vi "LCM_data_assign.vi"(9 "time-to-live":u16, 10 "Velodyne1":T2(ring), 11 "velodyne enable":bool) -> ()   [LabVIEW 2015]
uses:
  G_LCM.vi
  G_ALL.vi
  G_SEN.vi
  <vilib>/Instr/_visa.llb/VISA Configure Serial Port (Instr).vi
panel:
  out "error out 3":errorcluster
  out "velodyne overflow? 2":bool
  out "VELO_RAW":T1={"hash"=6418264790525055119, "sys time"=0, "type"=0, "raw"=""} {"hash" format="%x"}
  out "ibeo overflow?":bool
  out "veodyne error out":errorcluster
  out "control input":T3
  in  "saveconfig":bool
  in  "get data":bool
  in  "parameter idx 2":u16 format="%x"
  in  "setdata":bool
  in  "Mouting":u32 format="%x"
  in  "parameter idx":u16 format="%x"
  out "LCM error":errorcluster
  out "error out":errorcluster
  out "SDT_GPS_DATA":T4
  out "PATH_T":T5
  out "length":i32
  out "ALT_T":T6={"hash"=-8920902524919788889, "sys time"=0, "u time"=0, "alt"=0.0} {"hash" format="%016x"}
  out "value":cluster{"time":i32, "alt":sgl}
  out "data":dbl[][](array[numeric]) format="%#_17g"
  out "Waveform Graph":dbl[](graph)
  out "IBEO_2202_T":T7={"hash"=-9184050406206942030, "sys time"=0, "Header"={"Size of prev messages"=0, "Size of this messages"=8534, "Reserved"=0, "DeviceID"=0, "Data type"=8706, "NTP time"=30358766255088}, "Scan header"={"Scan number"=22632, "scanner status"=811, "Sync phase offset"=0, "Scan start time NTP"=30358508796168, "Scan end time NTP"=30358603880928, "Angle ticks per rotation"=11520, "Start angle"=0.8726646259971648, "End angle"=-0.8726646259971648, "Scan points"=849, "pos_x"=0.0, "pos_y"=0.0, "pos_h"=0.0, "Mounting position x"=3.5, "Mounting position y"=0.0, "Mounting position z"=0.45, "Reserved"=5}, "Scan points"=[{"flags"=0, "Echo"=0, "Radial distance"=20.2, "Horizontal angle"=0.8552113334772213, "Vertical angle"=-0.020943951023931952, "Echo pulse width"=92, "Reserved"=0}, {"flags"=0, "Echo"=0, "Radial distance"=20.05, "Horizontal angle"=0.8552113334772213, "Vertical angle"=-0.006981317007977317, "Echo pulse width"=48, "Reserved"=0}, {"flags"=0, "Echo"=0, "Radial distance"=20.21, "Horizontal angle"=0.8464846872172498, "Vertical angle"=-0.020943951023931952, "Echo pulse width"=80, "Reserved"=0}, {"flags"=0, "Echo"=0, "Radial distance"=20.03, "Horizontal angle"=0.8464846872172498, "Vertical angle"=-0.006981317007977317, "Echo pulse width"=120, "Reserved"=0}, {"flags"=0, "Echo"=0, "Radial distance"=20.400000000000002, "Horizontal angle"=0.8377580409572781, "Vertical angle"=-0.020943951023931952, "Echo pulse width"=136, "Reserved"=0}, {"flags"=0, "Echo"=0, "Radial distance"=20.080000000000002, "Horizontal angle"=0.8377580409572781, "Vertical angle"=-0.006981317007977317, "Echo pulse width"=132, "Reserved"=0}, {"flags"=0, "Echo"=0, "Radial distance"=20.67, "Horizontal angle"=0.8290313946973066, "Vertical angle"=-0.020943951023931952, "Echo pulse width"=124, "Reserved"=0}, {"flags"=0, "Echo"=0, "Radial distance"=20.37, "Horizontal angle"=0.8290313946973066, "Vertical angle"=-0.006981317007977317, "Echo pulse width"=144, "Reserved"=0}, {"flags"=5, "Echo"=0, "Radial distance"=20.830000000000002, "Horizontal angle"=0.8203047484373349, "Vertical angle"=-0.020943951023931952, "Echo pulse width"=72, "Reserved"=0}, {"flags"=4, "Echo"=1, "Radial distance"=21.87, "Horizontal angle"=0.8203047484373349, "Vertical angle"=-0.020943951023931952, "Echo pulse width"=124, "Reserved"=0}, {"flags"=4, "Echo"=0, "Radial distance"=21.88, "Horizontal angle"=0.8115781021773633, "Vertical angle"=-0.020943951023931952, "Echo pulse width"=132, "Reserved"=0}, {"flags"=4, "Echo"=0, "Radial distance"=21.78, "Horizontal angle"=0.8028514559173915, "Vertical angle"=-0.020943951023931952, "Echo pulse width"=156, "Reserved"=0}, {"flags"=4, "Echo"=0, "Radial distance"=21.76, "Horizontal angle"=0.7941248096574199, "Vertical angle"=-0.020943951023931952, "Echo pulse width"=176, "Reserved"=0}, {"flags"=1, "Echo"=0, "Radial distance"=23.37, "Horizontal angle"=0.7941248096574199, "Vertical angle"=-0.006981317007977317, "Echo pulse width"=100, "Reserved"=1}, {"flags"=0, "Echo"=1, "Radial distance"=48.230000000000004, "Horizontal angle"=0.7941248096574199, "Vertical angle"=-0.006981317007977317, "Echo pulse width"=120, "Reserved"=2}, {"flags"=4, "Echo"=0, "Radial distance"=21.76, "Horizontal angle"=0.7853981633974483, "Vertical angle"=-0.020943951023931952, "Echo pulse width"=172, "Reserved"=0}, {"flags"=1, "Echo"=0, "Radial distance"=23.25, "Horizontal angle"=0.7853981633974483, "Vertical angle"=-0.006981317007977317, "Echo pulse width"=144, "Reserved"=1}, {"flags"=0, "Echo"=1, "Radial distance"=48.02, "Horizontal angle"=0.7853981633974483, "Vertical angle"=-0.006981317007977317, "Echo pulse width"=108, "Reserved"=2}, {"flags"=0, "Echo"=0, "Radial distance"=16.740000000000002, "Horizontal angle"=0.7766715171374766, "Vertical angle"=-0.020943951023931952, "Echo pulse width"=156, "Reserved"=3}, {"flags"=0, "Echo"=0, "Radial distance"=16.77, "Horizontal angle"=0.7766715171374766, "Vertical angle"=-0.006981317007977317, "Echo pulse width"=152, "Reserved"=3}, {"flags"=5, "Echo"=0, "Radial distance"=5.44, "Horizontal angle"=0.767944870877505, "Vertical angle"=-0.020943951023931952, "Echo pulse width"=136, "Reserved"=0}, {"flags"=4, "Echo"=1, "Radial distance"=21.87, "Horizontal angle"=0.767944870877505, "Vertical angle"=-0.020943951023931952, "Echo pulse width"=164, "Reserved"=0}, {"flags"=1, "Echo"=0, "Radial distance"=23.17, "Horizontal angle"=0.767944870877505, "Vertical angle"=-0.006981317007977317, "Echo pulse width"=148, "Reserved"=1}, {"flags"=0, "Echo"=1, "Radial distance"=48.18, "Horizontal angle"=0.767944870877505, "Vertical angle"=-0.006981317007977317, "Echo pulse width"=108, "Reserved"=4}, {"flags"=4, "Echo"=0, "Radial distance"=22.03, "Horizontal angle"=0.7592182246175333, "Vertical angle"=-0.020943951023931952, "Echo pulse width"=164, "Reserved"=0}, {"flags"=0, "Echo"=0, "Radial distance"=23.3, "Horizontal angle"=0.7592182246175333, "Vertical angle"=-0.006981317007977317, "Echo pulse width"=168, "Reserved"=1}, {"flags"=5, "Echo"=0, "Radial distance"=5.21, "Horizontal angle"=0.7504915783575618, "Vertical angle"=-0.020943951023931952, "Echo pulse width"=144, "Reserved"=0}, {"flags"=4, "Echo"=1, "Radial distance"=22.27, "Horizontal angle"=0.7504915783575618, "Vertical angle"=-0.020943951023931952, "Echo pulse width"=164, "Reserved"=0}, {"flags"=0, "Echo"=0, "Radial distance"=23.34, "Horizontal angle"=0.7504915783575618, "Vertical angle"=-0.006981317007977317, "Echo pulse width"=172, "Reserved"=1}, {"flags"=5, "Echo"=0, "Radial distance"=20.36, "Horizontal angle"=0.74176493209759, "Vertical angle"=-0.020943951023931952, "Echo pulse width"=68, "Reserved"=0}, {"flags"=4, "Echo"=1, "Radial distance"=22.42, "Horizontal angle"=0.74176493209759, "Vertical angle"=-0.020943951023931952, "Echo pulse width"=152, "Reserved"=0}, {"flags"=0, "Echo"=0, "Radial distance"=23.38, "Horizontal angle"=0.74176493209759, "Vertical angle"=-0.006981317007977317, "Echo pulse width"=168, "Reserved"=1}, {"flags"=5, "Echo"=0, "Radial distance"=5.5600000000000005, "Horizontal angle"=0.7330382858376184, "Vertical angle"=-0.020943951023931952, "Echo pulse width"=168, "Reserved"=0}, {"flags"=4, "Echo"=1, "Radial distance"=22.62, "Horizontal angle"=0.7330382858376184, "Vertical angle"=-0.020943951023931952, "Echo pulse width"=152, "Reserved"=0}, {"flags"=1, "Echo"=0, "Radial distance"=23.37, "Horizontal angle"=0.7330382858376184, "Vertical angle"=-0.006981317007977317, "Echo pulse width"=156, "Reserved"=1}, {"flags"=0, "Echo"=1, "Radial distance"=48.21, "Horizontal angle"=0.7330382858376184, "Vertical angle"=-0.006981317007977317, "Echo pulse width"=72, "Reserved"=5}, {"flags"=5, "Echo"=0, "Radial distance"=5.58, "Horizontal angle"=0.7243116395776468, "Vertical angle"=-0.020943951023931952, "Echo pulse width"=136, "Reserved"=0}, {"flags"=5, "Echo"=1, "Radial distance"=20.88, "Horizontal angle"=0.7243116395776468, "Vertical angle"=-0.020943951023931952, "Echo pulse width"=64, "Reserved"=0}, {"flags"=4, "Echo"=2, "Radial distance"=22.77, "Horizontal angle"=0.7243116395776468, "Vertical angle"=-0.020943951023931952, "Echo pulse width"=148, "Reserved"=0}, {"flags"=0, "Echo"=0, "Radial distance"=23.62, "Horizontal angle"=0.7243116395776468, "Vertical angle"=-0.006981317007977317, "Echo pulse width"=172, "Reserved"=1}, {"flags"=5, "Echo"=0, "Radial distance"=5.63, "Horizontal angle"=0.7155849933176751, "Vertical angle"=-0.020943951023931952, "Echo pulse width"=196, "Reserved"=0}, {"flags"=4, "Echo"=1, "Radial distance"=22.69, "Horizontal angle"=0.7155849933176751, "Vertical angle"=-0.020943951023931952, "Echo pulse width"=212, "Reserved"=0}, {"flags"=0, "Echo"=0, "Radial distance"=23.82, "Horizontal angle"=0.7155849933176751, "Vertical angle"=-0.006981317007977317, "Echo pulse width"=160, "Reserved"=1}, {"flags"=5, "Echo"=0, "Radial distance"=5.67, "Horizontal angle"=0.7068583470577035, "Vertical angle"=-0.020943951023931952, "Echo pulse width"=172, "Reserved"=0}, {"flags"=4, "Echo"=1, "Radial distance"=23.16, "Horizontal angle"=0.7068583470577035, "Vertical angle"=-0.020943951023931952, "Echo pulse width"=176, "Reserved"=0}, {"flags"=0, "Echo"=0, "Radial distance"=23.62, "Horizontal angle"=0.7068583470577035, "Vertical angle"=-0.006981317007977317, "Echo pulse width"=164, "Reserved"=1}, {"flags"=5, "Echo"=0, "Radial distance"=5.53, "Horizontal angle"=0.6981317007977318, "Vertical angle"=-0.020943951023931952, "Echo pulse width"=208, "Reserved"=0}, {"flags"=0, "Echo"=1, "Radial distance"=23.35, "Horizontal angle"=0.6981317007977318, "Vertical angle"=-0.020943951023931952, "Echo pulse width"=160, "Reserved"=1}, {"flags"=0, "Echo"=0, "Radial distance"=23.650000000000002, "Horizontal angle"=0.6981317007977318, "Vertical angle"=-0.006981317007977317, "Echo pulse width"=148, "Reserved"=1}, {"flags"=5, "Echo"=0, "Radial distance"=5.55, "Horizontal angle"=0.6894050545377601, "Vertical angle"=-0.020943951023931952, "Echo pulse width"=192, "Reserved"=0}, {"flags"=0, "Echo"=1, "Radial distance"=23.55, "Horizontal angle"=0.6894050545377601, "Vertical angle"=-0.020943951023931952, "Echo pulse width"=160, "Reserved"=1}, {"flags"=0, "Echo"=0, "Radial distance"=23.62, "Horizontal angle"=0.6894050545377601, "Vertical angle"=-0.006981317007977317, "Echo pulse width"=160, "Reserved"=1}, {"flags"=5, "Echo"=0, "Radial distance"=5.5600000000000005, "Horizontal angle"=0.6806784082777886, "Vertical angle"=-0.020943951023931952, "Echo pulse width"=236, "Reserved"=0}, {"flags"=0, "Echo"=1, "Radial distance"=23.77, "Horizontal angle"=0.6806784082777886, "Vertical angle"=-0.020943951023931952, "Echo pulse width"=144, "Reserved"=1}, {"flags"=0, "Echo"=0, "Radial distance"=23.61, "Horizontal angle"=0.6806784082777886, "Vertical angle"=-0.006981317007977317, "Echo pulse width"=156, "Reserved"=1}, {"flags"=5, "Echo"=0, "Radial distance"=5.5200000000000005, "Horizontal angle"=0.6719517620178168, "Vertical angle"=-0.020943951023931952, "Echo pulse width"=220, "Reserved"=0}, {"flags"=4, "Echo"=1, "Radial distance"=24.17, "Horizontal angle"=0.6719517620178168, "Vertical angle"=-0.020943951023931952, "Echo pulse width"=148, "Reserved"=0}, {"flags"=0, "Echo"=0, "Radial distance"=23.66, "Horizontal angle"=0.6719517620178168, "Vertical angle"=-0.006981317007977317, "Echo pulse width"=164, "Reserved"=1}, {"flags"=5, "Echo"=0, "Radial distance"=5.67, "Horizontal angle"=0.6632251157578453, "Vertical angle"=-0.020943951023931952, "Echo pulse width"=224, "Reserved"=0}, {"flags"=4, "Echo"=1, "Radial distance"=24.45, "Horizontal angle"=0.6632251157578453, "Vertical angle"=-0.020943951023931952, "Echo pulse width"=148, "Reserved"=0}, {"flags"=1, "Echo"=0, "Radial distance"=32.230000000000004, "Horizontal angle"=0.6632251157578453, "Vertical angle"=-0.006981317007977317, "Echo pulse width"=40, "Reserved"=6}, {"flags"=0, "Echo"=1, "Radial distance"=35.42, "Horizontal angle"=0.6632251157578453, "Vertical angle"=-0.006981317007977317, "Echo pulse width"=164, "Reserved"=7}, {"flags"=5, "Echo"=0, "Radial distance"=5.63, "Horizontal angle"=0.6544984694978736, "Vertical angle"=-0.020943951023931952, "Echo pulse width"=208, "Reserved"=0}, {"flags"=4, "Echo"=1, "Radial distance"=24.73, "Horizontal angle"=0.6544984694978736, "Vertical angle"=-0.020943951023931952, "Echo pulse width"=144, "Reserved"=0}, {"flags"=0, "Echo"=0, "Radial distance"=35.14, "Horizontal angle"=0.6544984694978736, "Vertical angle"=-0.006981317007977317, "Echo pulse width"=164, "Reserved"=7}, {"flags"=5, "Echo"=0, "Radial distance"=5.64, "Horizontal angle"=0.6457718232379019, "Vertical angle"=-0.020943951023931952, "Echo pulse width"=244, "Reserved"=0}, {"flags"=4, "Echo"=1, "Radial distance"=25.04, "Horizontal angle"=0.6457718232379019, "Vertical angle"=-0.020943951023931952, "Echo pulse width"=132, "Reserved"=0}, {"flags"=0, "Echo"=0, "Radial distance"=35.01, "Horizontal angle"=0.6457718232379019, "Vertical angle"=-0.006981317007977317, "Echo pulse width"=156, "Reserved"=7}, {"flags"=5, "Echo"=0, "Radial distance"=5.71, "Horizontal angle"=0.6370451769779303, "Vertical angle"=-0.020943951023931952, "Echo pulse width"=264, "Reserved"=0}, {"flags"=4, "Echo"=1, "Radial distance"=25.6, "Horizontal angle"=0.6370451769779303, "Vertical angle"=-0.020943951023931952, "Echo pulse width"=132, "Reserved"=0}, {"flags"=1, "Echo"=0, "Radial distance"=32.68, "Horizontal angle"=0.6370451769779303, "Vertical angle"=-0.006981317007977317, "Echo pulse width"=56, "Reserved"=8}, {"flags"=0, "Echo"=1, "Radial distance"=34.86, "Horizontal angle"=0.6370451769779303, "Vertical angle"=-0.006981317007977317, "Echo pulse width"=160, "Reserved"=7}, {"flags"=5, "Echo"=0, "Radial distance"=5.63, "Horizontal angle"=0.6283185307179586, "Vertical angle"=-0.020943951023931952, "Echo pulse width"=296, "Reserved"=0}, {"flags"=4, "Echo"=1, "Radial distance"=25.84, "Horizontal angle"=0.6283185307179586, "Vertical angle"=-0.020943951023931952, "Echo pulse width"=92, "Reserved"=0}, {"flags"=5, "Echo"=0, "Radial distance"=7.54, "Horizontal angle"=0.6283185307179586, "Vertical angle"=-0.006981317007977317, "Echo pulse width"=168, "Reserved"=0}, {"flags"=0, "Echo"=1, "Radial distance"=34.87, "Horizontal angle"=0.6283185307179586, "Vertical angle"=-0.006981317007977317, "Echo pulse width"=124, "Reserved"=7}, {"flags"=4, "Echo"=0, "Radial distance"=5.67, "Horizontal angle"=0.619591884457987, "Vertical angle"=-0.020943951023931952, "Echo pulse width"=272, "Reserved"=0}, {"flags"=4, "Echo"=0, "Radial distance"=7.38, "Horizontal angle"=0.619591884457987, "Vertical angle"=-0.006981317007977317, "Echo pulse width"=204, "Reserved"=0}, {"flags"=4, "Echo"=0, "Radial distance"=5.67, "Horizontal angle"=0.6108652381980153, "Vertical angle"=-0.020943951023931952, "Echo pulse width"=284, "Reserved"=0}, {"flags"=0, "Echo"=0, "Radial distance"=7.33, "Horizontal angle"=0.6108652381980153, "Vertical angle"=-0.006981317007977317, "Echo pulse width"=224, "Reserved"=9}, {"flags"=0, "Echo"=0, "Radial distance"=7.21, "Horizontal angle"=0.6065019150680295, "Vertical angle"=0.00698131700797732, "Echo pulse width"=124, "Reserved"=9}, {"flags"=0, "Echo"=0, "Radial distance"=7.08, "Horizontal angle"=0.6065019150680295, "Vertical angle"=0.020943951023931963, "Echo pulse width"=120, "Reserved"=9}, {"flags"=4, "Echo"=0, "Radial distance"=5.79, "Horizontal angle"=0.6021385919380438, "Vertical angle"=-0.020943951023931952, "Echo pulse width"=248, "Reserved"=0}, {"flags"=0, "Echo"=0, "Radial distance"=7.09, "Horizontal angle"=0.6021385919380438, "Vertical angle"=-0.006981317007977317, "Echo pulse width"=232, "Reserved"=9}, {"flags"=0, "Echo"=0, "Radial distance"=7.24, "Horizontal angle"=0.5977752688080579, "Vertical angle"=0.00698131700797732, "Echo pulse width"=72, "Reserved"=9}, {"flags"=0, "Echo"=0, "Radial distance"=6.99, "Horizontal angle"=0.5977752688080579, "Vertical angle"=0.020943951023931963, "Echo pulse width"=60, "Reserved"=9}, {"flags"=4, "Echo"=0, "Radial distance"=5.75, "Horizontal angle"=0.593411945678072, "Vertical angle"=-0.020943951023931952, "Echo pulse width"=268, "Reserved"=0}, {"flags"=0, "Echo"=0, "Radial distance"=6.84, "Horizontal angle"=0.593411945678072, "Vertical angle"=-0.006981317007977317, "Echo pulse width"=284, "Reserved"=9}, {"flags"=0, "Echo"=0, "Radial distance"=7.140000000000001, "Horizontal angle"=0.5890486225480862, "Vertical angle"=0.00698131700797732, "Echo pulse width"=160, "Reserved"=9}, {"flags"=0, "Echo"=0, "Radial distance"=6.98, "Horizontal angle"=0.5890486225480862, "Vertical angle"=0.020943951023931963, "Echo pulse width"=144, "Reserved"=9}, {"flags"=4, "Echo"=0, "Radial distance"=5.79, "Horizontal angle"=0.5846852994181004, "Vertical angle"=-0.020943951023931952, "Echo pulse width"=236, "Reserved"=0}, {"flags"=0, "Echo"=0, "Radial distance"=6.95, "Horizontal angle"=0.5846852994181004, "Vertical angle"=-0.006981317007977317, "Echo pulse width"=264, "Reserved"=9}, {"flags"=0, "Echo"=0, "Radial distance"=7.03, "Horizontal angle"=0.5803219762881145, "Vertical angle"=0.00698131700797732, "Echo pulse width"=112, "Reserved"=9}, {"flags"=0, "Echo"=0, "Radial distance"=6.8, "Horizontal angle"=0.5803219762881145, "Vertical angle"=0.020943951023931963, "Echo pulse width"=104, "Reserved"=9}, {"flags"=4, "Echo"=0, "Radial distance"=5.67, "Horizontal angle"=0.5759586531581287, "Vertical angle"=-0.020943951023931952, "Echo pulse width"=268, "Reserved"=0}, {"flags"=0, "Echo"=0, "Radial distance"=6.76, "Horizontal angle"=0.5759586531581287, "Vertical angle"=-0.006981317007977317, "Echo pulse width"=288, "Reserved"=9}, {"flags"=0, "Echo"=0, "Radial distance"=7.0200000000000005, "Horizontal angle"=0.5715953300281429, "Vertical angle"=0.00698131700797732, "Echo pulse width"=168, "Reserved"=9}, {"flags"=0, "Echo"=0, "Radial distance"=6.91, "Horizontal angle"=0.5715953300281429, "Vertical angle"=0.020943951023931963, "Echo pulse width"=156, "Reserved"=9}, {"flags"=4, "Echo"=0, "Radial distance"=5.76, "Horizontal angle"=0.5672320068981571, "Vertical angle"=-0.020943951023931952, "Echo pulse width"=216, "Reserved"=0}, {"flags"=0, "Echo"=0, "Radial distance"=6.71, "Horizontal angle"=0.5672320068981571, "Vertical angle"=-0.006981317007977317, "Echo pulse width"=264, "Reserved"=9}, {"flags"=0, "Echo"=0, "Radial distance"=7.08, "Horizontal angle"=0.5628686837681712, "Vertical angle"=0.00698131700797732, "Echo pulse width"=136, "Reserved"=9}, {"flags"=0, "Echo"=0, "Radial distance"=6.8100000000000005, "Horizontal angle"=0.5628686837681712, "Vertical angle"=0.020943951023931963, "Echo pulse width"=112, "Reserved"=9}, {"flags"=4, "Echo"=0, "Radial distance"=5.79, "Horizontal angle"=0.5585053606381855, "Vertical angle"=-0.020943951023931952, "Echo pulse width"=248, "Reserved"=0}, {"flags"=0, "Echo"=0, "Radial distance"=6.6000000000000005, "Horizontal angle"=0.5585053606381855, "Vertical angle"=-0.006981317007977317, "Echo pulse width"=256, "Reserved"=9}, {"flags"=0, "Echo"=0, "Radial distance"=6.95, "Horizontal angle"=0.5541420375081997, "Vertical angle"=0.00698131700797732, "Echo pulse width"=176, "Reserved"=9}, {"flags"=0, "Echo"=0, "Radial distance"=6.75, "Horizontal angle"=0.5541420375081997, "Vertical angle"=0.020943951023931963, "Echo pulse width"=160, "Reserved"=9}, {"flags"=4, "Echo"=0, "Radial distance"=5.8100000000000005, "Horizontal angle"=0.5497787143782138, "Vertical angle"=-0.020943951023931952, "Echo pulse width"=204, "Reserved"=0}, {"flags"=0, "Echo"=0, "Radial distance"=6.61, "Horizontal angle"=0.5497787143782138, "Vertical angle"=-0.006981317007977317, "Echo pulse width"=224, "Reserved"=9}, {"flags"=0, "Echo"=0, "Radial distance"=6.88, "Horizontal angle"=0.5454153912482279, "Vertical angle"=0.00698131700797732, "Echo pulse width"=140, "Reserved"=9}, {"flags"=0, "Echo"=0, "Radial distance"=6.65, "Horizontal angle"=0.5454153912482279, "Vertical angle"=0.020943951023931963, "Echo pulse width"=124, "Reserved"=9}, {"flags"=4, "Echo"=0, "Radial distance"=5.8, "Horizontal angle"=0.5410520681182421, "Vertical angle"=-0.020943951023931952, "Echo pulse width"=232, "Reserved"=0}, {"flags"=0, "Echo"=0, "Radial distance"=6.65, "Horizontal angle"=0.5410520681182421, "Vertical angle"=-0.006981317007977317, "Echo pulse width"=232, "Reserved"=9}, {"flags"=0, "Echo"=0, "Radial distance"=6.91, "Horizontal angle"=0.5366887449882564, "Vertical angle"=0.00698131700797732, "Echo pulse width"=192, "Reserved"=9}, {"flags"=0, "Echo"=0, "Radial distance"=6.67, "Horizontal angle"=0.5366887449882564, "Vertical angle"=0.020943951023931963, "Echo pulse width"=160, "Reserved"=9}, {"flags"=4, "Echo"=0, "Radial distance"=5.91, "Horizontal angle"=0.5323254218582705, "Vertical angle"=-0.020943951023931952, "Echo pulse width"=196, "Reserved"=0}, {"flags"=0, "Echo"=0, "Radial distance"=6.7, "Horizontal angle"=0.5323254218582705, "Vertical angle"=-0.006981317007977317, "Echo pulse width"=200, "Reserved"=9}, {"flags"=0, "Echo"=0, "Radial distance"=6.72, "Horizontal angle"=0.5279620987282847, "Vertical angle"=0.00698131700797732, "Echo pulse width"=136, "Reserved"=9}, {"flags"=0, "Echo"=0, "Radial distance"=6.66, "Horizontal angle"=0.5279620987282847, "Vertical angle"=0.020943951023931963, "Echo pulse width"=144, "Reserved"=9}, {"flags"=4, "Echo"=0, "Radial distance"=5.91, "Horizontal angle"=0.5235987755982988, "Vertical angle"=-0.020943951023931952, "Echo pulse width"=224, "Reserved"=0}, {"flags"=0, "Echo"=0, "Radial distance"=6.72, "Horizontal angle"=0.5235987755982988, "Vertical angle"=-0.006981317007977317, "Echo pulse width"=220, "Reserved"=9}, {"flags"=0, "Echo"=0, "Radial distance"=6.87, "Horizontal angle"=0.519235452468313, "Vertical angle"=0.00698131700797732, "Echo pulse width"=180, "Reserved"=9}, {"flags"=0, "Echo"=0, "Radial distance"=6.68, "Horizontal angle"=0.519235452468313, "Vertical angle"=0.020943951023931963, "Echo pulse width"=180, "Reserved"=9}, {"flags"=4, "Echo"=0, "Radial distance"=6.03, "Horizontal angle"=0.5148721293383272, "Vertical angle"=-0.020943951023931952, "Echo pulse width"=192, "Reserved"=0}, {"flags"=0, "Echo"=0, "Radial distance"=6.68, "Horizontal angle"=0.5148721293383272, "Vertical angle"=-0.006981317007977317, "Echo pulse width"=208, "Reserved"=9}, {"flags"=0, "Echo"=0, "Radial distance"=7.01, "Horizontal angle"=0.5105088062083414, "Vertical angle"=0.00698131700797732, "Echo pulse width"=176, "Reserved"=9}, {"flags"=0, "Echo"=0, "Radial distance"=6.62, "Horizontal angle"=0.5105088062083414, "Vertical angle"=0.020943951023931963, "Echo pulse width"=148, "Reserved"=9}, {"flags"=4, "Echo"=0, "Radial distance"=5.99, "Horizontal angle"=0.5061454830783556, "Vertical angle"=-0.020943951023931952, "Echo pulse width"=216, "Reserved"=0}, {"flags"=0, "Echo"=0, "Radial distance"=6.6000000000000005, "Horizontal angle"=0.5061454830783556, "Vertical angle"=-0.006981317007977317, "Echo pulse width"=220, "Reserved"=9}, {"flags"=0, "Echo"=0, "Radial distance"=6.82, "Horizontal angle"=0.5017821599483697, "Vertical angle"=0.00698131700797732, "Echo pulse width"=200, "Reserved"=9}, {"flags"=0, "Echo"=0, "Radial distance"=6.640000000000001, "Horizontal angle"=0.5017821599483697, "Vertical angle"=0.020943951023931963, "Echo pulse width"=180, "Reserved"=9}, {"flags"=4, "Echo"=0, "Radial distance"=6.09, "Horizontal angle"=0.4974188368183839, "Vertical angle"=-0.020943951023931952, "Echo pulse width"=188, "Reserved"=0}, {"flags"=0, "Echo"=0, "Radial distance"=6.66, "Horizontal angle"=0.4974188368183839, "Vertical angle"=-0.006981317007977317, "Echo pulse width"=204, "Reserved"=9}, {"flags"=0, "Echo"=0, "Radial distance"=6.79, "Horizontal angle"=0.49305551368839806, "Vertical angle"=0.00698131700797732, "Echo pulse width"=160, "Reserved"=9}, {"flags"=0, "Echo"=0, "Radial distance"=6.59, "Horizontal angle"=0.49305551368839806, "Vertical angle"=0.020943951023931963, "Echo pulse width"=160, "Reserved"=9}, {"flags"=4, "Echo"=0, "Radial distance"=6.15, "Horizontal angle"=0.4886921905584123, "Vertical angle"=-0.020943951023931952, "Echo pulse width"=216, "Reserved"=0}, {"flags"=0, "Echo"=0, "Radial distance"=6.71, "Horizontal angle"=0.4886921905584123, "Vertical angle"=-0.006981317007977317, "Echo pulse width"=200, "Reserved"=9}, {"flags"=0, "Echo"=0, "Radial distance"=6.6000000000000005, "Horizontal angle"=0.48432886742842646, "Vertical angle"=0.00698131700797732, "Echo pulse width"=184, "Reserved"=9}, {"flags"=0, "Echo"=0, "Radial distance"=6.5200000000000005, "Horizontal angle"=0.48432886742842646, "Vertical angle"=0.020943951023931963, "Echo pulse width"=176, "Reserved"=9}, {"flags"=4, "Echo"=0, "Radial distance"=6.15, "Horizontal angle"=0.4799655442984406, "Vertical angle"=-0.020943951023931952, "Echo pulse width"=196, "Reserved"=0}, {"flags"=0, "Echo"=0, "Radial distance"=6.72, "Horizontal angle"=0.4799655442984406, "Vertical angle"=-0.006981317007977317, "Echo pulse width"=184, "Reserved"=9}, {"flags"=0, "Echo"=0, "Radial distance"=6.71, "Horizontal angle"=0.47560222116845474, "Vertical angle"=0.00698131700797732, "Echo pulse width"=184, "Reserved"=9}, {"flags"=0, "Echo"=0, "Radial distance"=6.63, "Horizontal angle"=0.47560222116845474, "Vertical angle"=0.020943951023931963, "Echo pulse width"=168, "Reserved"=9}, {"flags"=4, "Echo"=0, "Radial distance"=6.15, "Horizontal angle"=0.47123889803846897, "Vertical angle"=-0.020943951023931952, "Echo pulse width"=224, "Reserved"=0}, {"flags"=0, "Echo"=0, "Radial distance"=6.68, "Horizontal angle"=0.47123889803846897, "Vertical angle"=-0.006981317007977317, "Echo pulse width"=196, "Reserved"=9}, {"flags"=0, "Echo"=0, "Radial distance"=6.6000000000000005, "Horizontal angle"=0.46687557490848314, "Vertical angle"=0.00698131700797732, "Echo pulse width"=188, "Reserved"=9}, {"flags"=0, "Echo"=0, "Radial distance"=6.6000000000000005, "Horizontal angle"=0.46687557490848314, "Vertical angle"=0.020943951023931963, "Echo pulse width"=196, "Reserved"=9}, {"flags"=4, "Echo"=0, "Radial distance"=6.13, "Horizontal angle"=0.4625122517784973, "Vertical angle"=-0.020943951023931952, "Echo pulse width"=204, "Reserved"=0}, {"flags"=0, "Echo"=0, "Radial distance"=6.63, "Horizontal angle"=0.4625122517784973, "Vertical angle"=-0.006981317007977317, "Echo pulse width"=192, "Reserved"=9}, {"flags"=0, "Echo"=0, "Radial distance"=6.57, "Horizontal angle"=0.45814892864851153, "Vertical angle"=0.00698131700797732, "Echo pulse width"=172, "Reserved"=9}, {"flags"=0, "Echo"=0, "Radial distance"=6.63, "Horizontal angle"=0.45814892864851153, "Vertical angle"=0.020943951023931963, "Echo pulse width"=180, "Reserved"=9}, {"flags"=4, "Echo"=0, "Radial distance"=6.3100000000000005, "Horizontal angle"=0.45378560551852565, "Vertical angle"=-0.020943951023931952, "Echo pulse width"=220, "Reserved"=0}, {"flags"=0, "Echo"=0, "Radial distance"=6.67, "Horizontal angle"=0.45378560551852565, "Vertical angle"=-0.006981317007977317, "Echo pulse width"=200, "Reserved"=9}, {"flags"=0, "Echo"=0, "Radial distance"=6.63, "Horizontal angle"=0.4494222823885398, "Vertical angle"=0.00698131700797732, "Echo pulse width"=192, "Reserved"=9}, {"flags"=0, "Echo"=0, "Radial distance"=6.49, "Horizontal angle"=0.4494222823885398, "Vertical angle"=0.020943951023931963, "Echo pulse width"=184, "Reserved"=9}, {"flags"=4, "Echo"=0, "Radial distance"=6.2700000000000005, "Horizontal angle"=0.445058959258554, "Vertical angle"=-0.020943951023931952, "Echo pulse width"=196, "Reserved"=0}, {"flags"=0, "Echo"=0, "Radial distance"=6.59, "Horizontal angle"=0.445058959258554, "Vertical angle"=-0.006981317007977317, "Echo pulse width"=196, "Reserved"=9}, {"flags"=0, "Echo"=0, "Radial distance"=6.53, "Horizontal angle"=0.4406956361285682, "Vertical angle"=0.00698131700797732, "Echo pulse width"=172, "Reserved"=9}, {"flags"=0, "Echo"=0, "Radial distance"=6.51, "Horizontal angle"=0.4406956361285682, "Vertical angle"=0.020943951023931963, "Echo pulse width"=172, "Reserved"=9}, {"flags"=4, "Echo"=0, "Radial distance"=6.3500000000000005, "Horizontal angle"=0.4363323129985824, "Vertical angle"=-0.020943951023931952, "Echo pulse width"=220, "Reserved"=0}, {"flags"=0, "Echo"=0, "Radial distance"=6.67, "Horizontal angle"=0.4363323129985824, "Vertical angle"=-0.006981317007977317, "Echo pulse width"=204, "Reserved"=9}, {"flags"=0, "Echo"=0, "Radial distance"=6.5600000000000005, "Horizontal angle"=0.4319689898685966, "Vertical angle"=0.00698131700797732, "Echo pulse width"=188, "Reserved"=9}, {"flags"=0, "Echo"=0, "Radial distance"=6.5200000000000005, "Horizontal angle"=0.4319689898685966, "Vertical angle"=0.020943951023931963, "Echo pulse width"=192, "Reserved"=9}, {"flags"=0, "Echo"=0, "Radial distance"=6.390000000000001, "Horizontal angle"=0.42760566673861067, "Vertical angle"=-0.020943951023931952, "Echo pulse width"=192, "Reserved"=9}, {"flags"=0, "Echo"=0, "Radial distance"=6.71, "Horizontal angle"=0.42760566673861067, "Vertical angle"=-0.006981317007977317, "Echo pulse width"=192, "Reserved"=9}, {"flags"=0, "Echo"=0, "Radial distance"=6.49, "Horizontal angle"=0.4232423436086249, "Vertical angle"=0.00698131700797732, "Echo pulse width"=168, "Reserved"=9}, {"flags"=0, "Echo"=0, "Radial distance"=6.51, "Horizontal angle"=0.4232423436086249, "Vertical angle"=0.020943951023931963, "Echo pulse width"=168, "Reserved"=9}, {"flags"=0, "Echo"=0, "Radial distance"=6.41, "Horizontal angle"=0.41887902047863906, "Vertical angle"=-0.020943951023931952, "Echo pulse width"=212, "Reserved"=9}, {"flags"=0, "Echo"=0, "Radial distance"=6.76, "Horizontal angle"=0.41887902047863906, "Vertical angle"=-0.006981317007977317, "Echo pulse width"=216, "Reserved"=9}, {"flags"=0, "Echo"=0, "Radial distance"=6.66, "Horizontal angle"=0.4145156973486533, "Vertical angle"=0.00698131700797732, "Echo pulse width"=204, "Reserved"=9}, {"flags"=0, "Echo"=0, "Radial distance"=6.49, "Horizontal angle"=0.4145156973486533, "Vertical angle"=0.020943951023931963, "Echo pulse width"=188, "Reserved"=9}, {"flags"=0, "Echo"=0, "Radial distance"=6.47, "Horizontal angle"=0.41015237421866746, "Vertical angle"=-0.020943951023931952, "Echo pulse width"=180, "Reserved"=9}, {"flags"=0, "Echo"=0, "Radial distance"=6.71, "Horizontal angle"=0.41015237421866746, "Vertical angle"=-0.006981317007977317, "Echo pulse width"=192, "Reserved"=9}, {"flags"=0, "Echo"=0, "Radial distance"=6.69, "Horizontal angle"=0.40578905108868163, "Vertical angle"=0.00698131700797732, "Echo pulse width"=176, "Reserved"=9}, {"flags"=0, "Echo"=0, "Radial distance"=6.51, "Horizontal angle"=0.40578905108868163, "Vertical angle"=0.020943951023931963, "Echo pulse width"=176, "Reserved"=9}, {"flags"=0, "Echo"=0, "Radial distance"=6.53, "Horizontal angle"=0.40142572795869574, "Vertical angle"=-0.020943951023931952, "Echo pulse width"=208, "Reserved"=9}, {"flags"=0, "Echo"=0, "Radial distance"=6.71, "Horizontal angle"=0.40142572795869574, "Vertical angle"=-0.006981317007977317, "Echo pulse width"=200, "Reserved"=9}, {"flags"=0, "Echo"=0, "Radial distance"=6.79, "Horizontal angle"=0.39706240482870997, "Vertical angle"=0.00698131700797732, "Echo pulse width"=220, "Reserved"=9}, {"flags"=0, "Echo"=0, "Radial distance"=6.72, "Horizontal angle"=0.39706240482870997, "Vertical angle"=0.020943951023931963, "Echo pulse width"=220, "Reserved"=9}, {"flags"=0, "Echo"=0, "Radial distance"=6.61, "Horizontal angle"=0.39269908169872414, "Vertical angle"=-0.020943951023931952, "Echo pulse width"=184, "Reserved"=9}, {"flags"=0, "Echo"=0, "Radial distance"=6.74, "Horizontal angle"=0.39269908169872414, "Vertical angle"=-0.006981317007977317, "Echo pulse width"=176, "Reserved"=9}, {"flags"=0, "Echo"=0, "Radial distance"=6.69, "Horizontal angle"=0.3883357585687383, "Vertical angle"=0.00698131700797732, "Echo pulse width"=172, "Reserved"=9}, {"flags"=0, "Echo"=0, "Radial distance"=6.59, "Horizontal angle"=0.3883357585687383, "Vertical angle"=0.020943951023931963, "Echo pulse width"=160, "Reserved"=9}, {"flags"=0, "Echo"=0, "Radial distance"=6.63, "Horizontal angle"=0.3839724354387525, "Vertical angle"=-0.020943951023931952, "Echo pulse width"=216, "Reserved"=9}, {"flags"=0, "Echo"=0, "Radial distance"=6.74, "Horizontal angle"=0.3839724354387525, "Vertical angle"=-0.006981317007977317, "Echo pulse width"=208, "Reserved"=9}, {"flags"=0, "Echo"=0, "Radial distance"=6.84, "Horizontal angle"=0.37960911230876665, "Vertical angle"=0.00698131700797732, "Echo pulse width"=208, "Reserved"=9}, {"flags"=0, "Echo"=0, "Radial distance"=6.640000000000001, "Horizontal angle"=0.37960911230876665, "Vertical angle"=0.020943951023931963, "Echo pulse width"=200, "Reserved"=9}, {"flags"=0, "Echo"=0, "Radial distance"=6.67, "Horizontal angle"=0.3752457891787809, "Vertical angle"=-0.020943951023931952, "Echo pulse width"=180, "Reserved"=9}, {"flags"=0, "Echo"=0, "Radial distance"=6.67, "Horizontal angle"=0.3752457891787809, "Vertical angle"=-0.006981317007977317, "Echo pulse width"=196, "Reserved"=9}, {"flags"=0, "Echo"=0, "Radial distance"=6.69, "Horizontal angle"=0.370882466048795, "Vertical angle"=0.00698131700797732, "Echo pulse width"=172, "Reserved"=9}, {"flags"=0, "Echo"=0, "Radial distance"=6.67, "Horizontal angle"=0.370882466048795, "Vertical angle"=0.020943951023931963, "Echo pulse width"=172, "Reserved"=9}, {"flags"=0, "Echo"=0, "Radial distance"=6.84, "Horizontal angle"=0.3665191429188092, "Vertical angle"=-0.020943951023931952, "Echo pulse width"=236, "Reserved"=9}, {"flags"=0, "Echo"=0, "Radial distance"=6.84, "Horizontal angle"=0.3665191429188092, "Vertical angle"=-0.006981317007977317, "Echo pulse width"=276, "Reserved"=9}, {"flags"=0, "Echo"=0, "Radial distance"=6.95, "Horizontal angle"=0.3621558197888234, "Vertical angle"=0.00698131700797732, "Echo pulse width"=220, "Reserved"=9}, {"flags"=0, "Echo"=0, "Radial distance"=6.76, "Horizontal angle"=0.3621558197888234, "Vertical angle"=0.020943951023931963, "Echo pulse width"=196, "Reserved"=9}, {"flags"=0, "Echo"=0, "Radial distance"=6.87, "Horizontal angle"=0.35779249665883756, "Vertical angle"=-0.020943951023931952, "Echo pulse width"=192, "Reserved"=9}, {"flags"=0, "Echo"=0, "Radial distance"=7.05, "Horizontal angle"=0.35779249665883756, "Vertical angle"=-0.006981317007977317, "Echo pulse width"=236, "Reserved"=9}, {"flags"=0, "Echo"=0, "Radial distance"=6.8100000000000005, "Horizontal angle"=0.3534291735288517, "Vertical angle"=0.00698131700797732, "Echo pulse width"=168, "Reserved"=9}, {"flags"=0, "Echo"=0, "Radial distance"=6.79, "Horizontal angle"=0.3534291735288517, "Vertical angle"=0.020943951023931963, "Echo pulse width"=168, "Reserved"=9}, {"flags"=0, "Echo"=0, "Radial distance"=6.95, "Horizontal angle"=0.3490658503988659, "Vertical angle"=-0.020943951023931952, "Echo pulse width"=192, "Reserved"=9}, {"flags"=0, "Echo"=0, "Radial distance"=7.04, "Horizontal angle"=0.3490658503988659, "Vertical angle"=-0.006981317007977317, "Echo pulse width"=284, "Reserved"=9}, {"flags"=0, "Echo"=0, "Radial distance"=7.07, "Horizontal angle"=0.34470252726888007, "Vertical angle"=0.00698131700797732, "Echo pulse width"=252, "Reserved"=9}, {"flags"=0, "Echo"=0, "Radial distance"=6.98, "Horizontal angle"=0.34470252726888007, "Vertical angle"=0.020943951023931963, "Echo pulse width"=212, "Reserved"=9}, {"flags"=0, "Echo"=0, "Radial distance"=7.11, "Horizontal angle"=0.3403392041388943, "Vertical angle"=-0.020943951023931952, "Echo pulse width"=176, "Reserved"=9}, {"flags"=0, "Echo"=0, "Radial distance"=7.140000000000001, "Horizontal angle"=0.3403392041388943, "Vertical angle"=-0.006981317007977317, "Echo pulse width"=252, "Reserved"=9}, {"flags"=0, "Echo"=0, "Radial distance"=7.0200000000000005, "Horizontal angle"=0.3359758810089084, "Vertical angle"=0.00698131700797732, "Echo pulse width"=196, "Reserved"=9}, {"flags"=0, "Echo"=0, "Radial distance"=6.95, "Horizontal angle"=0.3359758810089084, "Vertical angle"=0.020943951023931963, "Echo pulse width"=176, "Reserved"=9}, {"flags"=0, "Echo"=0, "Radial distance"=7.23, "Horizontal angle"=0.33161255787892263, "Vertical angle"=-0.020943951023931952, "Echo pulse width"=268, "Reserved"=9}, {"flags"=0, "Echo"=0, "Radial distance"=7.28, "Horizontal angle"=0.33161255787892263, "Vertical angle"=-0.006981317007977317, "Echo pulse width"=284, "Reserved"=9}, {"flags"=0, "Echo"=0, "Radial distance"=7.2700000000000005, "Horizontal angle"=0.3272492347489368, "Vertical angle"=0.00698131700797732, "Echo pulse width"=276, "Reserved"=9}, {"flags"=0, "Echo"=0, "Radial distance"=7.16, "Horizontal angle"=0.3272492347489368, "Vertical angle"=0.020943951023931963, "Echo pulse width"=204, "Reserved"=9}, {"flags"=0, "Echo"=0, "Radial distance"=7.59, "Horizontal angle"=0.32288591161895097, "Vertical angle"=-0.020943951023931952, "Echo pulse width"=232, "Reserved"=9}, {"flags"=0, "Echo"=0, "Radial distance"=7.69, "Horizontal angle"=0.32288591161895097, "Vertical angle"=-0.006981317007977317, "Echo pulse width"=232, "Reserved"=9}, {"flags"=0, "Echo"=0, "Radial distance"=7.53, "Horizontal angle"=0.31852258848896514, "Vertical angle"=0.00698131700797732, "Echo pulse width"=172, "Reserved"=9}, {"flags"=0, "Echo"=0, "Radial distance"=7.41, "Horizontal angle"=0.31852258848896514, "Vertical angle"=0.020943951023931963, "Echo pulse width"=184, "Reserved"=9}, {"flags"=0, "Echo"=0, "Radial distance"=7.3500000000000005, "Horizontal angle"=0.3141592653589793, "Vertical angle"=-0.020943951023931952, "Echo pulse width"=300, "Reserved"=9}, {"flags"=0, "Echo"=0, "Radial distance"=7.68, "Horizontal angle"=0.3141592653589793, "Vertical angle"=-0.006981317007977317, "Echo pulse width"=264, "Reserved"=9}, {"flags"=0, "Echo"=0, "Radial distance"=7.58, "Horizontal angle"=0.3097959422289935, "Vertical angle"=0.00698131700797732, "Echo pulse width"=204, "Reserved"=9}, {"flags"=0, "Echo"=0, "Radial distance"=7.48, "Horizontal angle"=0.3097959422289935, "Vertical angle"=0.020943951023931963, "Echo pulse width"=192, "Reserved"=9}, {"flags"=0, "Echo"=0, "Radial distance"=7.47, "Horizontal angle"=0.30543261909900765, "Vertical angle"=-0.020943951023931952, "Echo pulse width"=260, "Reserved"=9}, {"flags"=0, "Echo"=0, "Radial distance"=7.8100000000000005, "Horizontal angle"=0.30543261909900765, "Vertical angle"=-0.006981317007977317, "Echo pulse width"=232, "Reserved"=9}, {"flags"=0, "Echo"=0, "Radial distance"=7.63, "Horizontal angle"=0.3010692959690219, "Vertical angle"=0.00698131700797732, "Echo pulse width"=164, "Reserved"=9}, {"flags"=0, "Echo"=0, "Radial distance"=7.59, "Horizontal angle"=0.3010692959690219, "Vertical angle"=0.020943951023931963, "Echo pulse width"=172, "Reserved"=9}, {"flags"=0, "Echo"=0, "Radial distance"=7.55, "Horizontal angle"=0.296705972839036, "Vertical angle"=-0.020943951023931952, "Echo pulse width"=300, "Reserved"=9}, {"flags"=0, "Echo"=0, "Radial distance"=7.96, "Horizontal angle"=0.296705972839036, "Vertical angle"=-0.006981317007977317, "Echo pulse width"=264, "Reserved"=9}, {"flags"=0, "Echo"=0, "Radial distance"=7.97, "Horizontal angle"=0.2923426497090502, "Vertical angle"=0.00698131700797732, "Echo pulse width"=236, "Reserved"=9}, {"flags"=0, "Echo"=0, "Radial distance"=7.82, "Horizontal angle"=0.2923426497090502, "Vertical angle"=0.020943951023931963, "Echo pulse width"=212, "Reserved"=9}, {"flags"=0, "Echo"=0, "Radial distance"=8.45, "Horizontal angle"=0.28797932657906433, "Vertical angle"=-0.020943951023931952, "Echo pulse width"=204, "Reserved"=9}, {"flags"=0, "Echo"=0, "Radial distance"=8.17, "Horizontal angle"=0.28797932657906433, "Vertical angle"=-0.006981317007977317, "Echo pulse width"=236, "Reserved"=9}, {"flags"=0, "Echo"=0, "Radial distance"=8.15, "Horizontal angle"=0.28361600344907856, "Vertical angle"=0.00698131700797732, "Echo pulse width"=184, "Reserved"=9}, {"flags"=0, "Echo"=0, "Radial distance"=7.95, "Horizontal angle"=0.28361600344907856, "Vertical angle"=0.020943951023931963, "Echo pulse width"=172, "Reserved"=9}, {"flags"=0, "Echo"=0, "Radial distance"=8.56, "Horizontal angle"=0.2792526803190927, "Vertical angle"=-0.020943951023931952, "Echo pulse width"=232, "Reserved"=9}, {"flags"=0, "Echo"=0, "Radial distance"=8.4, "Horizontal angle"=0.2792526803190927, "Vertical angle"=-0.006981317007977317, "Echo pulse width"=264, "Reserved"=9}, {"flags"=0, "Echo"=0, "Radial distance"=8.23, "Horizontal angle"=0.2748893571891069, "Vertical angle"=0.00698131700797732, "Echo pulse width"=192, "Reserved"=9}, {"flags"=0, "Echo"=0, "Radial distance"=8.2, "Horizontal angle"=0.2748893571891069, "Vertical angle"=0.020943951023931963, "Echo pulse width"=192, "Reserved"=9}, {"flags"=0, "Echo"=0, "Radial distance"=8.700000000000001, "Horizontal angle"=0.27052603405912107, "Vertical angle"=-0.020943951023931952, "Echo pulse width"=224, "Reserved"=9}, {"flags"=0, "Echo"=0, "Radial distance"=8.61, "Horizontal angle"=0.27052603405912107, "Vertical angle"=-0.006981317007977317, "Echo pulse width"=220, "Reserved"=9}, {"flags"=0, "Echo"=0, "Radial distance"=8.49, "Horizontal angle"=0.26616271092913524, "Vertical angle"=0.00698131700797732, "Echo pulse width"=176, "Reserved"=9}, {"flags"=0, "Echo"=0, "Radial distance"=8.43, "Horizontal angle"=0.26616271092913524, "Vertical angle"=0.020943951023931963, "Echo pulse width"=176, "Reserved"=9}, {"flags"=0, "Echo"=0, "Radial distance"=8.71, "Horizontal angle"=0.2617993877991494, "Vertical angle"=-0.020943951023931952, "Echo pulse width"=260, "Reserved"=9}, {"flags"=0, "Echo"=0, "Radial distance"=8.700000000000001, "Horizontal angle"=0.2617993877991494, "Vertical angle"=-0.006981317007977317, "Echo pulse width"=248, "Reserved"=9}, {"flags"=0, "Echo"=0, "Radial distance"=8.71, "Horizontal angle"=0.2574360646691636, "Vertical angle"=0.00698131700797732, "Echo pulse width"=196, "Reserved"=9}, {"flags"=0, "Echo"=0, "Radial distance"=8.68, "Horizontal angle"=0.2574360646691636, "Vertical angle"=0.020943951023931963, "Echo pulse width"=216, "Reserved"=9}, {"flags"=0, "Echo"=0, "Radial distance"=9.11, "Horizontal angle"=0.2530727415391778, "Vertical angle"=-0.020943951023931952, "Echo pulse width"=208, "Reserved"=9}, {"flags"=0, "Echo"=0, "Radial distance"=8.94, "Horizontal angle"=0.2530727415391778, "Vertical angle"=-0.006981317007977317, "Echo pulse width"=200, "Reserved"=9}, {"flags"=0, "Echo"=0, "Radial distance"=8.85, "Horizontal angle"=0.24870941840919195, "Vertical angle"=0.00698131700797732, "Echo pulse width"=176, "Reserved"=9}, {"flags"=0, "Echo"=0, "Radial distance"=8.870000000000001, "Horizontal angle"=0.24870941840919195, "Vertical angle"=0.020943951023931963, "Echo pulse width"=172, "Reserved"=9}, {"flags"=0, "Echo"=0, "Radial distance"=9.19, "Horizontal angle"=0.24434609527920614, "Vertical angle"=-0.020943951023931952, "Echo pulse width"=256, "Reserved"=9}, {"flags"=0, "Echo"=0, "Radial distance"=9.36, "Horizontal angle"=0.24434609527920614, "Vertical angle"=-0.006981317007977317, "Echo pulse width"=280, "Reserved"=9}, {"flags"=0, "Echo"=0, "Radial distance"=9.24, "Horizontal angle"=0.2399827721492203, "Vertical angle"=0.00698131700797732, "Echo pulse width"=208, "Reserved"=9}, {"flags"=0, "Echo"=0, "Radial distance"=9.200000000000001, "Horizontal angle"=0.2399827721492203, "Vertical angle"=0.020943951023931963, "Echo pulse width"=204, "Reserved"=9}, {"flags"=0, "Echo"=0, "Radial distance"=9.42, "Horizontal angle"=0.23561944901923448, "Vertical angle"=-0.020943951023931952, "Echo pulse width"=224, "Reserved"=9}, {"flags"=0, "Echo"=0, "Radial distance"=9.59, "Horizontal angle"=0.23561944901923448, "Vertical angle"=-0.006981317007977317, "Echo pulse width"=264, "Reserved"=9}, {"flags"=0, "Echo"=0, "Radial distance"=9.49, "Horizontal angle"=0.23125612588924865, "Vertical angle"=0.00698131700797732, "Echo pulse width"=176, "Reserved"=9}, {"flags"=0, "Echo"=0, "Radial distance"=9.35, "Horizontal angle"=0.23125612588924865, "Vertical angle"=0.020943951023931963, "Echo pulse width"=172, "Reserved"=9}, {"flags"=0, "Echo"=0, "Radial distance"=9.67, "Horizontal angle"=0.22689280275926282, "Vertical angle"=-0.020943951023931952, "Echo pulse width"=260, "Reserved"=9}, {"flags"=0, "Echo"=0, "Radial distance"=10.0, "Horizontal angle"=0.22689280275926282, "Vertical angle"=-0.006981317007977317, "Echo pulse width"=284, "Reserved"=9}, {"flags"=0, "Echo"=0, "Radial distance"=9.91, "Horizontal angle"=0.222529479629277, "Vertical angle"=0.00698131700797732, "Echo pulse width"=248, "Reserved"=9}, {"flags"=0, "Echo"=0, "Radial distance"=9.76, "Horizontal angle"=0.222529479629277, "Vertical angle"=0.020943951023931963, "Echo pulse width"=204, "Reserved"=9}, {"flags"=0, "Echo"=0, "Radial distance"=10.02, "Horizontal angle"=0.2181661564992912, "Vertical angle"=-0.020943951023931952, "Echo pulse width"=228, "Reserved"=9}, {"flags"=0, "Echo"=0, "Radial distance"=10.35, "Horizontal angle"=0.2181661564992912, "Vertical angle"=-0.006981317007977317, "Echo pulse width"=264, "Reserved"=9}, {"flags"=0, "Echo"=0, "Radial distance"=10.17, "Horizontal angle"=0.21380283336930533, "Vertical angle"=0.00698131700797732, "Echo pulse width"=180, "Reserved"=9}, {"flags"=0, "Echo"=0, "Radial distance"=10.07, "Horizontal angle"=0.21380283336930533, "Vertical angle"=0.020943951023931963, "Echo pulse width"=176, "Reserved"=9}, {"flags"=0, "Echo"=0, "Radial distance"=9.950000000000001, "Horizontal angle"=0.20943951023931953, "Vertical angle"=-0.020943951023931952, "Echo pulse width"=288, "Reserved"=9}, {"flags"=0, "Echo"=0, "Radial distance"=10.4, "Horizontal angle"=0.20943951023931953, "Vertical angle"=-0.006981317007977317, "Echo pulse width"=316, "Reserved"=9}, {"flags"=0, "Echo"=0, "Radial distance"=10.55, "Horizontal angle"=0.20507618710933373, "Vertical angle"=0.00698131700797732, "Echo pulse width"=268, "Reserved"=9}, {"flags"=0, "Echo"=0, "Radial distance"=10.32, "Horizontal angle"=0.20507618710933373, "Vertical angle"=0.020943951023931963, "Echo pulse width"=204, "Reserved"=9}, {"flags"=0, "Echo"=0, "Radial distance"=10.44, "Horizontal angle"=0.20071286397934787, "Vertical angle"=-0.020943951023931952, "Echo pulse width"=216, "Reserved"=9}, {"flags"=0, "Echo"=0, "Radial distance"=10.75, "Horizontal angle"=0.20071286397934787, "Vertical angle"=-0.006981317007977317, "Echo pulse width"=280, "Reserved"=9}, {"flags"=0, "Echo"=0, "Radial distance"=10.85, "Horizontal angle"=0.19634954084936207, "Vertical angle"=0.00698131700797732, "Echo pulse width"=176, "Reserved"=9}, {"flags"=0, "Echo"=0, "Radial distance"=10.8, "Horizontal angle"=0.19634954084936207, "Vertical angle"=0.020943951023931963, "Echo pulse width"=192, "Reserved"=9}, {"flags"=4, "Echo"=0, "Radial distance"=10.11, "Horizontal angle"=0.19198621771937624, "Vertical angle"=-0.020943951023931952, "Echo pulse width"=324, "Reserved"=0}, {"flags"=0, "Echo"=0, "Radial distance"=11.28, "Horizontal angle"=0.19198621771937624, "Vertical angle"=-0.006981317007977317, "Echo pulse width"=260, "Reserved"=9}, {"flags"=0, "Echo"=0, "Radial distance"=11.23, "Horizontal angle"=0.18762289458939044, "Vertical angle"=0.00698131700797732, "Echo pulse width"=220, "Reserved"=9}, {"flags"=0, "Echo"=0, "Radial distance"=11.120000000000001, "Horizontal angle"=0.18762289458939044, "Vertical angle"=0.020943951023931963, "Echo pulse width"=200, "Reserved"=9}, {"flags"=4, "Echo"=0, "Radial distance"=10.43, "Horizontal angle"=0.1832595714594046, "Vertical angle"=-0.020943951023931952, "Echo pulse width"=296, "Reserved"=0}, {"flags"=0, "Echo"=0, "Radial distance"=11.39, "Horizontal angle"=0.1832595714594046, "Vertical angle"=-0.006981317007977317, "Echo pulse width"=260, "Reserved"=9}, {"flags"=0, "Echo"=0, "Radial distance"=11.370000000000001, "Horizontal angle"=0.17889624832941878, "Vertical angle"=0.00698131700797732, "Echo pulse width"=172, "Reserved"=9}, {"flags"=0, "Echo"=0, "Radial distance"=11.51, "Horizontal angle"=0.17889624832941878, "Vertical angle"=0.020943951023931963, "Echo pulse width"=176, "Reserved"=9}, {"flags"=4, "Echo"=0, "Radial distance"=10.49, "Horizontal angle"=0.17453292519943295, "Vertical angle"=-0.020943951023931952, "Echo pulse width"=372, "Reserved"=0}, {"flags"=0, "Echo"=0, "Radial distance"=11.92, "Horizontal angle"=0.17453292519943295, "Vertical angle"=-0.006981317007977317, "Echo pulse width"=296, "Reserved"=9}, {"flags"=0, "Echo"=0, "Radial distance"=11.88, "Horizontal angle"=0.17016960206944715, "Vertical angle"=0.00698131700797732, "Echo pulse width"=208, "Reserved"=9}, {"flags"=0, "Echo"=0, "Radial distance"=12.040000000000001, "Horizontal angle"=0.17016960206944715, "Vertical angle"=0.020943951023931963, "Echo pulse width"=216, "Reserved"=9}, {"flags"=4, "Echo"=0, "Radial distance"=10.950000000000001, "Horizontal angle"=0.16580627893946132, "Vertical angle"=-0.020943951023931952, "Echo pulse width"=308, "Reserved"=0}, {"flags"=0, "Echo"=0, "Radial distance"=12.5, "Horizontal angle"=0.16580627893946132, "Vertical angle"=-0.006981317007977317, "Echo pulse width"=200, "Reserved"=9}, {"flags"=0, "Echo"=0, "Radial distance"=12.41, "Horizontal angle"=0.16144295580947549, "Vertical angle"=0.00698131700797732, "Echo pulse width"=172, "Reserved"=9}, {"flags"=0, "Echo"=0, "Radial distance"=12.71, "Horizontal angle"=0.16144295580947549, "Vertical angle"=0.020943951023931963, "Echo pulse width"=180, "Reserved"=9}, {"flags"=4, "Echo"=0, "Radial distance"=11.27, "Horizontal angle"=0.15707963267948966, "Vertical angle"=-0.020943951023931952, "Echo pulse width"=312, "Reserved"=0}, {"flags"=4, "Echo"=0, "Radial distance"=13.26, "Horizontal angle"=0.15707963267948966, "Vertical angle"=-0.006981317007977317, "Echo pulse width"=244, "Reserved"=0}, {"flags"=2, "Echo"=0, "Radial distance"=13.08, "Horizontal angle"=0.15271630954950383, "Vertical angle"=0.00698131700797732, "Echo pulse width"=212, "Reserved"=0}, {"flags"=3, "Echo"=0, "Radial distance"=13.27, "Horizontal angle"=0.15271630954950383, "Vertical angle"=0.020943951023931963, "Echo pulse width"=156, "Reserved"=0}, {"flags"=0, "Echo"=1, "Radial distance"=19.92, "Horizontal angle"=0.15271630954950383, "Vertical angle"=0.020943951023931963, "Echo pulse width"=176, "Reserved"=10}, {"flags"=4, "Echo"=0, "Radial distance"=11.790000000000001, "Horizontal angle"=0.148352986419518, "Vertical angle"=-0.020943951023931952, "Echo pulse width"=264, "Reserved"=0}, {"flags"=5, "Echo"=0, "Radial distance"=13.88, "Horizontal angle"=0.148352986419518, "Vertical angle"=-0.006981317007977317, "Echo pulse width"=168, "Reserved"=0}, {"flags"=5, "Echo"=1, "Radial distance"=15.94, "Horizontal angle"=0.148352986419518, "Vertical angle"=-0.006981317007977317, "Echo pulse width"=108, "Reserved"=0}, {"flags"=4, "Echo"=2, "Radial distance"=18.05, "Horizontal angle"=0.148352986419518, "Vertical angle"=-0.006981317007977317, "Echo pulse width"=340, "Reserved"=0}, {"flags"=0, "Echo"=0, "Radial distance"=19.580000000000002, "Horizontal angle"=0.14398966328953217, "Vertical angle"=0.00698131700797732, "Echo pulse width"=204, "Reserved"=10}, {"flags"=0, "Echo"=0, "Radial distance"=19.73, "Horizontal angle"=0.14398966328953217, "Vertical angle"=0.020943951023931963, "Echo pulse width"=188, "Reserved"=10}, {"flags"=4, "Echo"=0, "Radial distance"=12.19, "Horizontal angle"=0.13962634015954636, "Vertical angle"=-0.020943951023931952, "Echo pulse width"=296, "Reserved"=0}, {"flags"=3, "Echo"=0, "Radial distance"=13.52, "Horizontal angle"=0.13962634015954636, "Vertical angle"=-0.006981317007977317, "Echo pulse width"=128, "Reserved"=0}, {"flags"=5, "Echo"=1, "Radial distance"=15.610000000000001, "Horizontal angle"=0.13962634015954636, "Vertical angle"=-0.006981317007977317, "Echo pulse width"=392, "Reserved"=0}, {"flags"=0, "Echo"=2, "Radial distance"=19.61, "Horizontal angle"=0.13962634015954636, "Vertical angle"=-0.006981317007977317, "Echo pulse width"=148, "Reserved"=10}, {"flags"=0, "Echo"=0, "Radial distance"=19.56, "Horizontal angle"=0.13526301702956053, "Vertical angle"=0.00698131700797732, "Echo pulse width"=208, "Reserved"=10}, {"flags"=0, "Echo"=0, "Radial distance"=19.76, "Horizontal angle"=0.13526301702956053, "Vertical angle"=0.020943951023931963, "Echo pulse width"=192, "Reserved"=10}, {"flags"=4, "Echo"=0, "Radial distance"=12.83, "Horizontal angle"=0.1308996938995747, "Vertical angle"=-0.020943951023931952, "Echo pulse width"=288, "Reserved"=0}, {"flags"=5, "Echo"=0, "Radial distance"=14.97, "Horizontal angle"=0.1308996938995747, "Vertical angle"=-0.006981317007977317, "Echo pulse width"=400, "Reserved"=0}, {"flags"=0, "Echo"=1, "Radial distance"=19.35, "Horizontal angle"=0.1308996938995747, "Vertical angle"=-0.006981317007977317, "Echo pulse width"=204, "Reserved"=10}, {"flags"=0, "Echo"=0, "Radial distance"=19.59, "Horizontal angle"=0.1265363707695889, "Vertical angle"=0.00698131700797732, "Echo pulse width"=196, "Reserved"=10}, {"flags"=0, "Echo"=0, "Radial distance"=19.8, "Horizontal angle"=0.1265363707695889, "Vertical angle"=0.020943951023931963, "Echo pulse width"=200, "Reserved"=10}, {"flags"=4, "Echo"=0, "Radial distance"=13.39, "Horizontal angle"=0.12217304763960307, "Vertical angle"=-0.020943951023931952, "Echo pulse width"=292, "Reserved"=0}, {"flags"=5, "Echo"=0, "Radial distance"=15.700000000000001, "Horizontal angle"=0.12217304763960307, "Vertical angle"=-0.006981317007977317, "Echo pulse width"=172, "Reserved"=0}, {"flags"=4, "Echo"=1, "Radial distance"=17.69, "Horizontal angle"=0.12217304763960307, "Vertical angle"=-0.006981317007977317, "Echo pulse width"=380, "Reserved"=0}, {"flags"=0, "Echo"=0, "Radial distance"=19.75, "Horizontal angle"=0.11780972450961724, "Vertical angle"=0.00698131700797732, "Echo pulse width"=216, "Reserved"=10}, {"flags"=0, "Echo"=0, "Radial distance"=19.84, "Horizontal angle"=0.11780972450961724, "Vertical angle"=0.020943951023931963, "Echo pulse width"=200, "Reserved"=10}, {"flags"=5, "Echo"=0, "Radial distance"=13.99, "Horizontal angle"=0.11344640137963141, "Vertical angle"=-0.020943951023931952, "Echo pulse width"=152, "Reserved"=0}, {"flags"=4, "Echo"=1, "Radial distance"=15.35, "Horizontal angle"=0.11344640137963141, "Vertical angle"=-0.020943951023931952, "Echo pulse width"=120, "Reserved"=0}, {"flags"=4, "Echo"=0, "Radial distance"=16.45, "Horizontal angle"=0.11344640137963141, "Vertical angle"=-0.006981317007977317, "Echo pulse width"=500, "Reserved"=0}, {"flags"=0, "Echo"=0, "Radial distance"=19.71, "Horizontal angle"=0.1090830782496456, "Vertical angle"=0.00698131700797732, "Echo pulse width"=196, "Reserved"=10}, {"flags"=0, "Echo"=0, "Radial distance"=20.0, "Horizontal angle"=0.1090830782496456, "Vertical angle"=0.020943951023931963, "Echo pulse width"=200, "Reserved"=10}, {"flags"=4, "Echo"=0, "Radial distance"=14.72, "Horizontal angle"=0.10471975511965977, "Vertical angle"=-0.020943951023931952, "Echo pulse width"=172, "Reserved"=0}, {"flags"=4, "Echo"=0, "Radial distance"=17.25, "Horizontal angle"=0.10471975511965977, "Vertical angle"=-0.006981317007977317, "Echo pulse width"=420, "Reserved"=0}, {"flags"=0, "Echo"=0, "Radial distance"=19.72, "Horizontal angle"=0.10035643198967394, "Vertical angle"=0.00698131700797732, "Echo pulse width"=188, "Reserved"=10}, {"flags"=1, "Echo"=0, "Radial distance"=20.2, "Horizontal angle"=0.10035643198967394, "Vertical angle"=0.020943951023931963, "Echo pulse width"=204, "Reserved"=10}, {"flags"=0, "Echo"=1, "Radial distance"=22.21, "Horizontal angle"=0.10035643198967394, "Vertical angle"=0.020943951023931963, "Echo pulse width"=20, "Reserved"=11}, {"flags"=4, "Echo"=0, "Radial distance"=15.6, "Horizontal angle"=0.09599310885968812, "Vertical angle"=-0.020943951023931952, "Echo pulse width"=172, "Reserved"=0}, {"flags"=5, "Echo"=0, "Radial distance"=17.62, "Horizontal angle"=0.09599310885968812, "Vertical angle"=-0.006981317007977317, "Echo pulse width"=164, "Reserved"=0}, {"flags"=0, "Echo"=1, "Radial distance"=19.82, "Horizontal angle"=0.09599310885968812, "Vertical angle"=-0.006981317007977317, "Echo pulse width"=208, "Reserved"=10}, {"flags"=0, "Echo"=0, "Radial distance"=19.91, "Horizontal angle"=0.0916297857297023, "Vertical angle"=0.00698131700797732, "Echo pulse width"=192, "Reserved"=10}, {"flags"=0, "Echo"=0, "Radial distance"=20.52, "Horizontal angle"=0.0916297857297023, "Vertical angle"=0.020943951023931963, "Echo pulse width"=204, "Reserved"=10}, {"flags"=4, "Echo"=0, "Radial distance"=16.31, "Horizontal angle"=0.08726646259971647, "Vertical angle"=-0.020943951023931952, "Echo pulse width"=224, "Reserved"=0}, {"flags"=4, "Echo"=0, "Radial distance"=18.650000000000002, "Horizontal angle"=0.08726646259971647, "Vertical angle"=-0.006981317007977317, "Echo pulse width"=368, "Reserved"=0}, {"flags"=4, "Echo"=0, "Radial distance"=20.92, "Horizontal angle"=0.08290313946973066, "Vertical angle"=0.00698131700797732, "Echo pulse width"=184, "Reserved"=0}, {"flags"=4, "Echo"=0, "Radial distance"=21.46, "Horizontal angle"=0.08290313946973066, "Vertical angle"=0.020943951023931963, "Echo pulse width"=212, "Reserved"=0}, {"flags"=4, "Echo"=0, "Radial distance"=15.290000000000001, "Horizontal angle"=0.07853981633974483, "Vertical angle"=-0.020943951023931952, "Echo pulse width"=436, "Reserved"=0}, {"flags"=4, "Echo"=0, "Radial distance"=18.61, "Horizontal angle"=0.07853981633974483, "Vertical angle"=-0.006981317007977317, "Echo pulse width"=508, "Reserved"=0}, {"flags"=4, "Echo"=0, "Radial distance"=22.12, "Horizontal angle"=0.074176493209759, "Vertical angle"=0.00698131700797732, "Echo pulse width"=188, "Reserved"=0}, {"flags"=4, "Echo"=0, "Radial distance"=22.64, "Horizontal angle"=0.074176493209759, "Vertical angle"=0.020943951023931963, "Echo pulse width"=220, "Reserved"=0}, {"flags"=5, "Echo"=0, "Radial distance"=15.76, "Horizontal angle"=0.06981317007977318, "Vertical angle"=-0.020943951023931952, "Echo pulse width"=232, "Reserved"=0}, {"flags"=4, "Echo"=1, "Radial distance"=18.98, "Horizontal angle"=0.06981317007977318, "Vertical angle"=-0.020943951023931952, "Echo pulse width"=156, "Reserved"=0}, {"flags"=5, "Echo"=0, "Radial distance"=19.32, "Horizontal angle"=0.06981317007977318, "Vertical angle"=-0.006981317007977317, "Echo pulse width"=128, "Reserved"=0}, {"flags"=4, "Echo"=1, "Radial distance"=21.68, "Horizontal angle"=0.06981317007977318, "Vertical angle"=-0.006981317007977317, "Echo pulse width"=292, "Reserved"=0}, {"flags"=4, "Echo"=0, "Radial distance"=23.46, "Horizontal angle"=0.06544984694978735, "Vertical angle"=0.00698131700797732, "Echo pulse width"=200, "Reserved"=0}, {"flags"=4, "Echo"=0, "Radial distance"=24.44, "Horizontal angle"=0.06544984694978735, "Vertical angle"=0.020943951023931963, "Echo pulse width"=180, "Reserved"=0}, {"flags"=5, "Echo"=0, "Radial distance"=16.88, "Horizontal angle"=0.061086523819801536, "Vertical angle"=-0.020943951023931952, "Echo pulse width"=236, "Reserved"=0}, {"flags"=0, "Echo"=1, "Radial distance"=20.56, "Horizontal angle"=0.061086523819801536, "Vertical angle"=-0.020943951023931952, "Echo pulse width"=132, "Reserved"=10}, {"flags"=1, "Echo"=0, "Radial distance"=20.75, "Horizontal angle"=0.061086523819801536, "Vertical angle"=-0.006981317007977317, "Echo pulse width"=124, "Reserved"=10}, {"flags"=5, "Echo"=1, "Radial distance"=22.91, "Horizontal angle"=0.061086523819801536, "Vertical angle"=-0.006981317007977317, "Echo pulse width"=200, "Reserved"=0}, {"flags"=0, "Echo"=2, "Radial distance"=24.85, "Horizontal angle"=0.061086523819801536, "Vertical angle"=-0.006981317007977317, "Echo pulse width"=156, "Reserved"=12}, {"flags"=0, "Echo"=0, "Radial distance"=25.14, "Horizontal angle"=0.056723200689815706, "Vertical angle"=0.00698131700797732, "Echo pulse width"=204, "Reserved"=12}, {"flags"=0, "Echo"=0, "Radial distance"=26.37, "Horizontal angle"=0.056723200689815706, "Vertical angle"=0.020943951023931963, "Echo pulse width"=64, "Reserved"=13}, {"flags"=5, "Echo"=0, "Radial distance"=18.31, "Horizontal angle"=0.05235987755982988, "Vertical angle"=-0.020943951023931952, "Echo pulse width"=248, "Reserved"=0}, {"flags"=0, "Echo"=1, "Radial distance"=22.41, "Horizontal angle"=0.05235987755982988, "Vertical angle"=-0.020943951023931952, "Echo pulse width"=84, "Reserved"=14}, {"flags"=1, "Echo"=0, "Radial distance"=22.6, "Horizontal angle"=0.05235987755982988, "Vertical angle"=-0.006981317007977317, "Echo pulse width"=136, "Reserved"=14}, {"flags"=1, "Echo"=1, "Radial distance"=24.97, "Horizontal angle"=0.05235987755982988, "Vertical angle"=-0.006981317007977317, "Echo pulse width"=144, "Reserved"=12}, {"flags"=0, "Echo"=2, "Radial distance"=26.560000000000002, "Horizontal angle"=0.05235987755982988, "Vertical angle"=-0.006981317007977317, "Echo pulse width"=128, "Reserved"=13}, {"flags"=4, "Echo"=0, "Radial distance"=32.79, "Horizontal angle"=0.04799655442984406, "Vertical angle"=0.00698131700797732, "Echo pulse width"=176, "Reserved"=0}, {"flags"=4, "Echo"=0, "Radial distance"=20.11, "Horizontal angle"=0.04363323129985824, "Vertical angle"=-0.020943951023931952, "Echo pulse width"=264, "Reserved"=0}, {"flags"=5, "Echo"=0, "Radial distance"=24.76, "Horizontal angle"=0.04363323129985824, "Vertical angle"=-0.006981317007977317, "Echo pulse width"=132, "Reserved"=0}, {"flags"=5, "Echo"=1, "Radial distance"=28.05, "Horizontal angle"=0.04363323129985824, "Vertical angle"=-0.006981317007977317, "Echo pulse width"=224, "Reserved"=0}, {"flags"=4, "Echo"=2, "Radial distance"=31.12, "Horizontal angle"=0.04363323129985824, "Vertical angle"=-0.006981317007977317, "Echo pulse width"=92, "Reserved"=0}, {"flags"=4, "Echo"=0, "Radial distance"=32.99, "Horizontal angle"=0.039269908169872414, "Vertical angle"=0.00698131700797732, "Echo pulse width"=180, "Reserved"=0}, {"flags"=4, "Echo"=0, "Radial distance"=22.52, "Horizontal angle"=0.03490658503988659, "Vertical angle"=-0.020943951023931952, "Echo pulse width"=236, "Reserved"=0}, {"flags"=5, "Echo"=0, "Radial distance"=27.490000000000002, "Horizontal angle"=0.03490658503988659, "Vertical angle"=-0.006981317007977317, "Echo pulse width"=144, "Reserved"=0}, {"flags"=4, "Echo"=1, "Radial distance"=31.14, "Horizontal angle"=0.03490658503988659, "Vertical angle"=-0.006981317007977317, "Echo pulse width"=208, "Reserved"=0}, {"flags"=0, "Echo"=0, "Radial distance"=33.94, "Horizontal angle"=0.030543261909900768, "Vertical angle"=0.00698131700797732, "Echo pulse width"=200, "Reserved"=15}, {"flags"=4, "Echo"=0, "Radial distance"=24.73, "Horizontal angle"=0.02617993877991494, "Vertical angle"=-0.020943951023931952, "Echo pulse width"=80, "Reserved"=0}, {"flags"=5, "Echo"=0, "Radial distance"=30.580000000000002, "Horizontal angle"=0.02617993877991494, "Vertical angle"=-0.006981317007977317, "Echo pulse width"=168, "Reserved"=0}, {"flags"=1, "Echo"=1, "Radial distance"=34.27, "Horizontal angle"=0.02617993877991494, "Vertical angle"=-0.006981317007977317, "Echo pulse width"=112, "Reserved"=15}, {"flags"=4, "Echo"=2, "Radial distance"=36.050000000000004, "Horizontal angle"=0.02617993877991494, "Vertical angle"=-0.006981317007977317, "Echo pulse width"=76, "Reserved"=0}, {"flags"=4, "Echo"=0, "Radial distance"=37.57, "Horizontal angle"=0.02181661564992912, "Vertical angle"=0.00698131700797732, "Echo pulse width"=236, "Reserved"=0}, {"flags"=5, "Echo"=0, "Radial distance"=29.080000000000002, "Horizontal angle"=0.017453292519943295, "Vertical angle"=-0.006981317007977317, "Echo pulse width"=192, "Reserved"=0}, {"flags"=5, "Echo"=1, "Radial distance"=34.93, "Horizontal angle"=0.017453292519943295, "Vertical angle"=-0.006981317007977317, "Echo pulse width"=100, "Reserved"=0}, {"flags"=4, "Echo"=2, "Radial distance"=38.480000000000004, "Horizontal angle"=0.017453292519943295, "Vertical angle"=-0.006981317007977317, "Echo pulse width"=132, "Reserved"=0}, {"flags"=0, "Echo"=0, "Radial distance"=54.64, "Horizontal angle"=0.01308996938995747, "Vertical angle"=0.00698131700797732, "Echo pulse width"=188, "Reserved"=16}, {"flags"=0, "Echo"=0, "Radial distance"=54.18, "Horizontal angle"=0.01308996938995747, "Vertical angle"=0.020943951023931963, "Echo pulse width"=92, "Reserved"=16}, {"flags"=5, "Echo"=0, "Radial distance"=32.88, "Horizontal angle"=0.008726646259971648, "Vertical angle"=-0.006981317007977317, "Echo pulse width"=192, "Reserved"=0}, {"flags"=5, "Echo"=1, "Radial distance"=34.25, "Horizontal angle"=0.008726646259971648, "Vertical angle"=-0.006981317007977317, "Echo pulse width"=76, "Reserved"=0}, {"flags"=4, "Echo"=2, "Radial distance"=40.58, "Horizontal angle"=0.008726646259971648, "Vertical angle"=-0.006981317007977317, "Echo pulse width"=104, "Reserved"=0}, {"flags"=4, "Echo"=0, "Radial distance"=22.93, "Horizontal angle"=0.0, "Vertical angle"=-0.020943951023931952, "Echo pulse width"=84, "Reserved"=0}, {"flags"=4, "Echo"=0, "Radial distance"=22.61, "Horizontal angle"=-0.008726646259971648, "Vertical angle"=-0.020943951023931952, "Echo pulse width"=208, "Reserved"=0}, {"flags"=0, "Echo"=0, "Radial distance"=71.72, "Horizontal angle"=-0.01308996938995747, "Vertical angle"=0.00698131700797732, "Echo pulse width"=144, "Reserved"=17}, {"flags"=5, "Echo"=0, "Radial distance"=21.75, "Horizontal angle"=-0.017453292519943295, "Vertical angle"=-0.020943951023931952, "Echo pulse width"=188, "Reserved"=0}, {"flags"=4, "Echo"=1, "Radial distance"=23.55, "Horizontal angle"=-0.017453292519943295, "Vertical angle"=-0.020943951023931952, "Echo pulse width"=120, "Reserved"=0}, {"flags"=0, "Echo"=0, "Radial distance"=71.49, "Horizontal angle"=-0.017453292519943295, "Vertical angle"=-0.006981317007977317, "Echo pulse width"=52, "Reserved"=17}, {"flags"=5, "Echo"=0, "Radial distance"=21.03, "Horizontal angle"=-0.02617993877991494, "Vertical angle"=-0.020943951023931952, "Echo pulse width"=184, "Reserved"=0}, {"flags"=4, "Echo"=1, "Radial distance"=24.19, "Horizontal angle"=-0.02617993877991494, "Vertical angle"=-0.020943951023931952, "Echo pulse width"=112, "Reserved"=0}, {"flags"=0, "Echo"=0, "Radial distance"=58.050000000000004, "Horizontal angle"=-0.02617993877991494, "Vertical angle"=-0.006981317007977317, "Echo pulse width"=48, "Reserved"=18}, {"flags"=5, "Echo"=0, "Radial distance"=21.240000000000002, "Horizontal angle"=-0.03490658503988659, "Vertical angle"=-0.020943951023931952, "Echo pulse width"=168, "Reserved"=0}, {"flags"=4, "Echo"=1, "Radial distance"=24.47, "Horizontal angle"=-0.03490658503988659, "Vertical angle"=-0.020943951023931952, "Echo pulse width"=116, "Reserved"=0}, {"flags"=5, "Echo"=0, "Radial distance"=21.830000000000002, "Horizontal angle"=-0.04363323129985824, "Vertical angle"=-0.020943951023931952, "Echo pulse width"=164, "Reserved"=0}, {"flags"=4, "Echo"=1, "Radial distance"=23.71, "Horizontal angle"=-0.04363323129985824, "Vertical angle"=-0.020943951023931952, "Echo pulse width"=116, "Reserved"=0}, {"flags"=4, "Echo"=0, "Radial distance"=22.650000000000002, "Horizontal angle"=-0.05235987755982988, "Vertical angle"=-0.020943951023931952, "Echo pulse width"=212, "Reserved"=0}, {"flags"=0, "Echo"=0, "Radial distance"=229.02, "Horizontal angle"=-0.06544984694978735, "Vertical angle"=0.00698131700797732, "Echo pulse width"=128, "Reserved"=19}, {"flags"=0, "Echo"=0, "Radial distance"=188.3, "Horizontal angle"=-0.06544984694978735, "Vertical angle"=0.020943951023931963, "Echo pulse width"=144, "Reserved"=20}, {"flags"=1, "Echo"=0, "Radial distance"=38.07, "Horizontal angle"=-0.06981317007977318, "Vertical angle"=-0.006981317007977317, "Echo pulse width"=204, "Reserved"=21}, {"flags"=1, "Echo"=1, "Radial distance"=39.56, "Horizontal angle"=-0.06981317007977318, "Vertical angle"=-0.006981317007977317, "Echo pulse width"=88, "Reserved"=22}, {"flags"=0, "Echo"=2, "Radial distance"=57.84, "Horizontal angle"=-0.06981317007977318, "Vertical angle"=-0.006981317007977317, "Echo pulse width"=36, "Reserved"=23}, {"flags"=4, "Echo"=0, "Radial distance"=30.03, "Horizontal angle"=-0.07853981633974483, "Vertical angle"=-0.006981317007977317, "Echo pulse width"=200, "Reserved"=0}, {"flags"=4, "Echo"=0, "Radial distance"=21.91, "Horizontal angle"=-0.08726646259971647, "Vertical angle"=-0.020943951023931952, "Echo pulse width"=340, "Reserved"=0}, {"flags"=0, "Echo"=0, "Radial distance"=58.21, "Horizontal angle"=-0.08726646259971647, "Vertical angle"=-0.006981317007977317, "Echo pulse width"=52, "Reserved"=24}, {"flags"=0, "Echo"=0, "Radial distance"=88.99, "Horizontal angle"=-0.10035643198967394, "Vertical angle"=0.00698131700797732, "Echo pulse width"=76, "Reserved"=25}, {"flags"=4, "Echo"=0, "Radial distance"=15.52, "Horizontal angle"=-0.10471975511965977, "Vertical angle"=-0.020943951023931952, "Echo pulse width"=236, "Reserved"=0}, {"flags"=0, "Echo"=0, "Radial distance"=89.03, "Horizontal angle"=-0.1090830782496456, "Vertical angle"=0.00698131700797732, "Echo pulse width"=140, "Reserved"=25}, {"flags"=4, "Echo"=0, "Radial distance"=14.870000000000001, "Horizontal angle"=-0.11344640137963141, "Vertical angle"=-0.020943951023931952, "Echo pulse width"=76, "Reserved"=0}, {"flags"=0, "Echo"=0, "Radial distance"=287.03000000000003, "Horizontal angle"=-0.11780972450961724, "Vertical angle"=0.00698131700797732, "Echo pulse width"=140, "Reserved"=26}, {"flags"=4, "Echo"=0, "Radial distance"=22.91, "Horizontal angle"=-0.12217304763960307, "Vertical angle"=-0.020943951023931952, "Echo pulse width"=116, "Reserved"=0}, {"flags"=0, "Echo"=0, "Radial distance"=69.89, "Horizontal angle"=-0.1265363707695889, "Vertical angle"=0.020943951023931963, "Echo pulse width"=132, "Reserved"=27}, {"flags"=4, "Echo"=0, "Radial distance"=22.91, "Horizontal angle"=-0.1308996938995747, "Vertical angle"=-0.020943951023931952, "Echo pulse width"=252, "Reserved"=0}, {"flags"=0, "Echo"=0, "Radial distance"=153.20000000000002, "Horizontal angle"=-0.13526301702956053, "Vertical angle"=0.020943951023931963, "Echo pulse width"=48, "Reserved"=28}, {"flags"=5, "Echo"=0, "Radial distance"=22.1, "Horizontal angle"=-0.13962634015954636, "Vertical angle"=-0.020943951023931952, "Echo pulse width"=156, "Reserved"=0}, {"flags"=4, "Echo"=1, "Radial distance"=24.42, "Horizontal angle"=-0.13962634015954636, "Vertical angle"=-0.020943951023931952, "Echo pulse width"=152, "Reserved"=0}, {"flags"=4, "Echo"=0, "Radial distance"=47.07, "Horizontal angle"=-0.13962634015954636, "Vertical angle"=-0.006981317007977317, "Echo pulse width"=40, "Reserved"=0}, {"flags"=5, "Echo"=0, "Radial distance"=21.6, "Horizontal angle"=-0.148352986419518, "Vertical angle"=-0.020943951023931952, "Echo pulse width"=172, "Reserved"=0}, {"flags"=4, "Echo"=1, "Radial distance"=24.560000000000002, "Horizontal angle"=-0.148352986419518, "Vertical angle"=-0.020943951023931952, "Echo pulse width"=88, "Reserved"=0}, {"flags"=4, "Echo"=0, "Radial distance"=42.27, "Horizontal angle"=-0.148352986419518, "Vertical angle"=-0.006981317007977317, "Echo pulse width"=84, "Reserved"=0}, {"flags"=0, "Echo"=0, "Radial distance"=96.75, "Horizontal angle"=-0.15271630954950383, "Vertical angle"=0.00698131700797732, "Echo pulse width"=136, "Reserved"=29}, {"flags"=5, "Echo"=0, "Radial distance"=21.12, "Horizontal angle"=-0.15707963267948966, "Vertical angle"=-0.020943951023931952, "Echo pulse width"=176, "Reserved"=0}, {"flags"=4, "Echo"=1, "Radial distance"=24.02, "Horizontal angle"=-0.15707963267948966, "Vertical angle"=-0.020943951023931952, "Echo pulse width"=96, "Reserved"=0}, {"flags"=4, "Echo"=0, "Radial distance"=38.67, "Horizontal angle"=-0.15707963267948966, "Vertical angle"=-0.006981317007977317, "Echo pulse width"=120, "Reserved"=0}, {"flags"=0, "Echo"=0, "Radial distance"=84.31, "Horizontal angle"=-0.16144295580947549, "Vertical angle"=0.00698131700797732, "Echo pulse width"=104, "Reserved"=30}, {"flags"=5, "Echo"=0, "Radial distance"=21.52, "Horizontal angle"=-0.16580627893946132, "Vertical angle"=-0.020943951023931952, "Echo pulse width"=232, "Reserved"=0}, {"flags"=4, "Echo"=1, "Radial distance"=23.6, "Horizontal angle"=-0.16580627893946132, "Vertical angle"=-0.020943951023931952, "Echo pulse width"=92, "Reserved"=0}, {"flags"=5, "Echo"=0, "Radial distance"=30.400000000000002, "Horizontal angle"=-0.16580627893946132, "Vertical angle"=-0.006981317007977317, "Echo pulse width"=132, "Reserved"=0}, {"flags"=4, "Echo"=1, "Radial distance"=35.68, "Horizontal angle"=-0.16580627893946132, "Vertical angle"=-0.006981317007977317, "Echo pulse width"=128, "Reserved"=0}, {"flags"=1, "Echo"=0, "Radial distance"=74.71000000000001, "Horizontal angle"=-0.17016960206944715, "Vertical angle"=0.00698131700797732, "Echo pulse width"=104, "Reserved"=31}, {"flags"=0, "Echo"=1, "Radial distance"=76.92, "Horizontal angle"=-0.17016960206944715, "Vertical angle"=0.00698131700797732, "Echo pulse width"=148, "Reserved"=32}, {"flags"=0, "Echo"=0, "Radial distance"=76.97, "Horizontal angle"=-0.17016960206944715, "Vertical angle"=0.020943951023931963, "Echo pulse width"=128, "Reserved"=32}, {"flags"=4, "Echo"=0, "Radial distance"=22.63, "Horizontal angle"=-0.17453292519943295, "Vertical angle"=-0.020943951023931952, "Echo pulse width"=224, "Reserved"=0}, {"flags"=4, "Echo"=0, "Radial distance"=33.160000000000004, "Horizontal angle"=-0.17453292519943295, "Vertical angle"=-0.006981317007977317, "Echo pulse width"=128, "Reserved"=0}, {"flags"=0, "Echo"=0, "Radial distance"=70.54, "Horizontal angle"=-0.17889624832941878, "Vertical angle"=0.00698131700797732, "Echo pulse width"=128, "Reserved"=33}, {"flags"=4, "Echo"=0, "Radial distance"=31.080000000000002, "Horizontal angle"=-0.1832595714594046, "Vertical angle"=-0.006981317007977317, "Echo pulse width"=128, "Reserved"=0}, {"flags"=0, "Echo"=0, "Radial distance"=62.67, "Horizontal angle"=-0.18762289458939044, "Vertical angle"=0.00698131700797732, "Echo pulse width"=136, "Reserved"=34}, {"flags"=4, "Echo"=0, "Radial distance"=24.96, "Horizontal angle"=-0.19198621771937624, "Vertical angle"=-0.020943951023931952, "Echo pulse width"=136, "Reserved"=0}, {"flags"=4, "Echo"=0, "Radial distance"=29.32, "Horizontal angle"=-0.19198621771937624, "Vertical angle"=-0.006981317007977317, "Echo pulse width"=136, "Reserved"=0}, {"flags"=0, "Echo"=0, "Radial distance"=58.64, "Horizontal angle"=-0.19634954084936207, "Vertical angle"=0.00698131700797732, "Echo pulse width"=148, "Reserved"=35}, {"flags"=0, "Echo"=0, "Radial distance"=70.59, "Horizontal angle"=-0.19634954084936207, "Vertical angle"=0.020943951023931963, "Echo pulse width"=116, "Reserved"=36}, {"flags"=4, "Echo"=0, "Radial distance"=23.59, "Horizontal angle"=-0.20071286397934787, "Vertical angle"=-0.020943951023931952, "Echo pulse width"=160, "Reserved"=0}, {"flags"=4, "Echo"=0, "Radial distance"=27.68, "Horizontal angle"=-0.20071286397934787, "Vertical angle"=-0.006981317007977317, "Echo pulse width"=136, "Reserved"=0}, {"flags"=0, "Echo"=0, "Radial distance"=54.61, "Horizontal angle"=-0.20507618710933373, "Vertical angle"=0.00698131700797732, "Echo pulse width"=152, "Reserved"=37}, {"flags"=0, "Echo"=0, "Radial distance"=94.06, "Horizontal angle"=-0.20507618710933373, "Vertical angle"=0.020943951023931963, "Echo pulse width"=108, "Reserved"=38}, {"flags"=4, "Echo"=0, "Radial distance"=22.32, "Horizontal angle"=-0.20943951023931953, "Vertical angle"=-0.020943951023931952, "Echo pulse width"=172, "Reserved"=0}, {"flags"=4, "Echo"=0, "Radial distance"=26.16, "Horizontal angle"=-0.20943951023931953, "Vertical angle"=-0.006981317007977317, "Echo pulse width"=140, "Reserved"=0}, {"flags"=5, "Echo"=0, "Radial distance"=49.84, "Horizontal angle"=-0.21380283336930533, "Vertical angle"=0.00698131700797732, "Echo pulse width"=148, "Reserved"=0}, {"flags"=0, "Echo"=1, "Radial distance"=54.76, "Horizontal angle"=-0.21380283336930533, "Vertical angle"=0.00698131700797732, "Echo pulse width"=56, "Reserved"=37}, {"flags"=1, "Echo"=0, "Radial distance"=58.45, "Horizontal angle"=-0.21380283336930533, "Vertical angle"=0.020943951023931963, "Echo pulse width"=32, "Reserved"=39}, {"flags"=0, "Echo"=1, "Radial distance"=62.25, "Horizontal angle"=-0.21380283336930533, "Vertical angle"=0.020943951023931963, "Echo pulse width"=64, "Reserved"=40}, {"flags"=4, "Echo"=0, "Radial distance"=21.150000000000002, "Horizontal angle"=-0.2181661564992912, "Vertical angle"=-0.020943951023931952, "Echo pulse width"=164, "Reserved"=0}, {"flags"=5, "Echo"=0, "Radial distance"=24.97, "Horizontal angle"=-0.2181661564992912, "Vertical angle"=-0.006981317007977317, "Echo pulse width"=144, "Reserved"=0}, {"flags"=4, "Echo"=1, "Radial distance"=26.35, "Horizontal angle"=-0.2181661564992912, "Vertical angle"=-0.006981317007977317, "Echo pulse width"=64, "Reserved"=0}, {"flags"=4, "Echo"=0, "Radial distance"=49.5, "Horizontal angle"=-0.222529479629277, "Vertical angle"=0.00698131700797732, "Echo pulse width"=160, "Reserved"=0}, {"flags"=0, "Echo"=0, "Radial distance"=93.9, "Horizontal angle"=-0.222529479629277, "Vertical angle"=0.020943951023931963, "Echo pulse width"=92, "Reserved"=41}, {"flags"=5, "Echo"=0, "Radial distance"=20.13, "Horizontal angle"=-0.22689280275926282, "Vertical angle"=-0.020943951023931952, "Echo pulse width"=148, "Reserved"=0}, {"flags"=4, "Echo"=1, "Radial distance"=22.12, "Horizontal angle"=-0.22689280275926282, "Vertical angle"=-0.020943951023931952, "Echo pulse width"=136, "Reserved"=0}, {"flags"=5, "Echo"=0, "Radial distance"=23.72, "Horizontal angle"=-0.22689280275926282, "Vertical angle"=-0.006981317007977317, "Echo pulse width"=136, "Reserved"=0}, {"flags"=4, "Echo"=1, "Radial distance"=25.01, "Horizontal angle"=-0.22689280275926282, "Vertical angle"=-0.006981317007977317, "Echo pulse width"=100, "Reserved"=0}, {"flags"=4, "Echo"=0, "Radial distance"=44.88, "Horizontal angle"=-0.23125612588924865, "Vertical angle"=0.00698131700797732, "Echo pulse width"=148, "Reserved"=0}, {"flags"=0, "Echo"=0, "Radial distance"=63.27, "Horizontal angle"=-0.23125612588924865, "Vertical angle"=0.020943951023931963, "Echo pulse width"=112, "Reserved"=42}, {"flags"=5, "Echo"=0, "Radial distance"=19.240000000000002, "Horizontal angle"=-0.23561944901923448, "Vertical angle"=-0.020943951023931952, "Echo pulse width"=168, "Reserved"=0}, {"flags"=0, "Echo"=1, "Radial distance"=22.32, "Horizontal angle"=-0.23561944901923448, "Vertical angle"=-0.020943951023931952, "Echo pulse width"=176, "Reserved"=43}, {"flags"=4, "Echo"=0, "Radial distance"=23.06, "Horizontal angle"=-0.23561944901923448, "Vertical angle"=-0.006981317007977317, "Echo pulse width"=244, "Reserved"=0}, {"flags"=4, "Echo"=0, "Radial distance"=44.5, "Horizontal angle"=-0.2399827721492203, "Vertical angle"=0.00698131700797732, "Echo pulse width"=160, "Reserved"=0}, {"flags"=0, "Echo"=0, "Radial distance"=74.82000000000001, "Horizontal angle"=-0.2399827721492203, "Vertical angle"=0.020943951023931963, "Echo pulse width"=84, "Reserved"=44}, {"flags"=5, "Echo"=0, "Radial distance"=18.48, "Horizontal angle"=-0.24434609527920614, "Vertical angle"=-0.020943951023931952, "Echo pulse width"=176, "Reserved"=0}, {"flags"=0, "Echo"=1, "Radial distance"=21.59, "Horizontal angle"=-0.24434609527920614, "Vertical angle"=-0.020943951023931952, "Echo pulse width"=116, "Reserved"=43}, {"flags"=0, "Echo"=0, "Radial distance"=22.1, "Horizontal angle"=-0.24434609527920614, "Vertical angle"=-0.006981317007977317, "Echo pulse width"=248, "Reserved"=43}, {"flags"=1, "Echo"=0, "Radial distance"=39.93, "Horizontal angle"=-0.24870941840919195, "Vertical angle"=0.00698131700797732, "Echo pulse width"=156, "Reserved"=45}, {"flags"=0, "Echo"=1, "Radial distance"=44.6, "Horizontal angle"=-0.24870941840919195, "Vertical angle"=0.00698131700797732, "Echo pulse width"=84, "Reserved"=46}, {"flags"=0, "Echo"=0, "Radial distance"=95.45, "Horizontal angle"=-0.24870941840919195, "Vertical angle"=0.020943951023931963, "Echo pulse width"=76, "Reserved"=47}, {"flags"=5, "Echo"=0, "Radial distance"=17.68, "Horizontal angle"=-0.2530727415391778, "Vertical angle"=-0.020943951023931952, "Echo pulse width"=176, "Reserved"=0}, {"flags"=0, "Echo"=1, "Radial distance"=20.39, "Horizontal angle"=-0.2530727415391778, "Vertical angle"=-0.020943951023931952, "Echo pulse width"=196, "Reserved"=48}, {"flags"=0, "Echo"=0, "Radial distance"=21.32, "Horizontal angle"=-0.2530727415391778, "Vertical angle"=-0.006981317007977317, "Echo pulse width"=264, "Reserved"=43}, {"flags"=0, "Echo"=0, "Radial distance"=39.7, "Horizontal angle"=-0.2574360646691636, "Vertical angle"=0.00698131700797732, "Echo pulse width"=168, "Reserved"=45}, {"flags"=0, "Echo"=0, "Radial distance"=39.83, "Horizontal angle"=-0.2574360646691636, "Vertical angle"=0.020943951023931963, "Echo pulse width"=116, "Reserved"=45}, {"flags"=5, "Echo"=0, "Radial distance"=17.03, "Horizontal angle"=-0.2617993877991494, "Vertical angle"=-0.020943951023931952, "Echo pulse width"=192, "Reserved"=0}, {"flags"=4, "Echo"=1, "Radial distance"=19.43, "Horizontal angle"=-0.2617993877991494, "Vertical angle"=-0.020943951023931952, "Echo pulse width"=220, "Reserved"=0}, {"flags"=1, "Echo"=0, "Radial distance"=20.57, "Horizontal angle"=-0.2617993877991494, "Vertical angle"=-0.006981317007977317, "Echo pulse width"=232, "Reserved"=48}, {"flags"=4, "Echo"=1, "Radial distance"=22.67, "Horizontal angle"=-0.2617993877991494, "Vertical angle"=-0.006981317007977317, "Echo pulse width"=120, "Reserved"=0}, {"flags"=0, "Echo"=0, "Radial distance"=39.62, "Horizontal angle"=-0.26616271092913524, "Vertical angle"=0.00698131700797732, "Echo pulse width"=168, "Reserved"=45}, {"flags"=0, "Echo"=0, "Radial distance"=39.83, "Horizontal angle"=-0.26616271092913524, "Vertical angle"=0.020943951023931963, "Echo pulse width"=116, "Reserved"=45}, {"flags"=4, "Echo"=0, "Radial distance"=16.53, "Horizontal angle"=-0.27052603405912107, "Vertical angle"=-0.020943951023931952, "Echo pulse width"=440, "Reserved"=0}, {"flags"=5, "Echo"=0, "Radial distance"=20.080000000000002, "Horizontal angle"=-0.27052603405912107, "Vertical angle"=-0.006981317007977317, "Echo pulse width"=260, "Reserved"=0}, {"flags"=4, "Echo"=1, "Radial distance"=22.47, "Horizontal angle"=-0.27052603405912107, "Vertical angle"=-0.006981317007977317, "Echo pulse width"=64, "Reserved"=0}, {"flags"=0, "Echo"=0, "Radial distance"=39.9, "Horizontal angle"=-0.2748893571891069, "Vertical angle"=0.00698131700797732, "Echo pulse width"=172, "Reserved"=45}, {"flags"=0, "Echo"=0, "Radial distance"=95.94, "Horizontal angle"=-0.2748893571891069, "Vertical angle"=0.020943951023931963, "Echo pulse width"=92, "Reserved"=49}, {"flags"=4, "Echo"=0, "Radial distance"=16.05, "Horizontal angle"=-0.2792526803190927, "Vertical angle"=-0.020943951023931952, "Echo pulse width"=424, "Reserved"=0}, {"flags"=5, "Echo"=0, "Radial distance"=19.42, "Horizontal angle"=-0.2792526803190927, "Vertical angle"=-0.006981317007977317, "Echo pulse width"=160, "Reserved"=0}, {"flags"=5, "Echo"=1, "Radial distance"=20.650000000000002, "Horizontal angle"=-0.2792526803190927, "Vertical angle"=-0.006981317007977317, "Echo pulse width"=76, "Reserved"=0}, {"flags"=4, "Echo"=2, "Radial distance"=22.6, "Horizontal angle"=-0.2792526803190927, "Vertical angle"=-0.006981317007977317, "Echo pulse width"=60, "Reserved"=0}, {"flags"=0, "Echo"=0, "Radial distance"=34.82, "Horizontal angle"=-0.28361600344907856, "Vertical angle"=0.00698131700797732, "Echo pulse width"=172, "Reserved"=50}, {"flags"=1, "Echo"=0, "Radial distance"=35.06, "Horizontal angle"=-0.28361600344907856, "Vertical angle"=0.020943951023931963, "Echo pulse width"=148, "Reserved"=50}, {"flags"=0, "Echo"=1, "Radial distance"=59.39, "Horizontal angle"=-0.28361600344907856, "Vertical angle"=0.020943951023931963, "Echo pulse width"=96, "Reserved"=51}, {"flags"=4, "Echo"=0, "Radial distance"=15.81, "Horizontal angle"=-0.28797932657906433, "Vertical angle"=-0.020943951023931952, "Echo pulse width"=392, "Reserved"=0}, {"flags"=5, "Echo"=0, "Radial distance"=19.1, "Horizontal angle"=-0.28797932657906433, "Vertical angle"=-0.006981317007977317, "Echo pulse width"=208, "Reserved"=0}, {"flags"=5, "Echo"=1, "Radial distance"=20.830000000000002, "Horizontal angle"=-0.28797932657906433, "Vertical angle"=-0.006981317007977317, "Echo pulse width"=40, "Reserved"=0}, {"flags"=4, "Echo"=2, "Radial distance"=22.11, "Horizontal angle"=-0.28797932657906433, "Vertical angle"=-0.006981317007977317, "Echo pulse width"=84, "Reserved"=0}, {"flags"=0, "Echo"=0, "Radial distance"=34.79, "Horizontal angle"=-0.2923426497090502, "Vertical angle"=0.00698131700797732, "Echo pulse width"=176, "Reserved"=50}, {"flags"=1, "Echo"=0, "Radial distance"=34.99, "Horizontal angle"=-0.2923426497090502, "Vertical angle"=0.020943951023931963, "Echo pulse width"=160, "Reserved"=50}, {"flags"=0, "Echo"=1, "Radial distance"=94.31, "Horizontal angle"=-0.2923426497090502, "Vertical angle"=0.020943951023931963, "Echo pulse width"=12, "Reserved"=52}, {"flags"=4, "Echo"=0, "Radial distance"=16.43, "Horizontal angle"=-0.296705972839036, "Vertical angle"=-0.020943951023931952, "Echo pulse width"=268, "Reserved"=0}, {"flags"=5, "Echo"=0, "Radial distance"=18.740000000000002, "Horizontal angle"=-0.296705972839036, "Vertical angle"=-0.006981317007977317, "Echo pulse width"=244, "Reserved"=0}, {"flags"=4, "Echo"=1, "Radial distance"=21.62, "Horizontal angle"=-0.296705972839036, "Vertical angle"=-0.006981317007977317, "Echo pulse width"=168, "Reserved"=0}, {"flags"=4, "Echo"=0, "Radial distance"=34.03, "Horizontal angle"=-0.3010692959690219, "Vertical angle"=0.00698131700797732, "Echo pulse width"=264, "Reserved"=0}, {"flags"=0, "Echo"=0, "Radial distance"=34.9, "Horizontal angle"=-0.3010692959690219, "Vertical angle"=0.020943951023931963, "Echo pulse width"=148, "Reserved"=50}, {"flags"=4, "Echo"=0, "Radial distance"=16.35, "Horizontal angle"=-0.30543261909900765, "Vertical angle"=-0.020943951023931952, "Echo pulse width"=216, "Reserved"=0}, {"flags"=5, "Echo"=0, "Radial distance"=18.28, "Horizontal angle"=-0.30543261909900765, "Vertical angle"=-0.006981317007977317, "Echo pulse width"=296, "Reserved"=0}, {"flags"=5, "Echo"=1, "Radial distance"=21.87, "Horizontal angle"=-0.30543261909900765, "Vertical angle"=-0.006981317007977317, "Echo pulse width"=124, "Reserved"=0}, {"flags"=4, "Echo"=2, "Radial distance"=25.73, "Horizontal angle"=-0.30543261909900765, "Vertical angle"=-0.006981317007977317, "Echo pulse width"=76, "Reserved"=0}, {"flags"=5, "Echo"=0, "Radial distance"=33.47, "Horizontal angle"=-0.3097959422289935, "Vertical angle"=0.00698131700797732, "Echo pulse width"=192, "Reserved"=0}, {"flags"=0, "Echo"=1, "Radial distance"=35.18, "Horizontal angle"=-0.3097959422289935, "Vertical angle"=0.00698131700797732, "Echo pulse width"=132, "Reserved"=50}, {"flags"=0, "Echo"=0, "Radial distance"=81.47, "Horizontal angle"=-0.3097959422289935, "Vertical angle"=0.020943951023931963, "Echo pulse width"=96, "Reserved"=53}, {"flags"=4, "Echo"=0, "Radial distance"=16.080000000000002, "Horizontal angle"=-0.3141592653589793, "Vertical angle"=-0.020943951023931952, "Echo pulse width"=180, "Reserved"=0}, {"flags"=5, "Echo"=0, "Radial distance"=18.080000000000002, "Horizontal angle"=-0.3141592653589793, "Vertical angle"=-0.006981317007977317, "Echo pulse width"=272, "Reserved"=0}, {"flags"=5, "Echo"=1, "Radial distance"=21.150000000000002, "Horizontal angle"=-0.3141592653589793, "Vertical angle"=-0.006981317007977317, "Echo pulse width"=112, "Reserved"=0}, {"flags"=4, "Echo"=2, "Radial distance"=31.16, "Horizontal angle"=-0.3141592653589793, "Vertical angle"=-0.006981317007977317, "Echo pulse width"=88, "Reserved"=0}, {"flags"=1, "Echo"=0, "Radial distance"=30.3, "Horizontal angle"=-0.31852258848896514, "Vertical angle"=0.00698131700797732, "Echo pulse width"=172, "Reserved"=54}, {"flags"=4, "Echo"=1, "Radial distance"=33.27, "Horizontal angle"=-0.31852258848896514, "Vertical angle"=0.00698131700797732, "Echo pulse width"=104, "Reserved"=0}, {"flags"=1, "Echo"=0, "Radial distance"=30.21, "Horizontal angle"=-0.31852258848896514, "Vertical angle"=0.020943951023931963, "Echo pulse width"=136, "Reserved"=54}, {"flags"=5, "Echo"=1, "Radial distance"=34.26, "Horizontal angle"=-0.31852258848896514, "Vertical angle"=0.020943951023931963, "Echo pulse width"=80, "Reserved"=0}, {"flags"=0, "Echo"=2, "Radial distance"=83.43, "Horizontal angle"=-0.31852258848896514, "Vertical angle"=0.020943951023931963, "Echo pulse width"=112, "Reserved"=55}, {"flags"=4, "Echo"=0, "Radial distance"=15.67, "Horizontal angle"=-0.32288591161895097, "Vertical angle"=-0.020943951023931952, "Echo pulse width"=184, "Reserved"=0}, {"flags"=5, "Echo"=0, "Radial distance"=17.68, "Horizontal angle"=-0.32288591161895097, "Vertical angle"=-0.006981317007977317, "Echo pulse width"=312, "Reserved"=0}, {"flags"=5, "Echo"=1, "Radial distance"=20.95, "Horizontal angle"=-0.32288591161895097, "Vertical angle"=-0.006981317007977317, "Echo pulse width"=80, "Reserved"=0}, {"flags"=4, "Echo"=2, "Radial distance"=24.71, "Horizontal angle"=-0.32288591161895097, "Vertical angle"=-0.006981317007977317, "Echo pulse width"=84, "Reserved"=0}, {"flags"=0, "Echo"=0, "Radial distance"=30.07, "Horizontal angle"=-0.3272492347489368, "Vertical angle"=0.00698131700797732, "Echo pulse width"=180, "Reserved"=54}, {"flags"=1, "Echo"=0, "Radial distance"=30.080000000000002, "Horizontal angle"=-0.3272492347489368, "Vertical angle"=0.020943951023931963, "Echo pulse width"=168, "Reserved"=54}, {"flags"=0, "Echo"=1, "Radial distance"=63.910000000000004, "Horizontal angle"=-0.3272492347489368, "Vertical angle"=0.020943951023931963, "Echo pulse width"=112, "Reserved"=56}, {"flags"=4, "Echo"=0, "Radial distance"=15.31, "Horizontal angle"=-0.33161255787892263, "Vertical angle"=-0.020943951023931952, "Echo pulse width"=192, "Reserved"=0}, {"flags"=5, "Echo"=0, "Radial distance"=17.8, "Horizontal angle"=-0.33161255787892263, "Vertical angle"=-0.006981317007977317, "Echo pulse width"=292, "Reserved"=0}, {"flags"=5, "Echo"=1, "Radial distance"=20.87, "Horizontal angle"=-0.33161255787892263, "Vertical angle"=-0.006981317007977317, "Echo pulse width"=44, "Reserved"=0}, {"flags"=4, "Echo"=2, "Radial distance"=24.88, "Horizontal angle"=-0.33161255787892263, "Vertical angle"=-0.006981317007977317, "Echo pulse width"=92, "Reserved"=0}, {"flags"=0, "Echo"=0, "Radial distance"=29.98, "Horizontal angle"=-0.3359758810089084, "Vertical angle"=0.00698131700797732, "Echo pulse width"=172, "Reserved"=54}, {"flags"=1, "Echo"=0, "Radial distance"=30.04, "Horizontal angle"=-0.3359758810089084, "Vertical angle"=0.020943951023931963, "Echo pulse width"=172, "Reserved"=54}, {"flags"=0, "Echo"=1, "Radial distance"=82.82000000000001, "Horizontal angle"=-0.3359758810089084, "Vertical angle"=0.020943951023931963, "Echo pulse width"=104, "Reserved"=57}, {"flags"=4, "Echo"=0, "Radial distance"=14.93, "Horizontal angle"=-0.3403392041388943, "Vertical angle"=-0.020943951023931952, "Echo pulse width"=208, "Reserved"=0}, {"flags"=5, "Echo"=0, "Radial distance"=17.44, "Horizontal angle"=-0.3403392041388943, "Vertical angle"=-0.006981317007977317, "Echo pulse width"=312, "Reserved"=0}, {"flags"=5, "Echo"=1, "Radial distance"=24.6, "Horizontal angle"=-0.3403392041388943, "Vertical angle"=-0.006981317007977317, "Echo pulse width"=36, "Reserved"=0}, {"flags"=4, "Echo"=2, "Radial distance"=28.55, "Horizontal angle"=-0.3403392041388943, "Vertical angle"=-0.006981317007977317, "Echo pulse width"=120, "Reserved"=0}, {"flags"=0, "Echo"=0, "Radial distance"=30.11, "Horizontal angle"=-0.34470252726888007, "Vertical angle"=0.00698131700797732, "Echo pulse width"=176, "Reserved"=54}, {"flags"=0, "Echo"=0, "Radial distance"=30.11, "Horizontal angle"=-0.34470252726888007, "Vertical angle"=0.020943951023931963, "Echo pulse width"=160, "Reserved"=54}, {"flags"=4, "Echo"=0, "Radial distance"=14.55, "Horizontal angle"=-0.3490658503988659, "Vertical angle"=-0.020943951023931952, "Echo pulse width"=228, "Reserved"=0}, {"flags"=5, "Echo"=0, "Radial distance"=16.85, "Horizontal angle"=-0.3490658503988659, "Vertical angle"=-0.006981317007977317, "Echo pulse width"=336, "Reserved"=0}, {"flags"=4, "Echo"=1, "Radial distance"=27.68, "Horizontal angle"=-0.3490658503988659, "Vertical angle"=-0.006981317007977317, "Echo pulse width"=128, "Reserved"=0}, {"flags"=1, "Echo"=0, "Radial distance"=30.38, "Horizontal angle"=-0.3534291735288517, "Vertical angle"=0.00698131700797732, "Echo pulse width"=164, "Reserved"=54}, {"flags"=4, "Echo"=1, "Radial distance"=31.77, "Horizontal angle"=-0.3534291735288517, "Vertical angle"=0.00698131700797732, "Echo pulse width"=88, "Reserved"=0}, {"flags"=1, "Echo"=0, "Radial distance"=30.43, "Horizontal angle"=-0.3534291735288517, "Vertical angle"=0.020943951023931963, "Echo pulse width"=116, "Reserved"=54}, {"flags"=0, "Echo"=1, "Radial distance"=84.26, "Horizontal angle"=-0.3534291735288517, "Vertical angle"=0.020943951023931963, "Echo pulse width"=92, "Reserved"=58}, {"flags"=4, "Echo"=0, "Radial distance"=14.200000000000001, "Horizontal angle"=-0.35779249665883756, "Vertical angle"=-0.020943951023931952, "Echo pulse width"=220, "Reserved"=0}, {"flags"=5, "Echo"=0, "Radial distance"=16.81, "Horizontal angle"=-0.35779249665883756, "Vertical angle"=-0.006981317007977317, "Echo pulse width"=388, "Reserved"=0}, {"flags"=0, "Echo"=1, "Radial distance"=26.76, "Horizontal angle"=-0.35779249665883756, "Vertical angle"=-0.006981317007977317, "Echo pulse width"=132, "Reserved"=59}, {"flags"=1, "Echo"=0, "Radial distance"=27.01, "Horizontal angle"=-0.3621558197888234, "Vertical angle"=0.00698131700797732, "Echo pulse width"=120, "Reserved"=59}, {"flags"=4, "Echo"=1, "Radial distance"=31.62, "Horizontal angle"=-0.3621558197888234, "Vertical angle"=0.00698131700797732, "Echo pulse width"=132, "Reserved"=0}, {"flags"=4, "Echo"=0, "Radial distance"=13.790000000000001, "Horizontal angle"=-0.3665191429188092, "Vertical angle"=-0.020943951023931952, "Echo pulse width"=248, "Reserved"=0}, {"flags"=5, "Echo"=0, "Radial distance"=16.73, "Horizontal angle"=-0.3665191429188092, "Vertical angle"=-0.006981317007977317, "Echo pulse width"=360, "Reserved"=0}, {"flags"=4, "Echo"=1, "Radial distance"=26.240000000000002, "Horizontal angle"=-0.3665191429188092, "Vertical angle"=-0.006981317007977317, "Echo pulse width"=128, "Reserved"=0}, {"flags"=0, "Echo"=0, "Radial distance"=25.43, "Horizontal angle"=-0.370882466048795, "Vertical angle"=0.00698131700797732, "Echo pulse width"=192, "Reserved"=60}, {"flags"=1, "Echo"=0, "Radial distance"=25.310000000000002, "Horizontal angle"=-0.370882466048795, "Vertical angle"=0.020943951023931963, "Echo pulse width"=160, "Reserved"=60}, {"flags"=0, "Echo"=1, "Radial distance"=95.93, "Horizontal angle"=-0.370882466048795, "Vertical angle"=0.020943951023931963, "Echo pulse width"=36, "Reserved"=61}, {"flags"=4, "Echo"=0, "Radial distance"=13.51, "Horizontal angle"=-0.3752457891787809, "Vertical angle"=-0.020943951023931952, "Echo pulse width"=240, "Reserved"=0}, {"flags"=5, "Echo"=0, "Radial distance"=16.41, "Horizontal angle"=-0.3752457891787809, "Vertical angle"=-0.006981317007977317, "Echo pulse width"=364, "Reserved"=0}, {"flags"=0, "Echo"=1, "Radial distance"=25.55, "Horizontal angle"=-0.3752457891787809, "Vertical angle"=-0.006981317007977317, "Echo pulse width"=124, "Reserved"=60}, {"flags"=0, "Echo"=0, "Radial distance"=25.19, "Horizontal angle"=-0.37960911230876665, "Vertical angle"=0.00698131700797732, "Echo pulse width"=180, "Reserved"=60}, {"flags"=1, "Echo"=0, "Radial distance"=25.21, "Horizontal angle"=-0.37960911230876665, "Vertical angle"=0.020943951023931963, "Echo pulse width"=184, "Reserved"=60}, {"flags"=0, "Echo"=1, "Radial distance"=29.01, "Horizontal angle"=-0.37960911230876665, "Vertical angle"=0.020943951023931963, "Echo pulse width"=136, "Reserved"=62}, {"flags"=4, "Echo"=0, "Radial distance"=13.11, "Horizontal angle"=-0.3839724354387525, "Vertical angle"=-0.020943951023931952, "Echo pulse width"=272, "Reserved"=0}, {"flags"=5, "Echo"=0, "Radial distance"=16.09, "Horizontal angle"=-0.3839724354387525, "Vertical angle"=-0.006981317007977317, "Echo pulse width"=372, "Reserved"=0}, {"flags"=0, "Echo"=1, "Radial distance"=24.76, "Horizontal angle"=-0.3839724354387525, "Vertical angle"=-0.006981317007977317, "Echo pulse width"=136, "Reserved"=60}, {"flags"=0, "Echo"=0, "Radial distance"=25.11, "Horizontal angle"=-0.3883357585687383, "Vertical angle"=0.00698131700797732, "Echo pulse width"=176, "Reserved"=60}, {"flags"=1, "Echo"=0, "Radial distance"=25.13, "Horizontal angle"=-0.3883357585687383, "Vertical angle"=0.020943951023931963, "Echo pulse width"=188, "Reserved"=60}, {"flags"=0, "Echo"=1, "Radial distance"=29.09, "Horizontal angle"=-0.3883357585687383, "Vertical angle"=0.020943951023931963, "Echo pulse width"=136, "Reserved"=62}, {"flags"=4, "Echo"=0, "Radial distance"=12.91, "Horizontal angle"=-0.39269908169872414, "Vertical angle"=-0.020943951023931952, "Echo pulse width"=276, "Reserved"=0}, {"flags"=5, "Echo"=0, "Radial distance"=15.88, "Horizontal angle"=-0.39269908169872414, "Vertical angle"=-0.006981317007977317, "Echo pulse width"=216, "Reserved"=0}, {"flags"=5, "Echo"=1, "Radial distance"=18.09, "Horizontal angle"=-0.39269908169872414, "Vertical angle"=-0.006981317007977317, "Echo pulse width"=152, "Reserved"=0}, {"flags"=4, "Echo"=2, "Radial distance"=24.32, "Horizontal angle"=-0.39269908169872414, "Vertical angle"=-0.006981317007977317, "Echo pulse width"=136, "Reserved"=0}, {"flags"=0, "Echo"=0, "Radial distance"=25.150000000000002, "Horizontal angle"=-0.39706240482870997, "Vertical angle"=0.00698131700797732, "Echo pulse width"=192, "Reserved"=60}, {"flags"=1, "Echo"=0, "Radial distance"=25.17, "Horizontal angle"=-0.39706240482870997, "Vertical angle"=0.020943951023931963, "Echo pulse width"=184, "Reserved"=60}, {"flags"=0, "Echo"=1, "Radial distance"=29.14, "Horizontal angle"=-0.39706240482870997, "Vertical angle"=0.020943951023931963, "Echo pulse width"=144, "Reserved"=62}, {"flags"=4, "Echo"=0, "Radial distance"=12.55, "Horizontal angle"=-0.40142572795869574, "Vertical angle"=-0.020943951023931952, "Echo pulse width"=300, "Reserved"=0}, {"flags"=5, "Echo"=0, "Radial distance"=15.780000000000001, "Horizontal angle"=-0.40142572795869574, "Vertical angle"=-0.006981317007977317, "Echo pulse width"=212, "Reserved"=0}, {"flags"=5, "Echo"=1, "Radial distance"=17.85, "Horizontal angle"=-0.40142572795869574, "Vertical angle"=-0.006981317007977317, "Echo pulse width"=148, "Reserved"=0}, {"flags"=4, "Echo"=2, "Radial distance"=23.85, "Horizontal angle"=-0.40142572795869574, "Vertical angle"=-0.006981317007977317, "Echo pulse width"=144, "Reserved"=0}, {"flags"=0, "Echo"=0, "Radial distance"=25.19, "Horizontal angle"=-0.40578905108868163, "Vertical angle"=0.00698131700797732, "Echo pulse width"=196, "Reserved"=60}, {"flags"=0, "Echo"=0, "Radial distance"=25.44, "Horizontal angle"=-0.40578905108868163, "Vertical angle"=0.020943951023931963, "Echo pulse width"=288, "Reserved"=60}, {"flags"=4, "Echo"=0, "Radial distance"=12.31, "Horizontal angle"=-0.41015237421866746, "Vertical angle"=-0.020943951023931952, "Echo pulse width"=304, "Reserved"=0}, {"flags"=5, "Echo"=0, "Radial distance"=15.530000000000001, "Horizontal angle"=-0.41015237421866746, "Vertical angle"=-0.006981317007977317, "Echo pulse width"=232, "Reserved"=0}, {"flags"=5, "Echo"=1, "Radial distance"=18.35, "Horizontal angle"=-0.41015237421866746, "Vertical angle"=-0.006981317007977317, "Echo pulse width"=204, "Reserved"=0}, {"flags"=4, "Echo"=2, "Radial distance"=23.41, "Horizontal angle"=-0.41015237421866746, "Vertical angle"=-0.006981317007977317, "Echo pulse width"=152, "Reserved"=0}, {"flags"=1, "Echo"=0, "Radial distance"=25.150000000000002, "Horizontal angle"=-0.4145156973486533, "Vertical angle"=0.00698131700797732, "Echo pulse width"=284, "Reserved"=60}, {"flags"=4, "Echo"=1, "Radial distance"=42.410000000000004, "Horizontal angle"=-0.4145156973486533, "Vertical angle"=0.00698131700797732, "Echo pulse width"=156, "Reserved"=0}, {"flags"=1, "Echo"=0, "Radial distance"=61.690000000000005, "Horizontal angle"=-0.4145156973486533, "Vertical angle"=0.020943951023931963, "Echo pulse width"=64, "Reserved"=63}, {"flags"=0, "Echo"=1, "Radial distance"=83.67, "Horizontal angle"=-0.4145156973486533, "Vertical angle"=0.020943951023931963, "Echo pulse width"=100, "Reserved"=64}, {"flags"=4, "Echo"=0, "Radial distance"=12.030000000000001, "Horizontal angle"=-0.41887902047863906, "Vertical angle"=-0.020943951023931952, "Echo pulse width"=260, "Reserved"=0}, {"flags"=5, "Echo"=0, "Radial distance"=15.24, "Horizontal angle"=-0.41887902047863906, "Vertical angle"=-0.006981317007977317, "Echo pulse width"=256, "Reserved"=0}, {"flags"=5, "Echo"=1, "Radial distance"=18.18, "Horizontal angle"=-0.41887902047863906, "Vertical angle"=-0.006981317007977317, "Echo pulse width"=212, "Reserved"=0}, {"flags"=4, "Echo"=2, "Radial distance"=22.73, "Horizontal angle"=-0.41887902047863906, "Vertical angle"=-0.006981317007977317, "Echo pulse width"=144, "Reserved"=0}, {"flags"=5, "Echo"=0, "Radial distance"=25.150000000000002, "Horizontal angle"=-0.4232423436086249, "Vertical angle"=0.00698131700797732, "Echo pulse width"=260, "Reserved"=0}, {"flags"=5, "Echo"=1, "Radial distance"=29.25, "Horizontal angle"=-0.4232423436086249, "Vertical angle"=0.00698131700797732, "Echo pulse width"=92, "Reserved"=0}, {"flags"=4, "Echo"=2, "Radial distance"=42.46, "Horizontal angle"=-0.4232423436086249, "Vertical angle"=0.00698131700797732, "Echo pulse width"=164, "Reserved"=0}, {"flags"=4, "Echo"=0, "Radial distance"=44.550000000000004, "Horizontal angle"=-0.4232423436086249, "Vertical angle"=0.020943951023931963, "Echo pulse width"=164, "Reserved"=0}, {"flags"=4, "Echo"=0, "Radial distance"=11.86, "Horizontal angle"=-0.42760566673861067, "Vertical angle"=-0.020943951023931952, "Echo pulse width"=224, "Reserved"=0}, {"flags"=5, "Echo"=0, "Radial distance"=15.120000000000001, "Horizontal angle"=-0.42760566673861067, "Vertical angle"=-0.006981317007977317, "Echo pulse width"=276, "Reserved"=0}, {"flags"=5, "Echo"=1, "Radial distance"=18.28, "Horizontal angle"=-0.42760566673861067, "Vertical angle"=-0.006981317007977317, "Echo pulse width"=136, "Reserved"=0}, {"flags"=4, "Echo"=2, "Radial distance"=22.29, "Horizontal angle"=-0.42760566673861067, "Vertical angle"=-0.006981317007977317, "Echo pulse width"=148, "Reserved"=0}, {"flags"=5, "Echo"=0, "Radial distance"=24.990000000000002, "Horizontal angle"=-0.4319689898685966, "Vertical angle"=0.00698131700797732, "Echo pulse width"=256, "Reserved"=0}, {"flags"=5, "Echo"=1, "Radial distance"=32.85, "Horizontal angle"=-0.4319689898685966, "Vertical angle"=0.00698131700797732, "Echo pulse width"=92, "Reserved"=0}, {"flags"=4, "Echo"=2, "Radial distance"=42.54, "Horizontal angle"=-0.4319689898685966, "Vertical angle"=0.00698131700797732, "Echo pulse width"=160, "Reserved"=0}, {"flags"=4, "Echo"=0, "Radial distance"=11.55, "Horizontal angle"=-0.4363323129985824, "Vertical angle"=-0.020943951023931952, "Echo pulse width"=260, "Reserved"=0}, {"flags"=0, "Echo"=0, "Radial distance"=12.5, "Horizontal angle"=-0.4363323129985824, "Vertical angle"=-0.006981317007977317, "Echo pulse width"=160, "Reserved"=65}, {"flags"=0, "Echo"=0, "Radial distance"=12.450000000000001, "Horizontal angle"=-0.4406956361285682, "Vertical angle"=0.00698131700797732, "Echo pulse width"=156, "Reserved"=65}, {"flags"=0, "Echo"=0, "Radial distance"=12.47, "Horizontal angle"=-0.4406956361285682, "Vertical angle"=0.020943951023931963, "Echo pulse width"=160, "Reserved"=65}, {"flags"=4, "Echo"=0, "Radial distance"=11.51, "Horizontal angle"=-0.445058959258554, "Vertical angle"=-0.020943951023931952, "Echo pulse width"=248, "Reserved"=0}, {"flags"=0, "Echo"=0, "Radial distance"=12.48, "Horizontal angle"=-0.445058959258554, "Vertical angle"=-0.006981317007977317, "Echo pulse width"=148, "Reserved"=65}, {"flags"=0, "Echo"=0, "Radial distance"=12.5, "Horizontal angle"=-0.4494222823885398, "Vertical angle"=0.00698131700797732, "Echo pulse width"=96, "Reserved"=65}, {"flags"=0, "Echo"=0, "Radial distance"=12.44, "Horizontal angle"=-0.4494222823885398, "Vertical angle"=0.020943951023931963, "Echo pulse width"=104, "Reserved"=65}, {"flags"=4, "Echo"=0, "Radial distance"=11.15, "Horizontal angle"=-0.45378560551852565, "Vertical angle"=-0.020943951023931952, "Echo pulse width"=308, "Reserved"=0}, {"flags"=1, "Echo"=0, "Radial distance"=12.6, "Horizontal angle"=-0.45378560551852565, "Vertical angle"=-0.006981317007977317, "Echo pulse width"=128, "Reserved"=65}, {"flags"=5, "Echo"=1, "Radial distance"=15.76, "Horizontal angle"=-0.45378560551852565, "Vertical angle"=-0.006981317007977317, "Echo pulse width"=272, "Reserved"=0}, {"flags"=4, "Echo"=2, "Radial distance"=18.59, "Horizontal angle"=-0.45378560551852565, "Vertical angle"=-0.006981317007977317, "Echo pulse width"=124, "Reserved"=0}, {"flags"=0, "Echo"=0, "Radial distance"=20.79, "Horizontal angle"=-0.45814892864851153, "Vertical angle"=0.00698131700797732, "Echo pulse width"=192, "Reserved"=66}, {"flags"=0, "Echo"=0, "Radial distance"=20.57, "Horizontal angle"=-0.45814892864851153, "Vertical angle"=0.020943951023931963, "Echo pulse width"=184, "Reserved"=66}, {"flags"=4, "Echo"=0, "Radial distance"=11.15, "Horizontal angle"=-0.4625122517784973, "Vertical angle"=-0.020943951023931952, "Echo pulse width"=288, "Reserved"=0}, {"flags"=5, "Echo"=0, "Radial distance"=14.96, "Horizontal angle"=-0.4625122517784973, "Vertical angle"=-0.006981317007977317, "Echo pulse width"=288, "Reserved"=0}, {"flags"=5, "Echo"=1, "Radial distance"=18.31, "Horizontal angle"=-0.4625122517784973, "Vertical angle"=-0.006981317007977317, "Echo pulse width"=80, "Reserved"=0}, {"flags"=0, "Echo"=2, "Radial distance"=20.45, "Horizontal angle"=-0.4625122517784973, "Vertical angle"=-0.006981317007977317, "Echo pulse width"=144, "Reserved"=66}, {"flags"=0, "Echo"=0, "Radial distance"=20.6, "Horizontal angle"=-0.46687557490848314, "Vertical angle"=0.00698131700797732, "Echo pulse width"=184, "Reserved"=66}, {"flags"=0, "Echo"=0, "Radial distance"=20.400000000000002, "Horizontal angle"=-0.46687557490848314, "Vertical angle"=0.020943951023931963, "Echo pulse width"=180, "Reserved"=66}, {"flags"=4, "Echo"=0, "Radial distance"=10.89, "Horizontal angle"=-0.47123889803846897, "Vertical angle"=-0.020943951023931952, "Echo pulse width"=348, "Reserved"=0}, {"flags"=5, "Echo"=0, "Radial distance"=14.290000000000001, "Horizontal angle"=-0.47123889803846897, "Vertical angle"=-0.006981317007977317, "Echo pulse width"=344, "Reserved"=0}, {"flags"=5, "Echo"=1, "Radial distance"=18.11, "Horizontal angle"=-0.47123889803846897, "Vertical angle"=-0.006981317007977317, "Echo pulse width"=64, "Reserved"=0}, {"flags"=4, "Echo"=2, "Radial distance"=20.09, "Horizontal angle"=-0.47123889803846897, "Vertical angle"=-0.006981317007977317, "Echo pulse width"=152, "Reserved"=0}, {"flags"=0, "Echo"=0, "Radial distance"=20.48, "Horizontal angle"=-0.47560222116845474, "Vertical angle"=0.00698131700797732, "Echo pulse width"=184, "Reserved"=66}, {"flags"=0, "Echo"=0, "Radial distance"=20.400000000000002, "Horizontal angle"=-0.47560222116845474, "Vertical angle"=0.020943951023931963, "Echo pulse width"=180, "Reserved"=66}, {"flags"=4, "Echo"=0, "Radial distance"=10.950000000000001, "Horizontal angle"=-0.4799655442984406, "Vertical angle"=-0.020943951023931952, "Echo pulse width"=288, "Reserved"=0}, {"flags"=5, "Echo"=0, "Radial distance"=14.88, "Horizontal angle"=-0.4799655442984406, "Vertical angle"=-0.006981317007977317, "Echo pulse width"=280, "Reserved"=0}, {"flags"=5, "Echo"=1, "Radial distance"=16.87, "Horizontal angle"=-0.4799655442984406, "Vertical angle"=-0.006981317007977317, "Echo pulse width"=44, "Reserved"=0}, {"flags"=4, "Echo"=2, "Radial distance"=17.93, "Horizontal angle"=-0.4799655442984406, "Vertical angle"=-0.006981317007977317, "Echo pulse width"=48, "Reserved"=0}, {"flags"=0, "Echo"=0, "Radial distance"=20.5, "Horizontal angle"=-0.48432886742842646, "Vertical angle"=0.00698131700797732, "Echo pulse width"=200, "Reserved"=66}, {"flags"=0, "Echo"=0, "Radial distance"=20.400000000000002, "Horizontal angle"=-0.48432886742842646, "Vertical angle"=0.020943951023931963, "Echo pulse width"=180, "Reserved"=66}, {"flags"=4, "Echo"=0, "Radial distance"=10.69, "Horizontal angle"=-0.4886921905584123, "Vertical angle"=-0.020943951023931952, "Echo pulse width"=344, "Reserved"=0}, {"flags"=5, "Echo"=0, "Radial distance"=14.09, "Horizontal angle"=-0.4886921905584123, "Vertical angle"=-0.006981317007977317, "Echo pulse width"=404, "Reserved"=0}, {"flags"=4, "Echo"=1, "Radial distance"=19.37, "Horizontal angle"=-0.4886921905584123, "Vertical angle"=-0.006981317007977317, "Echo pulse width"=152, "Reserved"=0}, {"flags"=0, "Echo"=0, "Radial distance"=20.38, "Horizontal angle"=-0.49305551368839806, "Vertical angle"=0.00698131700797732, "Echo pulse width"=240, "Reserved"=66}, {"flags"=0, "Echo"=0, "Radial distance"=20.52, "Horizontal angle"=-0.49305551368839806, "Vertical angle"=0.020943951023931963, "Echo pulse width"=176, "Reserved"=66}, {"flags"=4, "Echo"=0, "Radial distance"=10.790000000000001, "Horizontal angle"=-0.4974188368183839, "Vertical angle"=-0.020943951023931952, "Echo pulse width"=288, "Reserved"=0}, {"flags"=5, "Echo"=0, "Radial distance"=14.55, "Horizontal angle"=-0.4974188368183839, "Vertical angle"=-0.006981317007977317, "Echo pulse width"=328, "Reserved"=0}, {"flags"=4, "Echo"=1, "Radial distance"=19.01, "Horizontal angle"=-0.4974188368183839, "Vertical angle"=-0.006981317007977317, "Echo pulse width"=156, "Reserved"=0}, {"flags"=5, "Echo"=0, "Radial distance"=20.11, "Horizontal angle"=-0.5017821599483697, "Vertical angle"=0.00698131700797732, "Echo pulse width"=344, "Reserved"=0}, {"flags"=5, "Echo"=1, "Radial distance"=24.560000000000002, "Horizontal angle"=-0.5017821599483697, "Vertical angle"=0.00698131700797732, "Echo pulse width"=80, "Reserved"=0}, {"flags"=4, "Echo"=2, "Radial distance"=30.28, "Horizontal angle"=-0.5017821599483697, "Vertical angle"=0.00698131700797732, "Echo pulse width"=188, "Reserved"=0}, {"flags"=5, "Echo"=0, "Radial distance"=20.84, "Horizontal angle"=-0.5017821599483697, "Vertical angle"=0.020943951023931963, "Echo pulse width"=168, "Reserved"=0}, {"flags"=5, "Echo"=1, "Radial distance"=31.61, "Horizontal angle"=-0.5017821599483697, "Vertical angle"=0.020943951023931963, "Echo pulse width"=76, "Reserved"=0}, {"flags"=4, "Echo"=2, "Radial distance"=33.15, "Horizontal angle"=-0.5017821599483697, "Vertical angle"=0.020943951023931963, "Echo pulse width"=112, "Reserved"=0}, {"flags"=4, "Echo"=0, "Radial distance"=10.53, "Horizontal angle"=-0.5061454830783556, "Vertical angle"=-0.020943951023931952, "Echo pulse width"=344, "Reserved"=0}, {"flags"=5, "Echo"=0, "Radial distance"=13.85, "Horizontal angle"=-0.5061454830783556, "Vertical angle"=-0.006981317007977317, "Echo pulse width"=452, "Reserved"=0}, {"flags"=4, "Echo"=1, "Radial distance"=18.650000000000002, "Horizontal angle"=-0.5061454830783556, "Vertical angle"=-0.006981317007977317, "Echo pulse width"=156, "Reserved"=0}, {"flags"=5, "Echo"=0, "Radial distance"=19.55, "Horizontal angle"=-0.5105088062083414, "Vertical angle"=0.00698131700797732, "Echo pulse width"=176, "Reserved"=0}, {"flags"=5, "Echo"=1, "Radial distance"=21.330000000000002, "Horizontal angle"=-0.5105088062083414, "Vertical angle"=0.00698131700797732, "Echo pulse width"=88, "Reserved"=0}, {"flags"=4, "Echo"=2, "Radial distance"=23.81, "Horizontal angle"=-0.5105088062083414, "Vertical angle"=0.00698131700797732, "Echo pulse width"=120, "Reserved"=0}, {"flags"=4, "Echo"=0, "Radial distance"=31.68, "Horizontal angle"=-0.5105088062083414, "Vertical angle"=0.020943951023931963, "Echo pulse width"=220, "Reserved"=0}, {"flags"=4, "Echo"=0, "Radial distance"=10.51, "Horizontal angle"=-0.5148721293383272, "Vertical angle"=-0.020943951023931952, "Echo pulse width"=288, "Reserved"=0}, {"flags"=5, "Echo"=0, "Radial distance"=14.280000000000001, "Horizontal angle"=-0.5148721293383272, "Vertical angle"=-0.006981317007977317, "Echo pulse width"=364, "Reserved"=0}, {"flags"=4, "Echo"=1, "Radial distance"=18.37, "Horizontal angle"=-0.5148721293383272, "Vertical angle"=-0.006981317007977317, "Echo pulse width"=148, "Reserved"=0}, {"flags"=5, "Echo"=0, "Radial distance"=19.23, "Horizontal angle"=-0.519235452468313, "Vertical angle"=0.00698131700797732, "Echo pulse width"=192, "Reserved"=0}, {"flags"=5, "Echo"=1, "Radial distance"=23.71, "Horizontal angle"=-0.519235452468313, "Vertical angle"=0.00698131700797732, "Echo pulse width"=140, "Reserved"=0}, {"flags"=4, "Echo"=2, "Radial distance"=30.400000000000002, "Horizontal angle"=-0.519235452468313, "Vertical angle"=0.00698131700797732, "Echo pulse width"=188, "Reserved"=0}, {"flags"=4, "Echo"=0, "Radial distance"=31.64, "Horizontal angle"=-0.519235452468313, "Vertical angle"=0.020943951023931963, "Echo pulse width"=216, "Reserved"=0}, {"flags"=4, "Echo"=0, "Radial distance"=10.31, "Horizontal angle"=-0.5235987755982988, "Vertical angle"=-0.020943951023931952, "Echo pulse width"=340, "Reserved"=0}, {"flags"=5, "Echo"=0, "Radial distance"=13.57, "Horizontal angle"=-0.5235987755982988, "Vertical angle"=-0.006981317007977317, "Echo pulse width"=428, "Reserved"=0}, {"flags"=4, "Echo"=1, "Radial distance"=18.05, "Horizontal angle"=-0.5235987755982988, "Vertical angle"=-0.006981317007977317, "Echo pulse width"=156, "Reserved"=0}, {"flags"=5, "Echo"=0, "Radial distance"=18.88, "Horizontal angle"=-0.5279620987282847, "Vertical angle"=0.00698131700797732, "Echo pulse width"=228, "Reserved"=0}, {"flags"=5, "Echo"=1, "Radial distance"=23.35, "Horizontal angle"=-0.5279620987282847, "Vertical angle"=0.00698131700797732, "Echo pulse width"=104, "Reserved"=0}, {"flags"=4, "Echo"=2, "Radial distance"=30.34, "Horizontal angle"=-0.5279620987282847, "Vertical angle"=0.00698131700797732, "Echo pulse width"=204, "Reserved"=0}, {"flags"=4, "Echo"=0, "Radial distance"=31.66, "Horizontal angle"=-0.5279620987282847, "Vertical angle"=0.020943951023931963, "Echo pulse width"=212, "Reserved"=0}, {"flags"=4, "Echo"=0, "Radial distance"=10.39, "Horizontal angle"=-0.5323254218582705, "Vertical angle"=-0.020943951023931952, "Echo pulse width"=288, "Reserved"=0}, {"flags"=5, "Echo"=0, "Radial distance"=14.51, "Horizontal angle"=-0.5323254218582705, "Vertical angle"=-0.006981317007977317, "Echo pulse width"=316, "Reserved"=0}, {"flags"=4, "Echo"=1, "Radial distance"=17.66, "Horizontal angle"=-0.5323254218582705, "Vertical angle"=-0.006981317007977317, "Echo pulse width"=164, "Reserved"=0}, {"flags"=5, "Echo"=0, "Radial distance"=18.67, "Horizontal angle"=-0.5366887449882564, "Vertical angle"=0.00698131700797732, "Echo pulse width"=248, "Reserved"=0}, {"flags"=4, "Echo"=1, "Radial distance"=30.51, "Horizontal angle"=-0.5366887449882564, "Vertical angle"=0.00698131700797732, "Echo pulse width"=176, "Reserved"=0}, {"flags"=5, "Echo"=0, "Radial distance"=31.76, "Horizontal angle"=-0.5366887449882564, "Vertical angle"=0.020943951023931963, "Echo pulse width"=200, "Reserved"=0}, {"flags"=4, "Echo"=1, "Radial distance"=41.42, "Horizontal angle"=-0.5366887449882564, "Vertical angle"=0.020943951023931963, "Echo pulse width"=84, "Reserved"=0}, {"flags"=4, "Echo"=0, "Radial distance"=10.13, "Horizontal angle"=-0.5410520681182421, "Vertical angle"=-0.020943951023931952, "Echo pulse width"=348, "Reserved"=0}, {"flags"=4, "Echo"=0, "Radial distance"=13.49, "Horizontal angle"=-0.5410520681182421, "Vertical angle"=-0.006981317007977317, "Echo pulse width"=576, "Reserved"=0}, {"flags"=5, "Echo"=0, "Radial distance"=18.43, "Horizontal angle"=-0.5454153912482279, "Vertical angle"=0.00698131700797732, "Echo pulse width"=252, "Reserved"=0}, {"flags"=4, "Echo"=1, "Radial distance"=30.55, "Horizontal angle"=-0.5454153912482279, "Vertical angle"=0.00698131700797732, "Echo pulse width"=176, "Reserved"=0}, {"flags"=5, "Echo"=0, "Radial distance"=31.92, "Horizontal angle"=-0.5454153912482279, "Vertical angle"=0.020943951023931963, "Echo pulse width"=204, "Reserved"=0}, {"flags"=4, "Echo"=1, "Radial distance"=41.480000000000004, "Horizontal angle"=-0.5454153912482279, "Vertical angle"=0.020943951023931963, "Echo pulse width"=124, "Reserved"=0}, {"flags"=4, "Echo"=0, "Radial distance"=10.19, "Horizontal angle"=-0.5497787143782138, "Vertical angle"=-0.020943951023931952, "Echo pulse width"=296, "Reserved"=0}, {"flags"=4, "Echo"=0, "Radial distance"=14.120000000000001, "Horizontal angle"=-0.5497787143782138, "Vertical angle"=-0.006981317007977317, "Echo pulse width"=480, "Reserved"=0}, {"flags"=5, "Echo"=0, "Radial distance"=18.31, "Horizontal angle"=-0.5541420375081997, "Vertical angle"=0.00698131700797732, "Echo pulse width"=252, "Reserved"=0}, {"flags"=4, "Echo"=1, "Radial distance"=30.84, "Horizontal angle"=-0.5541420375081997, "Vertical angle"=0.00698131700797732, "Echo pulse width"=148, "Reserved"=0}, {"flags"=5, "Echo"=0, "Radial distance"=32.19, "Horizontal angle"=-0.5541420375081997, "Vertical angle"=0.020943951023931963, "Echo pulse width"=156, "Reserved"=0}, {"flags"=4, "Echo"=1, "Radial distance"=40.42, "Horizontal angle"=-0.5541420375081997, "Vertical angle"=0.020943951023931963, "Echo pulse width"=108, "Reserved"=0}, {"flags"=4, "Echo"=0, "Radial distance"=10.01, "Horizontal angle"=-0.5585053606381855, "Vertical angle"=-0.020943951023931952, "Echo pulse width"=344, "Reserved"=0}, {"flags"=5, "Echo"=0, "Radial distance"=13.17, "Horizontal angle"=-0.5585053606381855, "Vertical angle"=-0.006981317007977317, "Echo pulse width"=380, "Reserved"=0}, {"flags"=4, "Echo"=1, "Radial distance"=16.94, "Horizontal angle"=-0.5585053606381855, "Vertical angle"=-0.006981317007977317, "Echo pulse width"=160, "Reserved"=0}, {"flags"=4, "Echo"=0, "Radial distance"=16.67, "Horizontal angle"=-0.5628686837681712, "Vertical angle"=0.00698131700797732, "Echo pulse width"=364, "Reserved"=0}, {"flags"=0, "Echo"=0, "Radial distance"=16.37, "Horizontal angle"=-0.5628686837681712, "Vertical angle"=0.020943951023931963, "Echo pulse width"=188, "Reserved"=67}, {"flags"=4, "Echo"=0, "Radial distance"=10.19, "Horizontal angle"=-0.5672320068981571, "Vertical angle"=-0.020943951023931952, "Echo pulse width"=284, "Reserved"=0}, {"flags"=4, "Echo"=0, "Radial distance"=13.64, "Horizontal angle"=-0.5672320068981571, "Vertical angle"=-0.006981317007977317, "Echo pulse width"=476, "Reserved"=0}, {"flags"=0, "Echo"=0, "Radial distance"=16.39, "Horizontal angle"=-0.5715953300281429, "Vertical angle"=0.00698131700797732, "Echo pulse width"=196, "Reserved"=67}, {"flags"=0, "Echo"=0, "Radial distance"=16.17, "Horizontal angle"=-0.5715953300281429, "Vertical angle"=0.020943951023931963, "Echo pulse width"=188, "Reserved"=67}, {"flags"=4, "Echo"=0, "Radial distance"=9.99, "Horizontal angle"=-0.5759586531581287, "Vertical angle"=-0.020943951023931952, "Echo pulse width"=336, "Reserved"=0}, {"flags"=5, "Echo"=0, "Radial distance"=13.05, "Horizontal angle"=-0.5759586531581287, "Vertical angle"=-0.006981317007977317, "Echo pulse width"=336, "Reserved"=0}, {"flags"=0, "Echo"=1, "Radial distance"=16.38, "Horizontal angle"=-0.5759586531581287, "Vertical angle"=-0.006981317007977317, "Echo pulse width"=160, "Reserved"=67}, {"flags"=0, "Echo"=0, "Radial distance"=16.23, "Horizontal angle"=-0.5803219762881145, "Vertical angle"=0.00698131700797732, "Echo pulse width"=192, "Reserved"=67}, {"flags"=0, "Echo"=0, "Radial distance"=16.01, "Horizontal angle"=-0.5803219762881145, "Vertical angle"=0.020943951023931963, "Echo pulse width"=184, "Reserved"=67}, {"flags"=4, "Echo"=0, "Radial distance"=9.99, "Horizontal angle"=-0.5846852994181004, "Vertical angle"=-0.020943951023931952, "Echo pulse width"=288, "Reserved"=0}, {"flags"=4, "Echo"=0, "Radial distance"=13.32, "Horizontal angle"=-0.5846852994181004, "Vertical angle"=-0.006981317007977317, "Echo pulse width"=460, "Reserved"=0}, {"flags"=0, "Echo"=0, "Radial distance"=16.240000000000002, "Horizontal angle"=-0.5890486225480862, "Vertical angle"=0.00698131700797732, "Echo pulse width"=188, "Reserved"=67}, {"flags"=0, "Echo"=0, "Radial distance"=15.97, "Horizontal angle"=-0.5890486225480862, "Vertical angle"=0.020943951023931963, "Echo pulse width"=188, "Reserved"=67}, {"flags"=4, "Echo"=0, "Radial distance"=9.77, "Horizontal angle"=-0.593411945678072, "Vertical angle"=-0.020943951023931952, "Echo pulse width"=344, "Reserved"=0}, {"flags"=4, "Echo"=0, "Radial distance"=12.81, "Horizontal angle"=-0.593411945678072, "Vertical angle"=-0.006981317007977317, "Echo pulse width"=492, "Reserved"=0}, {"flags"=0, "Echo"=0, "Radial distance"=16.16, "Horizontal angle"=-0.5977752688080579, "Vertical angle"=0.00698131700797732, "Echo pulse width"=184, "Reserved"=67}, {"flags"=0, "Echo"=0, "Radial distance"=15.97, "Horizontal angle"=-0.5977752688080579, "Vertical angle"=0.020943951023931963, "Echo pulse width"=188, "Reserved"=67}, {"flags"=4, "Echo"=0, "Radial distance"=9.83, "Horizontal angle"=-0.6021385919380438, "Vertical angle"=-0.020943951023931952, "Echo pulse width"=284, "Reserved"=0}, {"flags"=4, "Echo"=0, "Radial distance"=12.96, "Horizontal angle"=-0.6021385919380438, "Vertical angle"=-0.006981317007977317, "Echo pulse width"=456, "Reserved"=0}, {"flags"=0, "Echo"=0, "Radial distance"=16.23, "Horizontal angle"=-0.6065019150680295, "Vertical angle"=0.00698131700797732, "Echo pulse width"=192, "Reserved"=67}, {"flags"=0, "Echo"=0, "Radial distance"=16.05, "Horizontal angle"=-0.6065019150680295, "Vertical angle"=0.020943951023931963, "Echo pulse width"=188, "Reserved"=67}, {"flags"=4, "Echo"=0, "Radial distance"=9.67, "Horizontal angle"=-0.6108652381980153, "Vertical angle"=-0.020943951023931952, "Echo pulse width"=340, "Reserved"=0}, {"flags"=4, "Echo"=0, "Radial distance"=12.69, "Horizontal angle"=-0.6108652381980153, "Vertical angle"=-0.006981317007977317, "Echo pulse width"=480, "Reserved"=0}, {"flags"=0, "Echo"=0, "Radial distance"=16.240000000000002, "Horizontal angle"=-0.6152285613280012, "Vertical angle"=0.00698131700797732, "Echo pulse width"=188, "Reserved"=67}, {"flags"=0, "Echo"=0, "Radial distance"=16.04, "Horizontal angle"=-0.6152285613280012, "Vertical angle"=0.020943951023931963, "Echo pulse width"=180, "Reserved"=67}, {"flags"=4, "Echo"=0, "Radial distance"=9.790000000000001, "Horizontal angle"=-0.619591884457987, "Vertical angle"=-0.020943951023931952, "Echo pulse width"=284, "Reserved"=0}, {"flags"=4, "Echo"=0, "Radial distance"=12.84, "Horizontal angle"=-0.619591884457987, "Vertical angle"=-0.006981317007977317, "Echo pulse width"=440, "Reserved"=0}, {"flags"=0, "Echo"=0, "Radial distance"=16.39, "Horizontal angle"=-0.6239552075879727, "Vertical angle"=0.00698131700797732, "Echo pulse width"=192, "Reserved"=67}, {"flags"=0, "Echo"=0, "Radial distance"=16.17, "Horizontal angle"=-0.6239552075879727, "Vertical angle"=0.020943951023931963, "Echo pulse width"=184, "Reserved"=67}, {"flags"=4, "Echo"=0, "Radial distance"=9.59, "Horizontal angle"=-0.6283185307179586, "Vertical angle"=-0.020943951023931952, "Echo pulse width"=340, "Reserved"=0}, {"flags"=4, "Echo"=0, "Radial distance"=12.61, "Horizontal angle"=-0.6283185307179586, "Vertical angle"=-0.006981317007977317, "Echo pulse width"=468, "Reserved"=0}, {"flags"=5, "Echo"=0, "Radial distance"=17.150000000000002, "Horizontal angle"=-0.6326818538479445, "Vertical angle"=0.00698131700797732, "Echo pulse width"=380, "Reserved"=0}, {"flags"=4, "Echo"=1, "Radial distance"=26.13, "Horizontal angle"=-0.6326818538479445, "Vertical angle"=0.00698131700797732, "Echo pulse width"=88, "Reserved"=0}, {"flags"=0, "Echo"=0, "Radial distance"=16.36, "Horizontal angle"=-0.6326818538479445, "Vertical angle"=0.020943951023931963, "Echo pulse width"=180, "Reserved"=67}, {"flags"=4, "Echo"=0, "Radial distance"=9.67, "Horizontal angle"=-0.6370451769779303, "Vertical angle"=-0.020943951023931952, "Echo pulse width"=300, "Reserved"=0}, {"flags"=4, "Echo"=0, "Radial distance"=12.72, "Horizontal angle"=-0.6370451769779303, "Vertical angle"=-0.006981317007977317, "Echo pulse width"=432, "Reserved"=0}, {"flags"=5, "Echo"=0, "Radial distance"=16.990000000000002, "Horizontal angle"=-0.6414085001079161, "Vertical angle"=0.00698131700797732, "Echo pulse width"=288, "Reserved"=0}, {"flags"=4, "Echo"=1, "Radial distance"=25.72, "Horizontal angle"=-0.6414085001079161, "Vertical angle"=0.00698131700797732, "Echo pulse width"=60, "Reserved"=0}, {"flags"=4, "Echo"=0, "Radial distance"=9.450000000000001, "Horizontal angle"=-0.6457718232379019, "Vertical angle"=-0.020943951023931952, "Echo pulse width"=352, "Reserved"=0}, {"flags"=4, "Echo"=0, "Radial distance"=12.49, "Horizontal angle"=-0.6457718232379019, "Vertical angle"=-0.006981317007977317, "Echo pulse width"=456, "Reserved"=0}, {"flags"=5, "Echo"=0, "Radial distance"=16.87, "Horizontal angle"=-0.6501351463678877, "Vertical angle"=0.00698131700797732, "Echo pulse width"=384, "Reserved"=0}, {"flags"=5, "Echo"=1, "Radial distance"=25.48, "Horizontal angle"=-0.6501351463678877, "Vertical angle"=0.00698131700797732, "Echo pulse width"=68, "Reserved"=0}, {"flags"=4, "Echo"=2, "Radial distance"=26.84, "Horizontal angle"=-0.6501351463678877, "Vertical angle"=0.00698131700797732, "Echo pulse width"=84, "Reserved"=0}, {"flags"=4, "Echo"=0, "Radial distance"=9.55, "Horizontal angle"=-0.6544984694978736, "Vertical angle"=-0.020943951023931952, "Echo pulse width"=300, "Reserved"=0}, {"flags"=4, "Echo"=0, "Radial distance"=12.64, "Horizontal angle"=-0.6544984694978736, "Vertical angle"=-0.006981317007977317, "Echo pulse width"=424, "Reserved"=0}, {"flags"=4, "Echo"=0, "Radial distance"=16.55, "Horizontal angle"=-0.6588617926278594, "Vertical angle"=0.00698131700797732, "Echo pulse width"=424, "Reserved"=0}, {"flags"=4, "Echo"=0, "Radial distance"=9.33, "Horizontal angle"=-0.6632251157578453, "Vertical angle"=-0.020943951023931952, "Echo pulse width"=352, "Reserved"=0}, {"flags"=4, "Echo"=0, "Radial distance"=12.290000000000001, "Horizontal angle"=-0.6632251157578453, "Vertical angle"=-0.006981317007977317, "Echo pulse width"=448, "Reserved"=0}, {"flags"=4, "Echo"=0, "Radial distance"=16.55, "Horizontal angle"=-0.667588438887831, "Vertical angle"=0.00698131700797732, "Echo pulse width"=396, "Reserved"=0}, {"flags"=0, "Echo"=0, "Radial distance"=76.51, "Horizontal angle"=-0.667588438887831, "Vertical angle"=0.020943951023931963, "Echo pulse width"=96, "Reserved"=68}, {"flags"=4, "Echo"=0, "Radial distance"=9.47, "Horizontal angle"=-0.6719517620178168, "Vertical angle"=-0.020943951023931952, "Echo pulse width"=296, "Reserved"=0}, {"flags"=4, "Echo"=0, "Radial distance"=12.48, "Horizontal angle"=-0.6719517620178168, "Vertical angle"=-0.006981317007977317, "Echo pulse width"=396, "Reserved"=0}, {"flags"=4, "Echo"=0, "Radial distance"=16.31, "Horizontal angle"=-0.6763150851478027, "Vertical angle"=0.00698131700797732, "Echo pulse width"=388, "Reserved"=0}, {"flags"=0, "Echo"=0, "Radial distance"=84.49, "Horizontal angle"=-0.6763150851478027, "Vertical angle"=0.020943951023931963, "Echo pulse width"=72, "Reserved"=69}, {"flags"=4, "Echo"=0, "Radial distance"=9.290000000000001, "Horizontal angle"=-0.6806784082777886, "Vertical angle"=-0.020943951023931952, "Echo pulse width"=344, "Reserved"=0}, {"flags"=4, "Echo"=0, "Radial distance"=12.25, "Horizontal angle"=-0.6806784082777886, "Vertical angle"=-0.006981317007977317, "Echo pulse width"=424, "Reserved"=0}, {"flags"=4, "Echo"=0, "Radial distance"=15.99, "Horizontal angle"=-0.6850417314077744, "Vertical angle"=0.00698131700797732, "Echo pulse width"=432, "Reserved"=0}, {"flags"=4, "Echo"=0, "Radial distance"=9.35, "Horizontal angle"=-0.6894050545377601, "Vertical angle"=-0.020943951023931952, "Echo pulse width"=296, "Reserved"=0}, {"flags"=4, "Echo"=0, "Radial distance"=12.48, "Horizontal angle"=-0.6894050545377601, "Vertical angle"=-0.006981317007977317, "Echo pulse width"=380, "Reserved"=0}, {"flags"=5, "Echo"=0, "Radial distance"=15.870000000000001, "Horizontal angle"=-0.6937683776677459, "Vertical angle"=0.00698131700797732, "Echo pulse width"=400, "Reserved"=0}, {"flags"=4, "Echo"=1, "Radial distance"=21.39, "Horizontal angle"=-0.6937683776677459, "Vertical angle"=0.00698131700797732, "Echo pulse width"=108, "Reserved"=0}, {"flags"=4, "Echo"=0, "Radial distance"=9.19, "Horizontal angle"=-0.6981317007977318, "Vertical angle"=-0.020943951023931952, "Echo pulse width"=332, "Reserved"=0}, {"flags"=4, "Echo"=0, "Radial distance"=12.09, "Horizontal angle"=-0.6981317007977318, "Vertical angle"=-0.006981317007977317, "Echo pulse width"=416, "Reserved"=0}, {"flags"=4, "Echo"=0, "Radial distance"=15.75, "Horizontal angle"=-0.7024950239277177, "Vertical angle"=0.00698131700797732, "Echo pulse width"=412, "Reserved"=0}, {"flags"=4, "Echo"=0, "Radial distance"=9.19, "Horizontal angle"=-0.7068583470577035, "Vertical angle"=-0.020943951023931952, "Echo pulse width"=292, "Reserved"=0}, {"flags"=4, "Echo"=0, "Radial distance"=12.24, "Horizontal angle"=-0.7068583470577035, "Vertical angle"=-0.006981317007977317, "Echo pulse width"=372, "Reserved"=0}, {"flags"=5, "Echo"=0, "Radial distance"=15.67, "Horizontal angle"=-0.7112216701876892, "Vertical angle"=0.00698131700797732, "Echo pulse width"=384, "Reserved"=0}, {"flags"=5, "Echo"=1, "Radial distance"=21.22, "Horizontal angle"=-0.7112216701876892, "Vertical angle"=0.00698131700797732, "Echo pulse width"=36, "Reserved"=0}, {"flags"=4, "Echo"=2, "Radial distance"=25.09, "Horizontal angle"=-0.7112216701876892, "Vertical angle"=0.00698131700797732, "Echo pulse width"=112, "Reserved"=0}, {"flags"=4, "Echo"=0, "Radial distance"=9.07, "Horizontal angle"=-0.7155849933176751, "Vertical angle"=-0.020943951023931952, "Echo pulse width"=332, "Reserved"=0}, {"flags"=4, "Echo"=0, "Radial distance"=11.85, "Horizontal angle"=-0.7155849933176751, "Vertical angle"=-0.006981317007977317, "Echo pulse width"=412, "Reserved"=0}, {"flags"=5, "Echo"=0, "Radial distance"=15.39, "Horizontal angle"=-0.7199483164476609, "Vertical angle"=0.00698131700797732, "Echo pulse width"=352, "Reserved"=0}, {"flags"=4, "Echo"=1, "Radial distance"=24.77, "Horizontal angle"=-0.7199483164476609, "Vertical angle"=0.00698131700797732, "Echo pulse width"=156, "Reserved"=0}, {"flags"=4, "Echo"=0, "Radial distance"=25.89, "Horizontal angle"=-0.7199483164476609, "Vertical angle"=0.020943951023931963, "Echo pulse width"=72, "Reserved"=0}, {"flags"=4, "Echo"=0, "Radial distance"=9.07, "Horizontal angle"=-0.7243116395776468, "Vertical angle"=-0.020943951023931952, "Echo pulse width"=288, "Reserved"=0}, {"flags"=4, "Echo"=0, "Radial distance"=12.120000000000001, "Horizontal angle"=-0.7243116395776468, "Vertical angle"=-0.006981317007977317, "Echo pulse width"=360, "Reserved"=0}, {"flags"=5, "Echo"=0, "Radial distance"=15.11, "Horizontal angle"=-0.7286749627076325, "Vertical angle"=0.00698131700797732, "Echo pulse width"=376, "Reserved"=0}, {"flags"=5, "Echo"=1, "Radial distance"=21.26, "Horizontal angle"=-0.7286749627076325, "Vertical angle"=0.00698131700797732, "Echo pulse width"=36, "Reserved"=0}, {"flags"=4, "Echo"=2, "Radial distance"=24.35, "Horizontal angle"=-0.7286749627076325, "Vertical angle"=0.00698131700797732, "Echo pulse width"=136, "Reserved"=0}, {"flags"=4, "Echo"=0, "Radial distance"=25.76, "Horizontal angle"=-0.7286749627076325, "Vertical angle"=0.020943951023931963, "Echo pulse width"=192, "Reserved"=0}, {"flags"=4, "Echo"=0, "Radial distance"=8.950000000000001, "Horizontal angle"=-0.7330382858376184, "Vertical angle"=-0.020943951023931952, "Echo pulse width"=332, "Reserved"=0}, {"flags"=4, "Echo"=0, "Radial distance"=11.85, "Horizontal angle"=-0.7330382858376184, "Vertical angle"=-0.006981317007977317, "Echo pulse width"=392, "Reserved"=0}, {"flags"=5, "Echo"=0, "Radial distance"=15.15, "Horizontal angle"=-0.7374016089676042, "Vertical angle"=0.00698131700797732, "Echo pulse width"=368, "Reserved"=0}, {"flags"=5, "Echo"=1, "Radial distance"=19.61, "Horizontal angle"=-0.7374016089676042, "Vertical angle"=0.00698131700797732, "Echo pulse width"=92, "Reserved"=0}, {"flags"=4, "Echo"=2, "Radial distance"=24.13, "Horizontal angle"=-0.7374016089676042, "Vertical angle"=0.00698131700797732, "Echo pulse width"=124, "Reserved"=0}, {"flags"=4, "Echo"=0, "Radial distance"=25.240000000000002, "Horizontal angle"=-0.7374016089676042, "Vertical angle"=0.020943951023931963, "Echo pulse width"=252, "Reserved"=0}, {"flags"=4, "Echo"=0, "Radial distance"=8.950000000000001, "Horizontal angle"=-0.74176493209759, "Vertical angle"=-0.020943951023931952, "Echo pulse width"=284, "Reserved"=0}, {"flags"=4, "Echo"=0, "Radial distance"=11.92, "Horizontal angle"=-0.74176493209759, "Vertical angle"=-0.006981317007977317, "Echo pulse width"=348, "Reserved"=0}, {"flags"=5, "Echo"=0, "Radial distance"=14.870000000000001, "Horizontal angle"=-0.7461282552275759, "Vertical angle"=0.00698131700797732, "Echo pulse width"=376, "Reserved"=0}, {"flags"=5, "Echo"=1, "Radial distance"=19.37, "Horizontal angle"=-0.7461282552275759, "Vertical angle"=0.00698131700797732, "Echo pulse width"=124, "Reserved"=0}, {"flags"=4, "Echo"=2, "Radial distance"=23.97, "Horizontal angle"=-0.7461282552275759, "Vertical angle"=0.00698131700797732, "Echo pulse width"=120, "Reserved"=0}, {"flags"=4, "Echo"=0, "Radial distance"=24.92, "Horizontal angle"=-0.7461282552275759, "Vertical angle"=0.020943951023931963, "Echo pulse width"=276, "Reserved"=0}, {"flags"=4, "Echo"=0, "Radial distance"=8.83, "Horizontal angle"=-0.7504915783575618, "Vertical angle"=-0.020943951023931952, "Echo pulse width"=324, "Reserved"=0}, {"flags"=4, "Echo"=0, "Radial distance"=11.65, "Horizontal angle"=-0.7504915783575618, "Vertical angle"=-0.006981317007977317, "Echo pulse width"=368, "Reserved"=0}, {"flags"=5, "Echo"=0, "Radial distance"=14.790000000000001, "Horizontal angle"=-0.7548549014875475, "Vertical angle"=0.00698131700797732, "Echo pulse width"=392, "Reserved"=0}, {"flags"=5, "Echo"=1, "Radial distance"=19.07, "Horizontal angle"=-0.7548549014875475, "Vertical angle"=0.00698131700797732, "Echo pulse width"=104, "Reserved"=0}, {"flags"=4, "Echo"=2, "Radial distance"=23.75, "Horizontal angle"=-0.7548549014875475, "Vertical angle"=0.00698131700797732, "Echo pulse width"=108, "Reserved"=0}, {"flags"=4, "Echo"=0, "Radial distance"=24.63, "Horizontal angle"=-0.7548549014875475, "Vertical angle"=0.020943951023931963, "Echo pulse width"=236, "Reserved"=0}, {"flags"=4, "Echo"=0, "Radial distance"=8.870000000000001, "Horizontal angle"=-0.7592182246175333, "Vertical angle"=-0.020943951023931952, "Echo pulse width"=280, "Reserved"=0}, {"flags"=4, "Echo"=0, "Radial distance"=11.790000000000001, "Horizontal angle"=-0.7592182246175333, "Vertical angle"=-0.006981317007977317, "Echo pulse width"=296, "Reserved"=0}, {"flags"=5, "Echo"=0, "Radial distance"=14.64, "Horizontal angle"=-0.7635815477475192, "Vertical angle"=0.00698131700797732, "Echo pulse width"=352, "Reserved"=0}, {"flags"=5, "Echo"=1, "Radial distance"=19.36, "Horizontal angle"=-0.7635815477475192, "Vertical angle"=0.00698131700797732, "Echo pulse width"=208, "Reserved"=0}, {"flags"=4, "Echo"=2, "Radial distance"=23.62, "Horizontal angle"=-0.7635815477475192, "Vertical angle"=0.00698131700797732, "Echo pulse width"=100, "Reserved"=0}, {"flags"=1, "Echo"=0, "Radial distance"=12.46, "Horizontal angle"=-0.7635815477475192, "Vertical angle"=0.020943951023931963, "Echo pulse width"=140, "Reserved"=70}, {"flags"=4, "Echo"=1, "Radial distance"=24.11, "Horizontal angle"=-0.7635815477475192, "Vertical angle"=0.020943951023931963, "Echo pulse width"=160, "Reserved"=0}, {"flags"=4, "Echo"=0, "Radial distance"=8.71, "Horizontal angle"=-0.767944870877505, "Vertical angle"=-0.020943951023931952, "Echo pulse width"=328, "Reserved"=0}, {"flags"=4, "Echo"=0, "Radial distance"=11.48, "Horizontal angle"=-0.767944870877505, "Vertical angle"=-0.006981317007977317, "Echo pulse width"=320, "Reserved"=0}, {"flags"=1, "Echo"=0, "Radial distance"=12.43, "Horizontal angle"=-0.7723081940074907, "Vertical angle"=0.00698131700797732, "Echo pulse width"=196, "Reserved"=70}, {"flags"=4, "Echo"=1, "Radial distance"=16.14, "Horizontal angle"=-0.7723081940074907, "Vertical angle"=0.00698131700797732, "Echo pulse width"=100, "Reserved"=0}, {"flags"=0, "Echo"=0, "Radial distance"=12.25, "Horizontal angle"=-0.7723081940074907, "Vertical angle"=0.020943951023931963, "Echo pulse width"=188, "Reserved"=70}, {"flags"=4, "Echo"=0, "Radial distance"=8.870000000000001, "Horizontal angle"=-0.7766715171374766, "Vertical angle"=-0.020943951023931952, "Echo pulse width"=276, "Reserved"=0}, {"flags"=4, "Echo"=0, "Radial distance"=11.790000000000001, "Horizontal angle"=-0.7766715171374766, "Vertical angle"=-0.006981317007977317, "Echo pulse width"=256, "Reserved"=0}, {"flags"=0, "Echo"=0, "Radial distance"=12.33, "Horizontal angle"=-0.7810348402674625, "Vertical angle"=0.00698131700797732, "Echo pulse width"=168, "Reserved"=70}, {"flags"=0, "Echo"=0, "Radial distance"=12.15, "Horizontal angle"=-0.7810348402674625, "Vertical angle"=0.020943951023931963, "Echo pulse width"=164, "Reserved"=70}, {"flags"=4, "Echo"=0, "Radial distance"=8.59, "Horizontal angle"=-0.7853981633974483, "Vertical angle"=-0.020943951023931952, "Echo pulse width"=332, "Reserved"=0}, {"flags"=4, "Echo"=0, "Radial distance"=11.32, "Horizontal angle"=-0.7853981633974483, "Vertical angle"=-0.006981317007977317, "Echo pulse width"=304, "Reserved"=0}, {"flags"=0, "Echo"=0, "Radial distance"=12.27, "Horizontal angle"=-0.789761486527434, "Vertical angle"=0.00698131700797732, "Echo pulse width"=192, "Reserved"=70}, {"flags"=0, "Echo"=0, "Radial distance"=12.08, "Horizontal angle"=-0.789761486527434, "Vertical angle"=0.020943951023931963, "Echo pulse width"=192, "Reserved"=70}, {"flags"=4, "Echo"=0, "Radial distance"=8.67, "Horizontal angle"=-0.7941248096574199, "Vertical angle"=-0.020943951023931952, "Echo pulse width"=276, "Reserved"=0}, {"flags"=4, "Echo"=0, "Radial distance"=11.5, "Horizontal angle"=-0.7941248096574199, "Vertical angle"=-0.006981317007977317, "Echo pulse width"=248, "Reserved"=0}, {"flags"=0, "Echo"=0, "Radial distance"=12.15, "Horizontal angle"=-0.7984881327874057, "Vertical angle"=0.00698131700797732, "Echo pulse width"=164, "Reserved"=70}, {"flags"=0, "Echo"=0, "Radial distance"=11.99, "Horizontal angle"=-0.7984881327874057, "Vertical angle"=0.020943951023931963, "Echo pulse width"=168, "Reserved"=70}, {"flags"=4, "Echo"=0, "Radial distance"=8.47, "Horizontal angle"=-0.8028514559173915, "Vertical angle"=-0.020943951023931952, "Echo pulse width"=324, "Reserved"=0}, {"flags"=4, "Echo"=0, "Radial distance"=11.16, "Horizontal angle"=-0.8028514559173915, "Vertical angle"=-0.006981317007977317, "Echo pulse width"=284, "Reserved"=0}, {"flags"=0, "Echo"=0, "Radial distance"=12.11, "Horizontal angle"=-0.8072147790473774, "Vertical angle"=0.00698131700797732, "Echo pulse width"=192, "Reserved"=70}, {"flags"=0, "Echo"=0, "Radial distance"=11.89, "Horizontal angle"=-0.8072147790473774, "Vertical angle"=0.020943951023931963, "Echo pulse width"=188, "Reserved"=70}, {"flags"=4, "Echo"=0, "Radial distance"=8.63, "Horizontal angle"=-0.8115781021773633, "Vertical angle"=-0.020943951023931952, "Echo pulse width"=276, "Reserved"=0}, {"flags"=4, "Echo"=0, "Radial distance"=11.33, "Horizontal angle"=-0.8115781021773633, "Vertical angle"=-0.006981317007977317, "Echo pulse width"=236, "Reserved"=0}, {"flags"=0, "Echo"=0, "Radial distance"=12.07, "Horizontal angle"=-0.8159414253073491, "Vertical angle"=0.00698131700797732, "Echo pulse width"=164, "Reserved"=70}, {"flags"=0, "Echo"=0, "Radial distance"=11.870000000000001, "Horizontal angle"=-0.8159414253073491, "Vertical angle"=0.020943951023931963, "Echo pulse width"=160, "Reserved"=70}, {"flags"=4, "Echo"=0, "Radial distance"=8.47, "Horizontal angle"=-0.8203047484373349, "Vertical angle"=-0.020943951023931952, "Echo pulse width"=312, "Reserved"=0}, {"flags"=4, "Echo"=0, "Radial distance"=11.120000000000001, "Horizontal angle"=-0.8203047484373349, "Vertical angle"=-0.006981317007977317, "Echo pulse width"=264, "Reserved"=0}, {"flags"=0, "Echo"=0, "Radial distance"=11.96, "Horizontal angle"=-0.8246680715673207, "Vertical angle"=0.00698131700797732, "Echo pulse width"=184, "Reserved"=70}, {"flags"=0, "Echo"=0, "Radial distance"=11.92, "Horizontal angle"=-0.8246680715673207, "Vertical angle"=0.020943951023931963, "Echo pulse width"=200, "Reserved"=70}, {"flags"=4, "Echo"=0, "Radial distance"=8.59, "Horizontal angle"=-0.8290313946973066, "Vertical angle"=-0.020943951023931952, "Echo pulse width"=264, "Reserved"=0}, {"flags"=4, "Echo"=0, "Radial distance"=11.33, "Horizontal angle"=-0.8290313946973066, "Vertical angle"=-0.006981317007977317, "Echo pulse width"=220, "Reserved"=0}, {"flags"=0, "Echo"=0, "Radial distance"=12.030000000000001, "Horizontal angle"=-0.8333947178272924, "Vertical angle"=0.00698131700797732, "Echo pulse width"=164, "Reserved"=70}, {"flags"=0, "Echo"=0, "Radial distance"=11.870000000000001, "Horizontal angle"=-0.8333947178272924, "Vertical angle"=0.020943951023931963, "Echo pulse width"=160, "Reserved"=70}, {"flags"=4, "Echo"=0, "Radial distance"=8.43, "Horizontal angle"=-0.8377580409572781, "Vertical angle"=-0.020943951023931952, "Echo pulse width"=304, "Reserved"=0}, {"flags"=4, "Echo"=0, "Radial distance"=11.0, "Horizontal angle"=-0.8377580409572781, "Vertical angle"=-0.006981317007977317, "Echo pulse width"=256, "Reserved"=0}, {"flags"=0, "Echo"=0, "Radial distance"=12.040000000000001, "Horizontal angle"=-0.842121364087264, "Vertical angle"=0.00698131700797732, "Echo pulse width"=184, "Reserved"=70}, {"flags"=0, "Echo"=0, "Radial distance"=11.89, "Horizontal angle"=-0.842121364087264, "Vertical angle"=0.020943951023931963, "Echo pulse width"=188, "Reserved"=70}, {"flags"=4, "Echo"=0, "Radial distance"=8.51, "Horizontal angle"=-0.8464846872172498, "Vertical angle"=-0.020943951023931952, "Echo pulse width"=256, "Reserved"=0}, {"flags"=4, "Echo"=0, "Radial distance"=11.24, "Horizontal angle"=-0.8464846872172498, "Vertical angle"=-0.006981317007977317, "Echo pulse width"=212, "Reserved"=0}, {"flags"=0, "Echo"=0, "Radial distance"=12.09, "Horizontal angle"=-0.8508480103472356, "Vertical angle"=0.00698131700797732, "Echo pulse width"=168, "Reserved"=70}, {"flags"=0, "Echo"=0, "Radial distance"=11.91, "Horizontal angle"=-0.8508480103472356, "Vertical angle"=0.020943951023931963, "Echo pulse width"=164, "Reserved"=70}, {"flags"=4, "Echo"=0, "Radial distance"=8.31, "Horizontal angle"=-0.8552113334772213, "Vertical angle"=-0.020943951023931952, "Echo pulse width"=308, "Reserved"=0}, {"flags"=4, "Echo"=0, "Radial distance"=10.84, "Horizontal angle"=-0.8552113334772213, "Vertical angle"=-0.006981317007977317, "Echo pulse width"=264, "Reserved"=0}, {"flags"=0, "Echo"=0, "Radial distance"=12.14, "Horizontal angle"=-0.8595746566072073, "Vertical angle"=0.00698131700797732, "Echo pulse width"=200, "Reserved"=70}, {"flags"=0, "Echo"=0, "Radial distance"=11.97, "Horizontal angle"=-0.8595746566072073, "Vertical angle"=0.020943951023931963, "Echo pulse width"=184, "Reserved"=70}, {"flags"=4, "Echo"=0, "Radial distance"=8.51, "Horizontal angle"=-0.8639379797371932, "Vertical angle"=-0.020943951023931952, "Echo pulse width"=240, "Reserved"=0}, {"flags"=4, "Echo"=0, "Radial distance"=11.34, "Horizontal angle"=-0.8639379797371932, "Vertical angle"=-0.006981317007977317, "Echo pulse width"=176, "Reserved"=0}, {"flags"=0, "Echo"=0, "Radial distance"=12.290000000000001, "Horizontal angle"=-0.868301302867179, "Vertical angle"=0.00698131700797732, "Echo pulse width"=176, "Reserved"=70}, {"flags"=0, "Echo"=0, "Radial distance"=12.19, "Horizontal angle"=-0.868301302867179, "Vertical angle"=0.020943951023931963, "Echo pulse width"=160, "Reserved"=70}]} {"hash" format="%016x"}
  out "header":T8
  out "Ibeo error out":errorcluster
types:
  T1 = cluster{"hash":i64, "sys time":i64, "type":u8, "raw":string}
  T2 = enum16{"Velodyne 16", "Velodyne 32", "Velodyne 64"}
  T3 = cluster{"hash":i64, "sys time":i64, "ref_vel":dbl, "ref_steer":dbl, "alert":u8}
  T4 = cluster{"hash":i64, "sys time":i64, "lat":dbl, "lon":dbl}
  T5 = cluster{"hash":i64, "sys time":i64, "n":u32, "pathxy":dbl[]}
  T6 = cluster{"hash":i64, "sys time":i64, "u time":i64, "alt":dbl}
  T7 = cluster{"hash":i64, "sys time":i64, "Header":cluster{"Size of prev messages":u32, "Size of this messages":u32, "Reserved":u8, "DeviceID":u8, "Data type":u16, "NTP time":u64}, "Scan header":cluster{"Scan number":u16, "scanner status":u16, "Sync phase offset":u16, "Scan start time NTP":u64, "Scan end time NTP":u64, "Angle ticks per rotation":u16, "Start angle":dbl, "End angle":dbl, "Scan points":u16, "pos_x":dbl, "pos_y":dbl, "pos_h":dbl, "Mounting position x":dbl, "Mounting position y":dbl, "Mounting position z":dbl, "Reserved":u16}, "Scan points":cluster{"flags":u8, "Echo":u8, "Radial distance":dbl, "Horizontal angle":dbl, "Vertical angle":dbl, "Echo pulse width":u16, "Reserved":u16}[]}
  T8 = cluster{"Size of prev messages":u32, "Size of this messages":u32, "Reserved":u8, "DeviceID":u8, "Data type":u16, "NTP time":u64}
  T9 = cluster{"hash":i64, "sys time":i64, "time":dbl, "yaw_rate":dbl, "mdps torque":dbl, "mdps str_ang":dbl, "VS_CAN":dbl, "lat_accel":dbl, "mcp":dbl, "accel pedal value":dbl, "tps":dbl, "odometer":dbl, "battery voltage":dbl}
  T10 = cluster{"identifier":u32, "timestamp":timestamp, "payload":u8[]}
  T11 = cluster{"hash":i64, "sys time":i64, "Timestamp":u32, "Rot_ang":dbl[], "Ver_ang":dbl[], "Dist":dbl[], "Ver_off":dbl[], "Intensity":u8[], "pos x":dbl, "pos y":dbl, "Heading":dbl}
  T12 = enum16{"big-endian, network order", "native, host order", "little-endian"}
  T13 = cluster{"Laser block ID":u16, "Rotational position":u16}
  T14 = cluster{"hash":i64, "sys time":i64, "n":i32, "error":i32[]}
  T15 = cluster{"hash":i64, "sys time":i64, "status":i32, "TS_num":i32}
  T16 = cluster{"Magic word":u32, "Size of prev messages":u32, "Size of this messages":u32, "Reserved":u8, "DeviceID":u8, "Data type":u16, "NTP time":u64}
  T17 = cluster{"command id":u16, "Reserved":u16, "parameter idx":u16}
  T18 = enum16{"Standard", "Buffered", "CRLF", "Immediate"}
  T19 = cluster{"connection ID":refnum<k16>, "net address":u32, "port":u16}
  T20 = cluster{"hash":i64, "sys time":i64, "time":dbl, "yaw_rate":dbl, "mdps torque":dbl, "mdps str_ang":dbl, "VS_CAN":dbl, "lat_accel":dbl, "mcp":dbl, "accel pedal value":dbl, "tps":dbl, "odometer":dbl, "battery voltage":dbl, "WHL_SPD_RR":dbl, "WHL_SPD_RL":dbl, "WHL_SPD_FR":dbl, "WHL_SPD_FL":dbl}
  T21 = cluster{"hash":i64, "sys time":i64, "size":i32, "data":u8[]}
  T22 = cluster{"hash":i64, "sys time":i64, "Auto":bool, "Run":bool, "Solenoid":bool, "T lim":bool, "brk_enc":u8, "B PWM":u16, "T PWM":u16, "ref_vel":dbl, "ref_bkr_enc":dbl, "ref_apv":dbl, "ref_steer":dbl, "net address":u32}
  T23 = cluster{"hash":i64, "sys time":i64, "Auto":bool, "Run":bool, "Solenoid":bool, "T lim":bool, "brk_enc":u8, "B PWM":u16, "T PWM":u16, "ref_vel":dbl, "ref_bkr_enc":dbl, "ref_apv":dbl, "ref_steer":dbl}
  T24 = cluster{"hash":i64, "sys time":i64, "mobileye":u8[]}
  T25 = cluster{"hash":i64, "sys time":i64, "mobileye time":u32, "ID":u32, "data":u8[]}
  T26 = cluster{"hash":i64, "sys time":i64, "car time":u32, "ID":u32, "data":u8[]}
  T27 = cluster{"Scan number":u16, "scanner status":u16, "Sync phase offset":u16, "Scan start time NTP":u64, "Scan end time NTP":u64, "Angle ticks per rotation":u16, "Start angle":dbl, "End angle":dbl, "Scan points":u16, "pos_x":dbl, "pos_y":dbl, "pos_h":dbl, "Mounting position x":dbl, "Mounting position y":dbl, "Mounting position z":dbl, "Reserved":u16}
  T28 = cluster{"flags":u8, "Echo":u8, "Radial distance":dbl, "Horizontal angle":dbl, "Vertical angle":dbl, "Echo pulse width":u16, "Reserved":u16}[]
  T29 = cluster{"hash":i64, "sys time":i64, "Header":cluster{"Size of prev messages":u32, "Size of this messages":u32, "Reserved":u8, "DeviceID":u8, "Data type":u16, "NTP time":u64}, "Scan header":cluster{"Scan number":u16, "scanner status":u16, "Sync phase offset":u16, "Scan start time NTP":u64, "Scan end time NTP":u64, "Angle ticks per rotation":u16, "Start angle":dbl, "End angle":dbl, "Scan points":u16, "pos_x":dbl, "pos_y":dbl, "pos_h":dbl, "Mounting position x":dbl, "Mounting position y":dbl, "Mounting position z":dbl, "Reserved":u16}}
  T30 = cluster{"flags":u8, "Echo":u8, "Radial distance":dbl, "Horizontal angle":dbl, "Vertical angle":dbl, "Echo pulse width":u16, "Reserved":u16}
  T31 = cluster{"hash":i64, "sys time":i64, "Timestamp":u32, "Rotational angle":u16[], "dist":u16[][], "Intensity":u8[][], "pos_x":dbl, "pos_y":dbl, "pos_h":dbl}
  T32 = cluster{"hash":i64, "sys time":i64, "dt":dbl, "x":dbl, "y":dbl, "speed":dbl, "heading":dbl, "yaw_rate":dbl}
  T33 = cluster{"X":dbl[], "Y":dbl[], "Z":dbl[], "d":dbl[], "i":u8[]}
  T34 = cluster{"hash":i64, "sys time":i64, "n":i32, "data1":dbl[], "data2":dbl[], "lat":dbl[], "lon":dbl[]}
  T35 = cluster{"beep":bool, "duration (msec)":u32, "frequency (Hz)":u32}
  T36 = cluster{"hash":i64, "sys time":i64, "time":dbl, "x":dbl, "y":dbl, "h":dbl, "numSV":i32, "postype":i32, "lag":i32, "hordev":dbl, "lat":dbl, "lon":dbl, "hgt":dbl, "map_idx":i32}
  T37 = cluster{"hash":i64, "sys time":i64, "s_lat":dbl, "s_lon":dbl, "d_lat":dbl, "d_lon":dbl, "Message":i64}
  T38 = cluster{"hash":i64, "sys time":i64, "status":i32, "TS_num":i32, "TS_type":i32[], "TS_loc_x":dbl[], "TS_loc_y":dbl[]}
  T39 = cluster{"hash":i64, "sys time":i64, "left_lane_exist":bool, "right_lane_exist":bool, "left_lane_dot":dbl, "right_lane_dot":dbl}
  T40 = cluster{"hash":i64, "sys time":i64, "stopline_exist":bool, "stopline_distance":dbl}
  T41 = cluster{"hash":i64, "sys time":i64, "time":dbl, "speed":dbl, "heading":dbl, "lat":dbl, "lon":dbl}
  T42 = cluster{"Scan number":u16, "scanner status":u16, "Sync phase offset":u16, "Scan start time NTP":u64, "Scan end time NTP":u64, "Angle ticks per rotation":u16, "Start angle":i16, "End angle":i16, "Scan points":u16, "Mounting position yaw angle ":i16, "Mounting position pitch angle":i16, "Mounting position roll angle":i16, "Mounting position x":i16, "Mounting position y":i16, "Mounting position z":i16, "Reserved":u16}
  T43 = cluster{"Scan number":u16, "scanner status":u16, "Sync phase offset":u16, "Scan start time NTP":u64, "Scan end time NTP":u64, "Angle ticks per rotation":u16, "Start angle":dbl, "End angle":dbl, "Scan points":u16, "Mounting position yaw angle ":dbl, "Mounting position pitch angle":dbl, "Mounting position roll angle":dbl, "Mounting position x":dbl, "Mounting position y":dbl, "Mounting position z":dbl, "Reserved":u16}
  T44 = cluster{"Layer/Echo":u8, "flags":u8, "Horizontal angle":i16, "Radial distance":u16, "Echo pulse width":u16, "Reserved":u16}
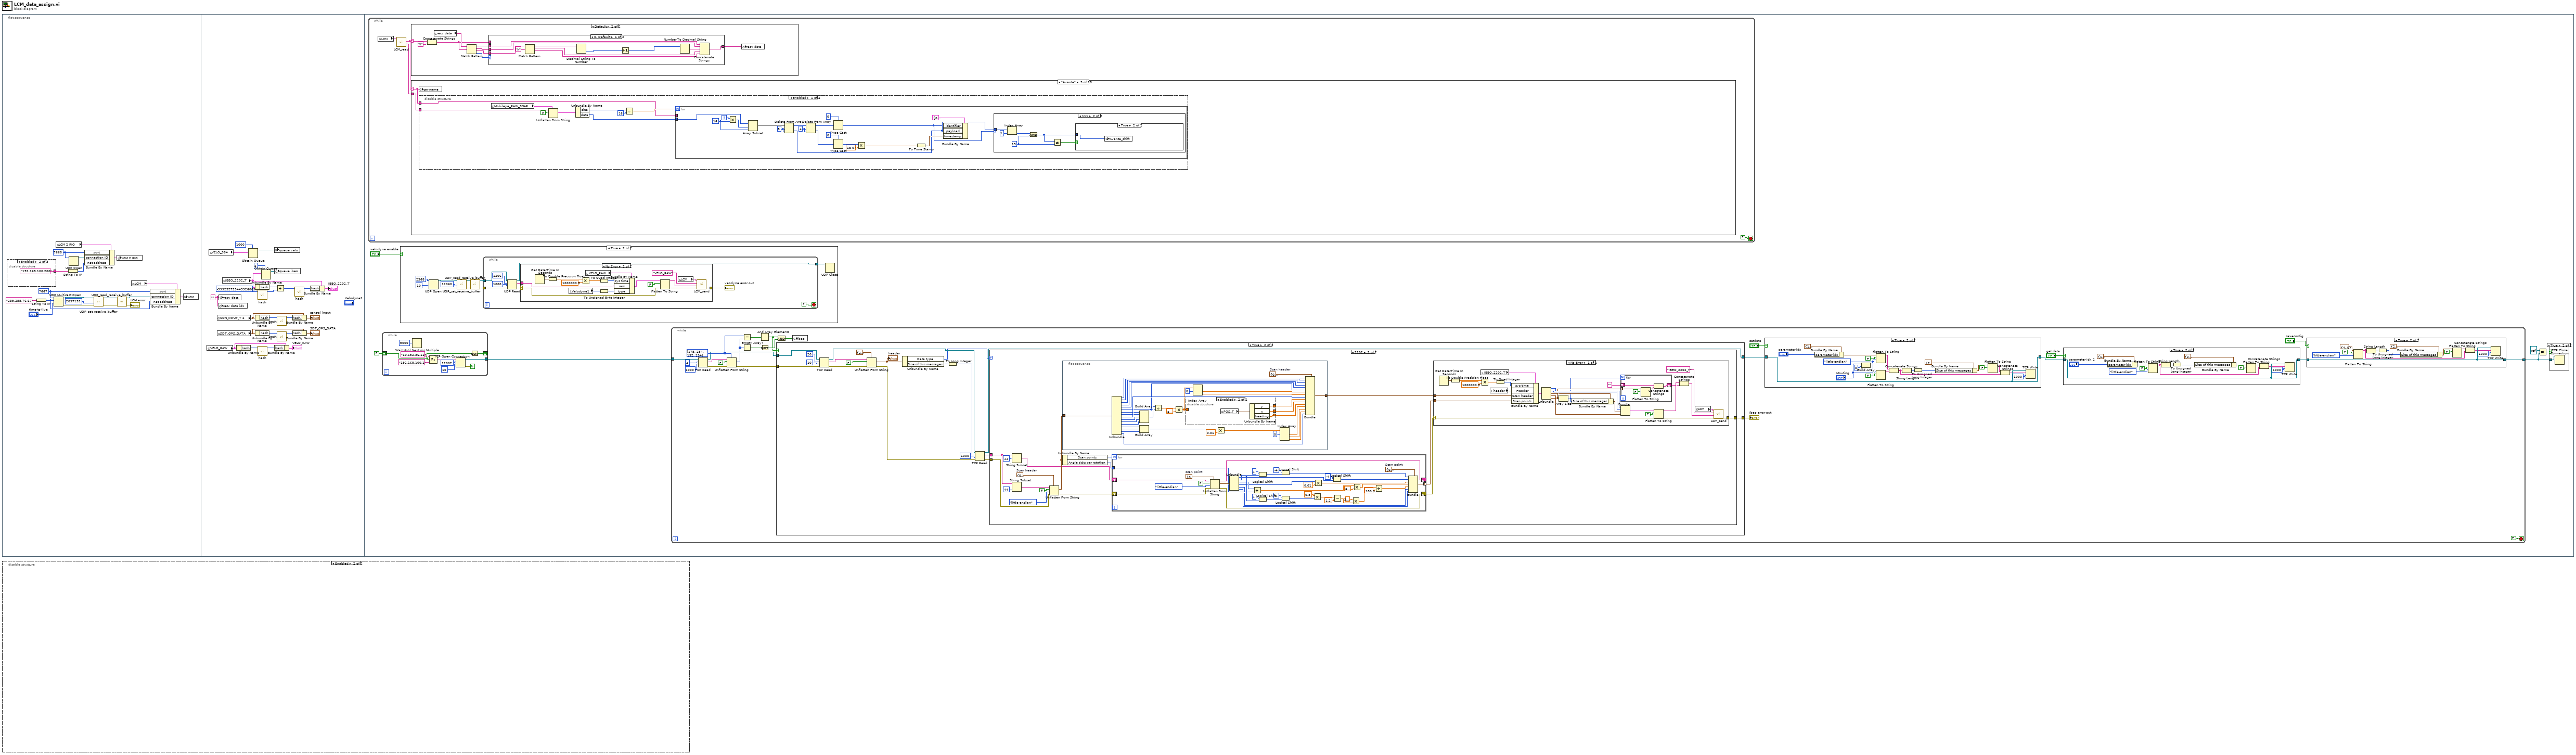
[diagram p0: block diagram]
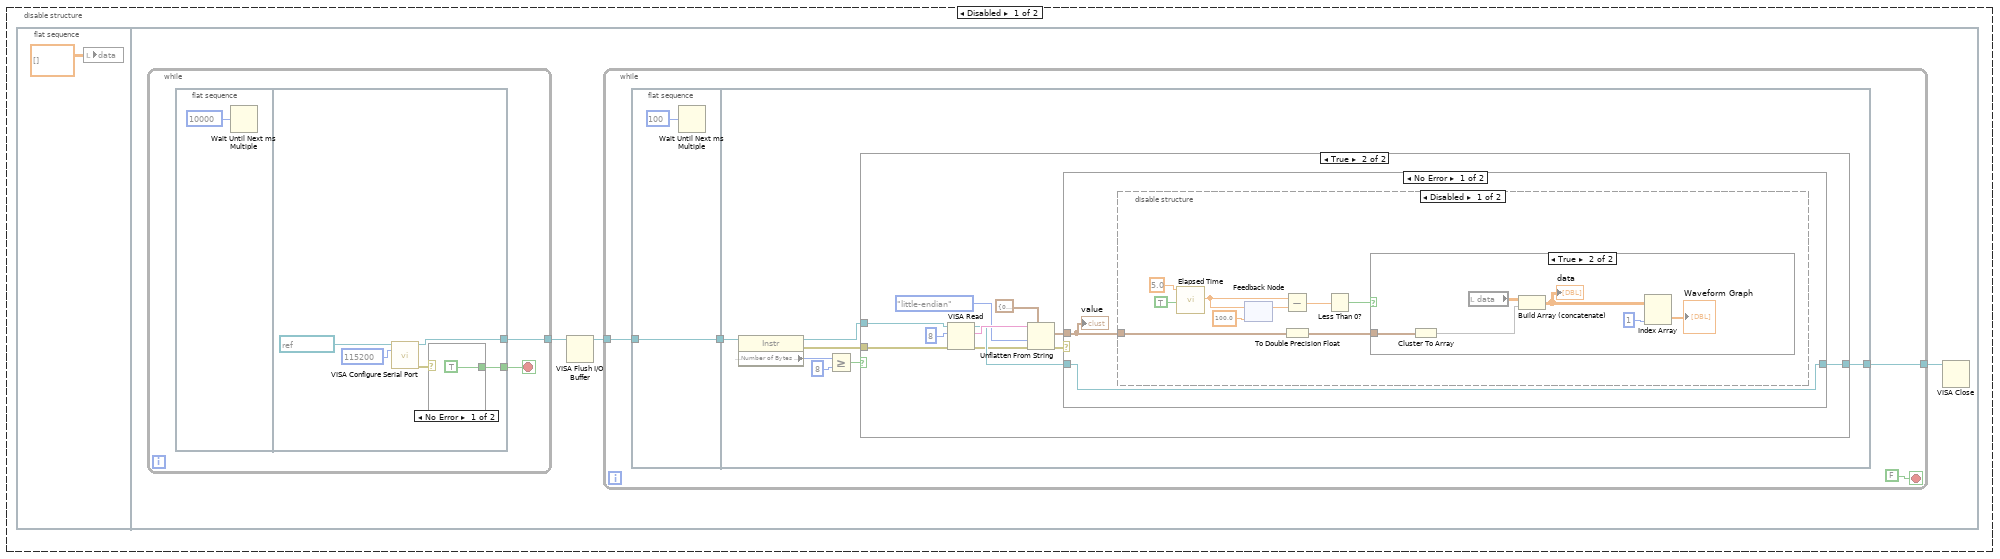
[diagram p2: hidden frame]
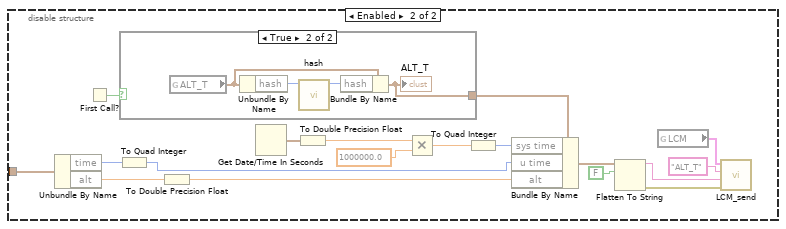
[diagram p6: hidden frame]
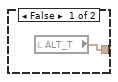
[diagram p7: hidden frame]
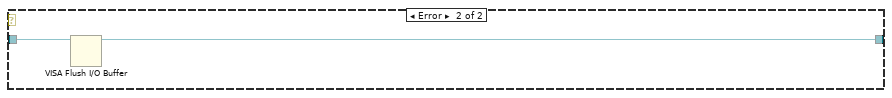
[diagram p8: hidden frame]
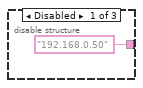
[diagram p9: hidden frame]
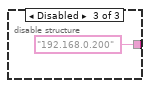
[diagram p10: hidden frame]
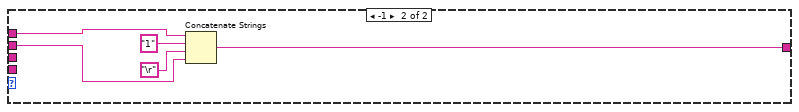
[diagram p12: hidden frame]
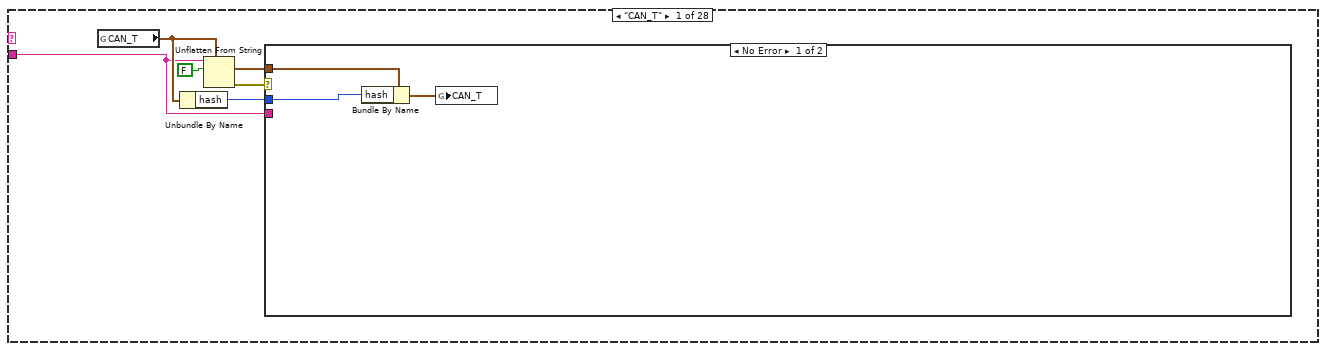
[diagram p13: hidden frame]
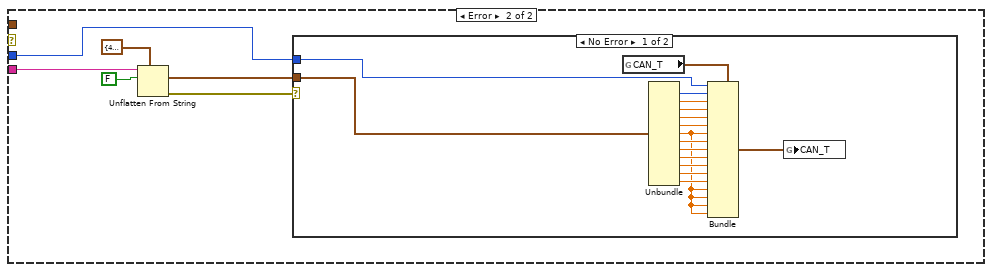
[diagram p14: hidden frame]
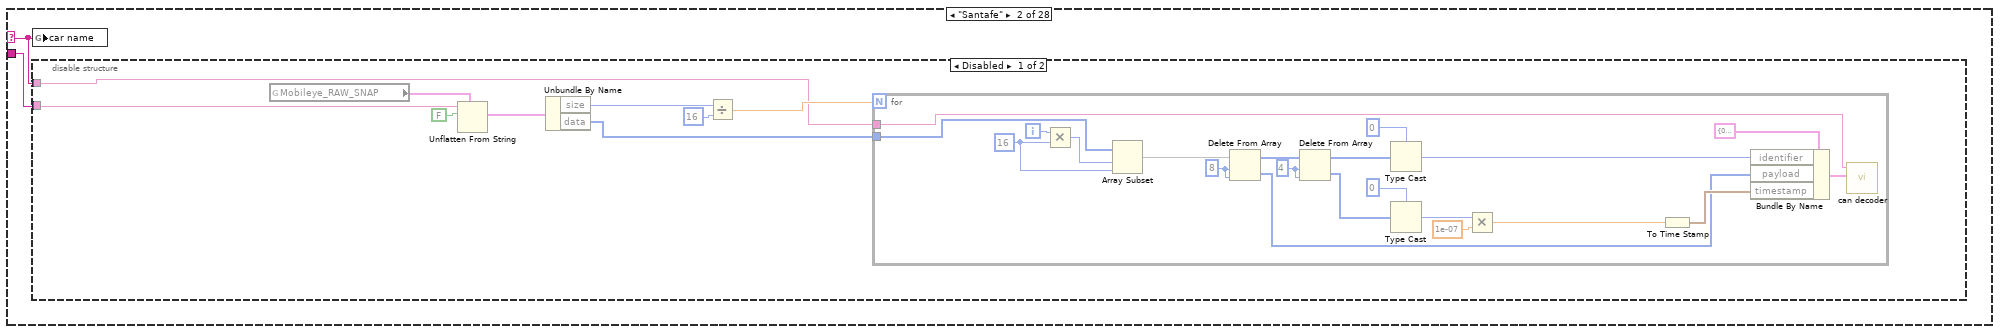
[diagram p16: hidden frame]
diagram:
  n1 = flat-sequence {
    frame #0 {
      w8 = u16 7667 ("port")
      w17 = u16 7668 ("port 2")
      n2 = disable-structure shown="Enabled" {
        disable-tunnel: ["192.168.0.50" ("name") "192.168.100.200" ("name") "192.168.0.200" ("name")] -> w14
        frame Disabled {
        }
        frame Enabled {
        }
        frame Disabled {
        }
      }
      n3 = String To IP(1:"239.255.76.67" ("Multicast Address")) -> (0:w9:u32)
      n4 = UDP Multicast Open(9:"time-to-live", 10:w9, 11:w8) -> (0:w2:errorcluster, 3:w4:refnum<k16>)  [unwired: 2 in, 1 out]
      n5 = global read "G_LCM.vi" "LCM 2 RIO"() -> (w19:T19)
      n6 = String To IP(1:w14) -> (0:w15:u32)
      n7 = UDP Open(11:w17) -> (port=w16:refnum<k16>)  [unwired: 4 in, 2 out]
      n8 = Bundle By Name(cluster=w19, "port"=w17, "connection ID"=w16, "net address"=w15) -> (w18:T19)
      n9 = call "UDP_set_receive_buffer.vi"("error in (no error)"=w2, "Receive Buffer Size"=u32 2097152, "connection ID"=w4) -> ("error out"=w6:errorcluster, "connection ID out"=w5:refnum<k16>)  [unwired: 6 in]
      n10 = global write "G_LCM.vi" "LCM 2 RIO"(w18) -> ()
      n11 = call "UDP_read_receive_buffer.vi"("error in (no error)"=w6, "connection ID"=w5) -> ("error out"=→"LCM error":errorcluster, "connection ID out"=w3:refnum<k16>)  [unwired: 5 in, 1 out]
      n12 = global read "G_LCM.vi" "LCM"() -> (w11:T19)
      n13 = Bundle By Name(cluster=w11, "port"=w8, "connection ID"=w3, "net address"=w9) -> (w10:T19)
      n14 = global write "G_LCM.vi" "LCM"(w10) -> ()
    }
    frame #1 {
      w34 = "" ("recv data idx")
      n15 = global read "G_LCM.vi" "VELO_RAW"() -> (w26:T1)
      n16 = global read "G_LCM.vi" "VELO_384"() -> (w24:T11)
      n17 = global read "G_LCM.vi" "CON_INPUT_T 2"() -> (w36:T3)
      n18 = global read "G_LCM.vi" "SDT_GPS_DATA"() -> (w40:T4)
      n19 = global write "G_LCM.vi" "recv data idx"(w34) -> ()
      n20 = global write "G_LCM.vi" "recv data"(w34) -> ()
      n21 = global read "G_LCM.vi" "IBEO_2202_T"() -> (w31:T7)
      n22 = Unbundle By Name(w26) -> ("hash"=w29:i64)
      n23 = Obtain Queue(max queue size (-1, unlimited)=1000, element data type=w24) -> (queue out=w25:refnum<queue>)  [unwired: 3 in, 2 out]
      n24 = Unbundle By Name(w31) -> ("hash"=w43:i64)
      n25 = Unbundle By Name(w36) -> ("hash"=w37:i64)
      n26 = Unbundle By Name(w40) -> ("hash"=w41:i64)
      n27 = call "hash.vi"("input"=i64 -3992327254439260095 ("hash")) -> ("output"=w42:i64)  [unwired: 10 in]
      n28 = call "hash.vi"("input"=w29) -> ("output"=w28:i64)  [unwired: 10 in]
      n29 = Obtain Queue(max queue size (-1, unlimited)=2, element data type=w31) -> (queue out=w30:refnum<queue>)  [unwired: 3 in, 2 out]
      n30 = global write "G_LCM.vi" "queue velo"(w25) -> ()
      n31 = global write "G_LCM.vi" "queue ibeo"(w30) -> ()
      n32 = Bundle By Name(cluster=w26, "hash"=w28) -> (→"VELO_RAW":T1)
      n33 = Add(x=w43, y=w42) -> (x+y=w44:i64)
      n34 = call "hash.vi"("input"=w37) -> ("output"=w35:i64)  [unwired: 10 in]
      n35 = call "hash.vi"("input"=w41) -> ("output"=w39:i64)  [unwired: 10 in]
      n36 = Bundle By Name(cluster=w36, "hash"=w35) -> (→"control input":T3)
      n37 = Bundle By Name(cluster=w40, "hash"=w39) -> (→"SDT_GPS_DATA":T4)
      n38 = call "hash.vi"("input"=w44) -> ("output"=w47:i64)  [unwired: 10 in]
      n39 = Bundle By Name(cluster=w31, "hash"=w47) -> (→"IBEO_2202_T":T7)
    }
    frame #2 {
      n40 = while {
        stop <- FALSE stop-if-true
        n41 = global read "G_LCM.vi" "LCM"() -> (w54:T19)
        n42 = call "LCM_read.vi"("LCM"=w54) -> ("data"=w57:string, "ID"=w56:string)  [unwired: 7 in, 2 out]
        n43 = case shown="Default" w56 {
          selector: w56 -> [_ w58]
          frame "" {
          }
          frame Default {
            n44 = Concatenate Strings(w58, "\t") -> (w59:string)
            n45 = global read "G_LCM.vi" "recv data"() -> (w64:string)
            n46 = Match Pattern(string=w64, regular expression=w59) -> (before substring=w63:string, match substring=w62:string, after substring=w61:string, offset past match=w66:i32)  [unwired: 1 in]
            n47 = case shown="0, Default" w66 {
              tunnel: w63 -> [w70 w78]
              tunnel: w62 -> [w69 _]
              tunnel: w61 -> [w68 _]
              tunnel: [w67 w80] -> w60
              tunnel: w59 -> [_ w79]
              frame 0, Default {
                n48 = Match Pattern(string=w68, regular expression="\r") -> (before substring=w77:string, match substring=w73:string, after substring=w74:string)  [unwired: 1 in, 1 out]
                n49 = Decimal String To Number(string=w77) -> (number=w72:i32)  [unwired: 2 in, 1 out]
                n50 = Increment(x=w72) -> (x+1=w76:i32)
                n51 = Number To Decimal String(number=w76) -> (decimal integer string=w75:string)  [unwired: 1 in]
                n52 = Concatenate Strings(w70, w69, w75, w73, w74) -> (w67:string)
              }
              frame -1 {
                n53 = Concatenate Strings(w79, "1", "\r", w78) -> (w80:string)
              }
            }
            n54 = global write "G_LCM.vi" "recv data"(w60) -> ()
          }
        }
        n55 = case shown="\"Avante\"" w56 {
          selector: w56 -> [_ w114 w146 w183 w184 _ _ _ _ _ _ _ _ _ _ _ _ _ _ _ _ _ _ _ _ _ _ _]
          tunnel: w57 -> [w83 w115 w147 _ w185 w194 w286 w296 w309 _ w325 w352 w358 w367 w492 w501 w513 w533 w545 w566 w572 w595 w604 w613 w636 w645 w658 w667]
          frame "CAN_T" {
            n56 = global read "G_LCM.vi" "CAN_T"() -> (w87:T20)
            n57 = Unbundle By Name(w87) -> ("hash"=w85:i64)
            n58 = Unflatten From String(type=w87, binary string=w83, data includes array or string size? (T)=FALSE) -> (value=w86:T20, error out=w84:errorcluster)  [unwired: 2 in, 1 out]
            n59 = case shown="No Error" w84 {
              tunnel: w86 -> [w91 _]
              tunnel: w85 -> [w90 w93]
              tunnel: w83 -> [_ w97]
              frame No Error {
                n60 = Bundle By Name(cluster=w91, "hash"=w90) -> (w89:T20)
                n61 = global write "G_LCM.vi" "CAN_T"(w89) -> ()
              }
              frame Error {
                n62 = Unflatten From String(type=T9 {"hash"=4925705798588944810, "sys time"=0, "time"=0.0, "yaw_rate"=0.0, "mdps torque"=0.0, "mdps str_ang"=0.0, "VS_CAN"=0.0, "lat_accel"=0.0, "mcp"=0.0, "accel pedal value"=0.0, "tps"=0.0, "odometer"=0.0, "battery voltage"=0.0} ("CAN_T"), binary string=w97, data includes array or string size? (T)=FALSE) -> (value=w94:T9, error out=w92:errorcluster)  [unwired: 2 in, 1 out]
                n63 = case shown="No Error" w92 {
                  tunnel: w94 -> [w113 _]
                  tunnel: w93 -> [w99 _]
                  frame No Error {
                    n64 = global read "G_LCM.vi" "CAN_T"() -> (w112:T20)
                    n65 = Unbundle(w113) -> ("sys time"=w111:i64, "time"=w110:dbl, "yaw_rate"=w109:dbl, "mdps torque"=w108:dbl, "mdps str_ang"=w107:dbl, "VS_CAN"=w100:dbl, "lat_accel"=w106:dbl, "mcp"=w105:dbl, "accel pedal value"=w104:dbl, "tps"=w103:dbl, "odometer"=w102:dbl, "battery voltage"=w101:dbl)  [unwired: 1 out]
                    n66 = Bundle(cluster=w112, "hash"=w99, "sys time"=w111, "time"=w110, "yaw_rate"=w109, "mdps torque"=w108, "mdps str_ang"=w107, "VS_CAN"=w100, "lat_accel"=w106, "mcp"=w105, "accel pedal value"=w104, "tps"=w103, "odometer"=w102, "battery voltage"=w101, "WHL_SPD_RR"=w100, "WHL_SPD_RL"=w100, "WHL_SPD_FR"=w100, "WHL_SPD_FL"=w100) -> (w98:T20)
                    n67 = global write "G_LCM.vi" "CAN_T"(w98) -> ()
                  }
                  frame Error {
                  }
                }
              }
            }
          }
          frame "Santafe" {
            n68 = global write "G_LCM.vi" "car name"(w114) -> ()
            n69 = disable-structure shown="Disabled" {
              disable-tunnel: w115 -> [w118 _]
              disable-tunnel: w114 -> [w116 _]
              frame Disabled {
                n70 = global read "G_LCM.vi" "Mobileye_RAW_SNAP"() -> (w119:T21)
                n71 = Unflatten From String(type=w119, binary string=w118, data includes array or string size? (T)=FALSE) -> (value=w117:T21)  [unwired: 2 in, 2 out]
                n72 = Unbundle By Name(w117) -> ("size"=w121:i32, "data"=w124:u8[])
                n73 = Divide(x=w121, y=16) -> (x/y=w123:dbl)
                n74 = for {
                  N: w123 -> [_]
                  tunnel: w124 -> [w145]
                  tunnel: w116 -> [w125]
                  i -> [w144]
                  w137 = 4 ("length")
                  w135 = 8 ("index")
                  w143 = 16 ("y")
                  n75 = Multiply(x=w144, y=w143) -> (x*y=w142:i32)
                  n76 = Array Subset(array=w145, index=w142, length=w143) -> (w127:u8[])
                  n77 = Delete From Array(array=w127, length=w135, index=w135) -> (deleted portion=w128:u8[], array with subset deleted=w136:u8[])
                  n78 = Delete From Array(array=w136, length=w137, index=w137) -> (deleted portion=w141:u8[], array with subset deleted=w138:u8[])
                  n79 = Type Cast(type=u32 0, x=w138) -> (*(type *) &x=w129:u32)
                  n80 = Type Cast(type=u32 0, x=w141) -> (*(type *) &x=w130:u32)
                  n81 = Multiply(x=w130, y=1e-07) -> (x*y=w133:dbl)
                  n82 = To Time Stamp(1:w133) -> (0:w132:timestamp)
                  n83 = Bundle By Name(cluster=T10 {"identifier"=0, "timestamp"=timestamp(0 s since 1904-01-01), "payload"=[]} ("can cluster"), "identifier"=w129, "payload"=w128, "timestamp"=w132) -> (w126:T10)
                  n84 = call "can decoder.vi"("can cluster"=w126, "name"=w125) -> ()  [unwired: 10 in]
                }
              }
              frame Enabled {
              }
            }
          }
          frame "Avante" {
            n85 = global write "G_LCM.vi" "car name"(w146) -> ()
            n86 = disable-structure shown="Enabled" {
              disable-tunnel: w147 -> [w150 _]
              disable-tunnel: w146 -> [w148 _]
              frame Enabled {
                n87 = global read "G_LCM.vi" "Mobileye_RAW_SNAP"() -> (w151:T21)
                n88 = Unflatten From String(type=w151, binary string=w150, data includes array or string size? (T)=FALSE) -> (value=w149:T21)  [unwired: 2 in, 2 out]
                n89 = Unbundle By Name(w149) -> ("size"=w153:i32, "data"=w156:u8[])
                n90 = Divide(x=w153, y=16) -> (x/y=w155:dbl)
                n91 = for {
                  N: w155 -> [_]
                  tunnel: w156 -> [w175]
                  tunnel: w148 -> [_]
                  i -> [w174]
                  w167 = 4 ("length")
                  w165 = 8 ("index")
                  w173 = 16 ("y")
                  n92 = Multiply(x=w174, y=w173) -> (x*y=w172:i32)
                  n93 = Array Subset(array=w175, index=w172, length=w173) -> (w159:u8[])
                  n94 = Delete From Array(array=w159, length=w165, index=w165) -> (deleted portion=w158:u8[], array with subset deleted=w166:u8[])
                  n95 = Delete From Array(array=w166, length=w167, index=w167) -> (deleted portion=w171:u8[], array with subset deleted=w168:u8[])
                  n96 = Type Cast(type=u32 0, x=w168) -> (*(type *) &x=w157:u32)
                  n97 = Type Cast(type=u32 0, x=w171) -> (*(type *) &x=w160:u32)
                  n98 = Multiply(x=w160, y=1e-07) -> (x*y=w163:dbl)
                  n99 = To Time Stamp(1:w163) -> (0:w162:timestamp)
                  n100 = Bundle By Name(cluster=T10 {"identifier"=0, "timestamp"=timestamp(0 s since 1904-01-01), "payload"=[]} ("can cluster"), "identifier"=w157, "payload"=w158, "timestamp"=w162) -> ()  [unwired: 1 out]
                  n101 = case shown="111" w157 {
                    tunnel: w158 -> [_ w176]
                    frame 0, Default {
                    }
                    frame 273 {
                      w179 = u8 15 ("y")
                      n102 = Index Array(array=w176, index=1) -> (element=w178:u8)
                      n103 = And(x=w178, y=w179) -> (x .and. y?=w180:u8)
                      n104 = Not Equal?(x=w180, y=w179) -> (x != y?=w181:bool)
                      n105 = case shown="True" w181 {
                        tunnel: w180 -> [_ w182]
                        frame False {
                        }
                        frame True {
                          n106 = global write "G_ALL.vi" "Avante_shift"(w182) -> ()
                        }
                      }
                    }
                  }
                }
              }
              frame Disabled {
              }
            }
          }
          frame "Prius" {
            # "s"
            n107 = global write "G_LCM.vi" "car name"(w183) -> ()
          }
          frame "Mobileye560", "Mobileye560S" {
            n108 = global write "G_LCM.vi" "Mobileye name"(w184) -> ()
            n109 = global read "G_LCM.vi" "Mobileye_RAW_SNAP"() -> (w189:T21)
            n110 = Unbundle By Name(w189) -> ("hash"=w187:i64)
            n111 = Unflatten From String(type=w189, binary string=w185, data includes array or string size? (T)=FALSE) -> (value=w188:T21, error out=w186:errorcluster)  [unwired: 2 in, 1 out]
            n112 = case shown="No Error" w186 {
              tunnel: w188 -> [w193 _]
              tunnel: w187 -> [w192 _]
              frame No Error {
                n113 = Bundle By Name(cluster=w193, "hash"=w192) -> (w191:T21)
                n114 = global write "G_LCM.vi" "Mobileye_RAW_SNAP"(w191) -> ()
              }
              frame Error {
              }
            }
          }
          frame "CON_T" {
            n115 = flat-sequence {
              tunnel: w194 -> [w195]
              frame #0 {
                n116 = global read "G_LCM.vi" "CON_T 2"() -> (w198:T22)
                n117 = Unflatten From String(type=w198, binary string=w195, data includes array or string size? (T)=FALSE) -> (value=w197:T22, error out=w196:errorcluster)  [unwired: 2 in, 1 out]
                n118 = case shown="No Error" w196 {
                  tunnel: w197 -> [w215 _]
                  tunnel: w195 -> [_ w231]
                  frame No Error {
                    n119 = Unbundle(w215) -> ("sys time"=w216:i64, "Auto"=w214:bool, "Run"=w213:bool, "Solenoid"=w212:bool, "T lim"=w211:bool, "brk_enc"=w210:u8, "B PWM"=w209:u16, "T PWM"=w208:u16, "ref_vel"=w207:dbl, "ref_bkr_enc"=w206:dbl, "ref_apv"=w205:dbl, "ref_steer"=w204:dbl, "net address"=w200:u32)  [unwired: 1 out]
                    n120 = global read "G_LCM.vi" "CON_T"() -> (w203:T23)
                    n121 = First Call?() -> (First Call?: T/F=w201:bool)
                    n122 = case shown="True" w201 {
                      tunnel: w200 -> [_ w219]
                      frame False {
                      }
                      frame True {
                        n123 = flat-sequence {
                          tunnel: w219 -> [w222]
                          tunnel: [w222] -> w218
                          tunnel: w218 -> [w223]
                          frame #0 {
                            n124 = global read "G_LCM.vi" "LCM 2 RIO"() -> (w221:T19)
                            n125 = Unbundle By Name(w221) -> ("connection ID"=w220:refnum<k16>)
                            n126 = UDP Close(connection ID=w220) -> ()  [unwired: 1 in, 2 out]
                          }
                          frame #1 {
                            w225 = u16 7668 ("port 2")
                            n127 = global read "G_LCM.vi" "LCM 2 RIO"() -> (w227:T19)
                            n128 = UDP Open(11:w225) -> (port=w224:refnum<k16>)  [unwired: 4 in, 2 out]
                            n129 = Bundle By Name(cluster=w227, "port"=w225, "connection ID"=w224, "net address"=w223) -> (w226:T19)
                            n130 = global write "G_LCM.vi" "LCM 2 RIO"(w226) -> ()
                          }
                        }
                      }
                    }
                    n131 = Unbundle By Name(w203) -> ("hash"=w202:i64)
                    n132 = Bundle(cluster=w203, "hash"=w202, "sys time"=w216, "Auto"=w214, "Run"=w213, "Solenoid"=w212, "T lim"=w211, "brk_enc"=w210, "B PWM"=w209, "T PWM"=w208, "ref_vel"=w207, "ref_bkr_enc"=w206, "ref_apv"=w205, "ref_steer"=w204) -> (w217:T23)
                    n133 = global write "G_LCM.vi" "CON_T"(w217) -> ()
                  }
                  frame Error {
                    n134 = global read "G_LCM.vi" "CON_T"() -> (w233:T23)
                    n135 = Unbundle By Name(w233) -> ("hash"=w228:i64)
                    n136 = Unflatten From String(type=w233, binary string=w231, data includes array or string size? (T)=FALSE) -> (value=w229:T23, error out=w230:errorcluster)  [unwired: 2 in, 1 out]
                    n137 = case shown="No Error" w230 {
                      tunnel: w229 -> [w236 _]
                      tunnel: w228 -> [w234 _]
                      frame No Error {
                        n138 = Bundle By Name(cluster=w236, "hash"=w234) -> (w235:T23)
                        n139 = global write "G_LCM.vi" "CON_T"(w235) -> ()
                      }
                      frame Error {
                      }
                    }
                  }
                }
              }
              frame #1 {
                n140 = disable-structure shown="Enabled" {
                  frame Enabled {
                    n141 = Get Date/Time In Seconds() -> (seconds since 1Jan1904=w257:timestamp)
                    n142 = global read "G_LCM.vi" "ibeo"() -> (w243:bool)
                    n143 = To Double Precision Float(number=w257) -> (double precision float=w256:dbl)
                    n144 = global read "G_ALL.vi" "Steering"() -> (w238:dbl)
                    n145 = Build Array(w243) -> (w242:bool[])
                    n146 = Multiply(x=w256, y=1000000.0) -> (x*y=w254:dbl)
                    n147 = Negate(x=w238) -> (-x=w237:dbl)
                    n148 = Boolean Array To Number(Boolean array=w242) -> (number=w241:u32)
                    n149 = local read "control input"() -> (w246:T3)
                    n150 = global read "G_ALL.vi" "VS_des"() -> (w239:dbl)
                    n151 = To Quad Integer(1:w254) -> (0:w253:i64)
                    n152 = To Unsigned Byte Integer(number=w241) -> (unsigned 8bit integer=w240:u8)
                    n153 = Add(x=w237, y=0.0) -> (x+y=w244:dbl)
                    n154 = Bundle By Name(cluster=w246, "sys time"=w253, "ref_vel"=w239, "ref_steer"=w244, "alert"=w240) -> (w248:T3)
                    n155 = global read "G_LCM.vi" "LCM 2 RIO"() -> (w247:T19)
                    n156 = Flatten To String(anything=w248, prepend array or string size? (T)=FALSE) -> (data string=w249:string, error out=w252:errorcluster)  [unwired: 2 in, 1 out]
                    n157 = call "LCM_send.vi"("error in (no error)"=w252, "DATA"=w249, "ID"="CON_INPUT_T", "LCM"=w247) -> ()  [unwired: 6 in, 2 out]
                  }
                  frame Disabled {
                  }
                }
              }
              frame #2 {
                n158 = global read "G_ALL.vi" "replay"() -> (w258:bool)
                n159 = case shown="False" w258 {
                  frame False {
                    n160 = disable-structure shown="Enabled" {
                      frame Enabled {
                        n161 = First Call?() -> (First Call?: T/F=w268:bool)
                        n162 = case shown="True" w268 {
                          tunnel: [w280 w281] -> w267
                          frame False {
                            n163 = local read "PATH_T"() -> (w280:T5)
                          }
                          frame True {
                            n164 = global read "G_LCM.vi" "PATH_T"() -> (w282:T5)
                            n165 = Unbundle By Name(w282) -> ("hash"=w284:i64)
                            n166 = call "hash.vi"("input"=w284) -> ("output"=w283:i64)  [unwired: 10 in]
                            n167 = Bundle By Name(cluster=w282, "hash"=w283) -> (w281:T5)
                            "PATH_T" <- w281
                          }
                        }
                        n168 = global read "G_ALL.vi" "map_track 2"() -> (w259:dbl[][])
                        n169 = Get Date/Time In Seconds() -> (seconds since 1Jan1904=w274:timestamp)
                        n170 = To Double Precision Float(number=w274) -> (double precision float=w275:dbl)
                        n171 = Transpose 2D Array(2D array=w259) -> (transposed array=w263:dbl[][])
                        n172 = Array Size(array=w259) -> (size(s)=w262:i32[])
                        n173 = Multiply(x=w275, y=1000000.0) -> (x*y=w277:dbl)
                        n174 = Multiply Array Elements(1:w262) -> (0:w261:i32)
                        n175 = Index Array(array=w262, index=0) -> (element=w265:i32)
                        n176 = Reshape Array(w263, w261) -> (w260:dbl[])
                        n177 = To Quad Integer(1:w277) -> (0:w273:i64)
                        n178 = To Unsigned Long Integer(number=w265) -> (unsigned 32bit integer=w264:u32)
                        n179 = Bundle By Name(cluster=w267, "sys time"=w273, "n"=w264, "pathxy"=w260) -> (w272:T5)
                        n180 = Flatten To String(anything=w272, prepend array or string size? (T)=FALSE) -> (data string=w270:string, error out=w269:errorcluster)  [unwired: 2 in, 1 out]
                        n181 = global read "G_LCM.vi" "LCM"() -> (w279:T19)
                        n182 = call "LCM_send.vi"("error in (no error)"=w269, "DATA"=w270, "ID"="PATH_T", "LCM"=w279) -> ()  [unwired: 6 in, 2 out]
                      }
                      frame Disabled {
                      }
                    }
                  }
                  frame True {
                  }
                }
              }
            }
          }
          frame "EYE_RAW_T", "EYE_T" {
            n183 = global read "G_LCM.vi" "EYE_RAW_T"() -> (w290:T24)
            n184 = global write "G_LCM.vi" "Mobileye name"("Mobileye" ("Mobileye name")) -> ()
            n185 = Unbundle By Name(w290) -> ("hash"=w288:i64)
            n186 = Unflatten From String(type=w290, binary string=w286, data includes array or string size? (T)=FALSE) -> (value=w289:T24, error out=w287:errorcluster)  [unwired: 2 in, 1 out]
            n187 = case shown="No Error" w287 {
              tunnel: w289 -> [w293 _]
              tunnel: w288 -> [w292 _]
              frame No Error {
                n188 = Bundle By Name(cluster=w293, "hash"=w292) -> (w294:T24)
                n189 = global write "G_LCM.vi" "EYE_RAW_T"(w294) -> ()
              }
              frame Error {
              }
            }
          }
          frame "CAN_EYE_RAW_T" {
            n190 = global write "G_LCM.vi" "Mobileye name"("Mobileye" ("Mobileye name")) -> ()
            n191 = global read "G_LCM.vi" "CAN_EYE_RAW_T"() -> (w300:T25)
            n192 = Unbundle By Name(w300) -> ("hash"=w298:i64)
            n193 = Unflatten From String(type=w300, binary string=w296, data includes array or string size? (T)=FALSE) -> (value=w299:T25, error out=w297:errorcluster)  [unwired: 2 in, 1 out]
            n194 = case shown="Error" w297 {
              tunnel: w299 -> [w303 _]
              tunnel: w298 -> [w302 _]
              frame No Error {
                n195 = Bundle By Name(cluster=w303, "hash"=w302) -> (w304:T25)
                n196 = global write "G_LCM.vi" "CAN_EYE_RAW_T"(w304) -> ()
              }
              frame Error {
              }
            }
          }
          frame "CAN_CAR_RAW_T" {
            n197 = global read "G_LCM.vi" "CAN_CAR_RAW_T"() -> (w308:T26)
            n198 = Unbundle By Name(w308) -> ("hash"=w306:i64)
            n199 = Unflatten From String(type=w308, binary string=w309, data includes array or string size? (T)=FALSE) -> (value=w307:T26, error out=w305:errorcluster)  [unwired: 2 in, 1 out]
            n200 = case shown="No Error" w305 {
              tunnel: w307 -> [w312 _]
              tunnel: w306 -> [w311 _]
              frame No Error {
                n201 = Bundle By Name(cluster=w312, "hash"=w311) -> (w313:T26)
                n202 = global write "G_LCM.vi" "CAN_CAR_RAW_T"(w313) -> ()
              }
              frame Error {
              }
            }
          }
          frame "False", Default {
          }
          frame "IBEO_2202_T" {
            n203 = global read "G_LCM.vi" "IBEO_2202_T"() -> (w314:T7)
            n204 = Unbundle By Name(w314) -> ("hash"=w323:i64)
            n205 = Unbundle(w314) -> ("hash"=w320:i64, "sys time"=w321:i64, "Header"=w319:T8, "Scan header"=w318:T27, "Scan points"=w315:T28)
            n206 = Bundle("hash"=w320, "sys time"=w321, "Header"=w319, "Scan header"=w318) -> (w317:T29)  [unwired: 1 in]
            n207 = Unflatten From String(type=w317, binary string=w325, data includes array or string size? (T)=FALSE) -> (rest of the binary string=w316:string, value=w324:T29, error out=w322:errorcluster)  [unwired: 2 in]
            n208 = case shown="No Error" w322 {
              tunnel: w324 -> [w335 _]
              tunnel: w323 -> [w334 _]
              tunnel: w316 -> [w340 _]
              tunnel: w315 -> [w339 _]
              tunnel: w314 -> [w336 _]
              frame No Error {
                n209 = Unbundle By Name(w335) -> ("Header.Size of this messages"=w341:u32)
                n210 = Index Array(array=w339, index=0) -> (element=w337:T30)
                n211 = for {
                  N: w341 -> [_]
                  shift-right: [w344] -> _
                  shift-left: w340 -> [w346]
                  tunnel: w337 -> [w345]
                  tunnel: [w343] -> w330 mode=indexing
                  tunnel: [w342] -> _
                  n212 = Unflatten From String(type=w345, binary string=w346, data includes array or string size? (T)=FALSE) -> (rest of the binary string=w344:string, value=w343:T30, error out=w342:errorcluster)  [unwired: 2 in]
                }
                n213 = Unbundle(w335) -> ("sys time"=w333:i64, "Header"=w332:T8, "Scan header"=w331:T27)  [unwired: 1 out]
                n214 = global read "G_LCM.vi" "queue ibeo"() -> (w329:refnum<queue>)
                n215 = Bundle(cluster=w336, "hash"=w334, "sys time"=w333, "Header"=w332, "Scan header"=w331, "Scan points"=w330) -> (w327:T7)
                n216 = global write "G_LCM.vi" "IBEO_2202_T"(w327) -> ()
                n217 = Lossy Enqueue Element(queue=w329, element=w327) -> (overflow?=→"ibeo overflow?":bool)  [unwired: 1 in, 3 out]
              }
              frame Error {
              }
            }
          }
          frame "VELO_PT_T" {
            n218 = global read "G_LCM.vi" "VELO_PT_T"() -> (w349:T31)
            n219 = Unflatten From String(type=w349, binary string=w352, data includes array or string size? (T)=FALSE) -> (value=w350:T31, error out=w348:errorcluster)  [unwired: 2 in, 1 out]
            n220 = case shown="No Error" w348 {
              tunnel: w350 -> [w353 _]
              frame No Error {
                n221 = call "velosterstack.vi"("VELO_PT_T"=w353) -> ()  [unwired: 10 in, 1 out]
              }
              frame Error {
              }
            }
          }
          frame "VELO_384 " {
            n222 = global read "G_LCM.vi" "VELO_384"() -> (w355:T11)
            n223 = Unflatten From String(type=w355, binary string=w358, data includes array or string size? (T)=FALSE) -> (value=w356:T11, error out=w354:errorcluster)  [unwired: 2 in, 1 out]
            n224 = case shown="No Error" w354 {
              tunnel: w356 -> [w359 _]
              frame No Error {
                n225 = flat-sequence {
                  tunnel: w359 -> [w361]
                  frame #0 {
                    n226 = global read "G_LCM.vi" "queue velo"() -> (w360:refnum<queue>)
                    n227 = Lossy Enqueue Element(queue=w360, element=w361) -> (overflow?=→"velodyne overflow? 2":bool)  [unwired: 1 in, 3 out]
                  }
                }
              }
              frame Error {
              }
            }
          }
          frame "VELO_RAW" {
            n228 = global read "G_LCM.vi" "VELO_RAW"() -> (w365:T1)
            n229 = Unflatten From String(type=w365, binary string=w367, data includes array or string size? (T)=FALSE) -> (value=w363:T1, error out=w364:errorcluster)  [unwired: 2 in, 1 out]
            n230 = case shown="No Error" w364 {
              tunnel: w363 -> [w392 _]
              frame No Error {
                n231 = Unbundle By Name(w392) -> ("raw"=w391:string, "type"=w390:u8)
                n232 = case shown="2" w390 {
                  tunnel: [w423 w424 w425] -> w374
                  frame 0 {
                    w423 = dbl[][] [[0.0, -15.0, 0.0, 0.0, 0.0], [0.0, 1.0, 0.0, 0.0, 0.0], [0.0, -13.0, 0.0, 0.0, 0.0], [0.0, 3.0, 0.0, 0.0, 0.0], [0.0, -11.0, 0.0, 0.0, 0.0], [0.0, 5.0, 0.0, 0.0, 0.0], [0.0, -9.0, 0.0, 0.0, 0.0], [0.0, 7.0, 0.0, 0.0, 0.0], [0.0, -7.0, 0.0, 0.0, 0.0], [0.0, 9.0, 0.0, 0.0, 0.0], [0.0, -5.0, 0.0, 0.0, 0.0], [0.0, 11.0, 0.0, 0.0, 0.0], [0.0, -3.0, 0.0, 0.0, 0.0], [0.0, 13.0, 0.0, 0.0, 0.0], [0.0, -1.0, 0.0, 0.0, 0.0], [0.0, 15.0, 0.0, 0.0, 0.0], [0.0, -15.0, 0.0, 0.0, 0.0], [0.0, 1.0, 0.0, 0.0, 0.0], [0.0, -13.0, 0.0, 0.0, 0.0], [0.0, 3.0, 0.0, 0.0, 0.0], [0.0, -11.0, 0.0, 0.0, 0.0], [0.0, 5.0, 0.0, 0.0, 0.0], [0.0, -9.0, 0.0, 0.0, 0.0], [0.0, 7.0, 0.0, 0.0, 0.0], [0.0, -7.0, 0.0, 0.0, 0.0], [0.0, 9.0, 0.0, 0.0, 0.0], [0.0, -5.0, 0.0, 0.0, 0.0], [0.0, 11.0, 0.0, 0.0, 0.0], [0.0, -3.0, 0.0, 0.0, 0.0], [0.0, 13.0, 0.0, 0.0, 0.0], [0.0, -1.0, 0.0, 0.0, 0.0], [0.0, 15.0, 0.0, 0.0, 0.0], [0.0, 0.0, 0.0, 0.0, 0.0], [0.0, 0.0, 0.0, 0.0, 0.0], [0.0, 0.0, 0.0, 0.0, 0.0], [0.0, 0.0, 0.0, 0.0, 0.0], [0.0, 0.0, 0.0, 0.0, 0.0], [0.0, 0.0, 0.0, 0.0, 0.0], [0.0, 0.0, 0.0, 0.0, 0.0], [0.0, 0.0, 0.0, 0.0, 0.0], [0.0, 0.0, 0.0, 0.0, 0.0], [0.0, 0.0, 0.0, 0.0, 0.0], [0.0, 0.0, 0.0, 0.0, 0.0], [0.0, 0.0, 0.0, 0.0, 0.0], [0.0, 0.0, 0.0, 0.0, 0.0], [0.0, 0.0, 0.0, 0.0, 0.0], [0.0, 0.0, 0.0, 0.0, 0.0], [0.0, 0.0, 0.0, 0.0, 0.0], [0.0, 0.0, 0.0, 0.0, 0.0], [0.0, 0.0, 0.0, 0.0, 0.0], [0.0, 0.0, 0.0, 0.0, 0.0], [0.0, 0.0, 0.0, 0.0, 0.0], [0.0, 0.0, 0.0, 0.0, 0.0], [0.0, 0.0, 0.0, 0.0, 0.0], [0.0, 0.0, 0.0, 0.0, 0.0], [0.0, 0.0, 0.0, 0.0, 0.0], [0.0, 0.0, 0.0, 0.0, 0.0], [0.0, 0.0, 0.0, 0.0, 0.0], [0.0, 0.0, 0.0, 0.0, 0.0], [0.0, 0.0, 0.0, 0.0, 0.0], [0.0, 0.0, 0.0, 0.0, 0.0], [0.0, 0.0, 0.0, 0.0, 0.0], [0.0, 0.0, 0.0, 0.0, 0.0], [0.0, 0.0, 0.0, 0.0, 0.0]]  # Velo 16
                  }
                  frame 1, Default {
                    w424 = dbl[][] [[0.0, -30.67, 0.0, 0.0, 0.0], [0.0, -9.3299999, 0.0, 0.0, 0.0], [0.0, -29.33, 0.0, 0.0, 0.0], [0.0, -8.0, 0.0, 0.0, 0.0], [0.0, -28.0, 0.0, 0.0, 0.0], [0.0, -6.6700001, 0.0, 0.0, 0.0], [0.0, -26.67, 0.0, 0.0, 0.0], [0.0, -5.3299999, 0.0, 0.0, 0.0], [0.0, -25.33, 0.0, 0.0, 0.0], [0.0, -4.0, 0.0, 0.0, 0.0], [0.0, -24.0, 0.0, 0.0, 0.0], [0.0, -2.6700001, 0.0, 0.0, 0.0], [0.0, -22.67, 0.0, 0.0, 0.0], [0.0, -1.33, 0.0, 0.0, 0.0], [0.0, -21.33, 0.0, 0.0, 0.0], [0.0, 0.0, 0.0, 0.0, 0.0], [0.0, -20.0, 0.0, 0.0, 0.0], [0.0, 1.33, 0.0, 0.0, 0.0], [0.0, -18.67, 0.0, 0.0, 0.0], [0.0, 2.6700001, 0.0, 0.0, 0.0], [0.0, -17.33, 0.0, 0.0, 0.0], [0.0, 4.0, 0.0, 0.0, 0.0], [0.0, -16.0, 0.0, 0.0, 0.0], [0.0, 5.3299999, 0.0, 0.0, 0.0], [0.0, -14.67, 0.0, 0.0, 0.0], [0.0, 6.6700001, 0.0, 0.0, 0.0], [0.0, -13.33, 0.0, 0.0, 0.0], [0.0, 8.0, 0.0, 0.0, 0.0], [0.0, -12.0, 0.0, 0.0, 0.0], [0.0, 9.3299999, 0.0, 0.0, 0.0], [0.0, -10.67, 0.0, 0.0, 0.0], [0.0, 10.67, 0.0, 0.0, 0.0], [0.0, 0.0, 0.0, 0.0, 0.0], [0.0, 0.0, 0.0, 0.0, 0.0], [0.0, 0.0, 0.0, 0.0, 0.0], [0.0, 0.0, 0.0, 0.0, 0.0], [0.0, 0.0, 0.0, 0.0, 0.0], [0.0, 0.0, 0.0, 0.0, 0.0], [0.0, 0.0, 0.0, 0.0, 0.0], [0.0, 0.0, 0.0, 0.0, 0.0], [0.0, 0.0, 0.0, 0.0, 0.0], [0.0, 0.0, 0.0, 0.0, 0.0], [0.0, 0.0, 0.0, 0.0, 0.0], [0.0, 0.0, 0.0, 0.0, 0.0], [0.0, 0.0, 0.0, 0.0, 0.0], [0.0, 0.0, 0.0, 0.0, 0.0], [0.0, 0.0, 0.0, 0.0, 0.0], [0.0, 0.0, 0.0, 0.0, 0.0], [0.0, 0.0, 0.0, 0.0, 0.0], [0.0, 0.0, 0.0, 0.0, 0.0], [0.0, 0.0, 0.0, 0.0, 0.0], [0.0, 0.0, 0.0, 0.0, 0.0], [0.0, 0.0, 0.0, 0.0, 0.0], [0.0, 0.0, 0.0, 0.0, 0.0], [0.0, 0.0, 0.0, 0.0, 0.0], [0.0, 0.0, 0.0, 0.0, 0.0], [0.0, 0.0, 0.0, 0.0, 0.0], [0.0, 0.0, 0.0, 0.0, 0.0], [0.0, 0.0, 0.0, 0.0, 0.0], [0.0, 0.0, 0.0, 0.0, 0.0], [0.0, 0.0, 0.0, 0.0, 0.0], [0.0, 0.0, 0.0, 0.0, 0.0], [0.0, 0.0, 0.0, 0.0, 0.0], [0.0, 0.0, 0.0, 0.0, 0.0]]  # Velo_32
                  }
                  frame 2 {
                    w425 = dbl[][] [[-5.3328056, -7.2988362, 111.0, 19.736338, 2.5999999], [-3.2344019, -6.9644198, 146.0, 19.778963, -2.5999999], [2.4376695, 0.250889, 131.76823, 20.688799, 2.5999999], [4.7373252, 0.55538797, 138.12656, 20.727015, -2.5999999], [-1.0502493, -6.6410818, 119.0, 19.82012, 2.5999999], [1.2386309, -6.2594609, 135.0, 19.868624, -2.5999999], [-1.8405367, -8.6656351, 132.0, 19.561426, 2.5999999], [0.4511103, -8.3104696, 145.0, 19.606993, -2.5999999], [3.2611551, -5.9352221, 116.0, 19.909781, 2.5999999], [5.4685535, -5.587399, 133.99889, 19.953875, -2.5999999], [2.4743285, -7.9891219, 117.0, 19.648148, 2.5999999], [4.7189918, -7.644258, 145.0, 19.692244, -2.5999999], [-5.3511744, -3.2475569, 118.71672, 20.249313, 2.5999999], [-3.1158857, -2.850472, 142.90839, 20.29929, -2.5999999], [-6.1270261, -5.204318, 120.0, 20.00238, 2.5999999], [-3.852011, -4.9137921, 137.0, 20.039125, -2.5999999], [-1.1109436, -2.4998751, 101.71324, 20.343384, 2.5999999], [1.1519098, -2.184176, 145.31258, 20.38307, -2.5999999], [-1.8682934, -4.5764661, 130.0, 20.081753, 2.5999999], [0.43604341, -4.2038751, 147.0, 20.128786, -2.5999999], [3.1763444, -1.798143, 115.82812, 20.431576, 2.5999999], [5.4284201, -1.49388, 146.0, 20.469791, -2.5999999], [2.4024715, -1.877563, 129.29713, 20.169943, 2.5999999], [4.6698937, -3.492661, 157.97737, 20.218447, -2.5999999], [-5.3977456, 0.88327599, 124.12312, 20.768169, 2.5999999], [-3.1504908, 1.234519, 128.0, 20.812265, -2.5999999], [-6.1759849, -1.177825, 133.0, 20.509478, 2.5999999], [-3.8819003, -0.86169797, 130.0, 20.549164, -2.5999999], [-1.1136208, 1.585669, 131.0, 20.856361, 2.5999999], [1.0969903, 1.925001, 131.0, 20.898987, -2.5999999], [-1.9088749, -0.486963, 138.48773, 20.596197, 2.5999999], [0.36758029, -0.123898, 137.21994, 20.641764, -2.5999999], [-8.3386211, -22.597513, 117.0, 10.828748, 2.5999999], [-4.7629819, -22.397568, 100.0, 10.854152, -2.5999999], [4.1516571, -11.576517, 130.0, 12.142142, 2.5999999], [7.3577185, -10.877901, 102.0, 12.220895, -2.5999999], [-1.2630961, -21.935509, 106.0, 10.912581, 2.5999999], [2.1595552, -21.409546, 91.0, 10.978632, -2.5999999], [-2.6141083, -25.066507, 127.0, 10.508655, 2.5999999], [0.95595688, -24.458101, 95.0, 10.588678, -2.5999999], [5.5369682, -20.777454, 106.0, 11.057385, 2.5999999], [8.9712191, -20.243195, 97.0, 11.123436, -2.5999999], [4.4757471, -23.863358, 115.0, 10.666161, 2.5999999], [7.8848143, -23.352007, 92.0, 10.732212, -2.5999999], [-8.0466499, -16.629311, 135.0, 11.559117, 2.5999999], [-4.595552, -16.230633, 108.0, 11.606115, -2.5999999], [-9.3918352, -19.788239, 135.0, 11.179325, 2.5999999], [-5.9566336, -19.21587, 98.0, 11.249186, -2.5999999], [-1.3779737, -15.754419, 116.0, 11.662004, 2.5999999], [2.0754263, -15.166914, 105.0, 11.730595, -2.5999999], [-2.5654242, -18.828558, 138.0, 11.296184, 2.5999999], [0.87227631, -18.312876, 105.0, 11.358424, -2.5999999], [5.2989287, -14.641928, 123.0, 11.791565, 2.5999999], [8.7970304, -14.048302, 86.0, 11.860156, -2.5999999], [4.1742177, -17.687857, 135.0, 11.433367, 2.5999999], [7.5869775, -17.16544, 92.0, 11.495607, -2.5999999], [-7.8831077, -10.436752, 121.0, 12.270433, 2.5999999], [-4.5919614, -10.085198, 103.0, 12.30981, -2.5999999], [-9.1805763, -13.484814, 146.0, 11.924937, 2.5999999], [-5.7835727, -13.107666, 99.0, 11.968124, -2.5999999], [-1.2335371, -9.5621262, 123.0, 12.368239, 2.5999999], [1.9424959, -9.0374413, 106.0, 12.426669, -2.5999999], [-2.5727935, -12.651329, 134.0, 12.020203, 2.5999999], [0.81118912, -12.115005, 104.0, 12.081173, -2.5999999]]  # Velo_64
                  }
                }
                n233 = for {
                  N: 12 -> [_]
                  shift-right: [w431] -> _
                  shift-left: w391 -> [w484]
                  tunnel: w390 -> [w472]
                  tunnel: [w432] -> w376 mode=concatenating
                  tunnel: [w429] -> w368 mode=concatenating
                  tunnel: w374 -> [w428]
                  i -> [w479]
                  w467 = 96 ("length (rest)")
                  n234 = Equal?(x=w472, y=u8 2) -> (x = y?=w473:bool)
                  n235 = Quotient & Remainder(x=w479, y=2) -> (x-y*floor(x/y)=w476:i32)  [unwired: 1 out]
                  n236 = Select(t=w476, s=w473, f=0) -> (s? t:f=w475:i32)
                  n237 = Multiply(x=32, y=w475) -> (x*y=w452:i32)
                  n238 = Array Subset(array=w428, index (row)=w452, length (row)=32 ("length")) -> (w450:dbl[][])  [unwired: 2 in]
                  n239 = Unflatten From String(type=T13 {"Laser block ID"=0, "Rotational position"=0}, binary string=w484, data includes array or string size? (T)=FALSE, byte order (0:big-endian, network order)=T12."native, host order") -> (rest of the binary string=w468:string, value=w483:T13)  [unwired: 1 in, 1 out]
                  n240 = Unbundle By Name(w483) -> ("Rotational position"=w480:u16)
                  n241 = String Subset(string=w468, offset (0)=w467) -> (substring=w431:string)  [unwired: 1 in]
                  n242 = String Subset(string=w468, length (rest)=w467) -> (substring=w466:string)  [unwired: 1 in]
                  n243 = Unflatten From String(type=u8[] [], binary string=w466, data includes array or string size? (T)=FALSE, byte order (0:big-endian, network order)=T12."native, host order") -> (value=w464:u8[])  [unwired: 1 in, 2 out]
                  n244 = Reshape Array(w464, 32 ("dimension size"), 3 ("dimension size")) -> (w461:u8[][])
                  n245 = Index Array(array=w461, index (col) #1=1 ("disabled index (col)"), index (col) #2=0 ("index (col)"), index (col) #3=2 ("index (col)")) -> (element #1=w459:u8[], element #2=w458:u8[], element #3=w429:u8[])  [unwired: 3 in]
                  n246 = Join Numbers(hi=w459, lo=w458) -> ((hi.lo)=w453:u16[])
                  n247 = To Double Precision Float(number=w480) -> (double precision float=w481:dbl)
                  n248 = To Double Precision Float(number=w453) -> (double precision float=w455:dbl[])
                  n249 = Multiply(x=w481, y=0.01) -> (x*y=w447:dbl)
                  n250 = Index Array(array=w450, index (col) #1=0 ("disabled index (col)"), index (col) #2=4 ("disabled index (col)"), index (col) #3=1 ("index (col)")) -> (element #1=w448:dbl[], element #2=w440:dbl[], element #3=w436:dbl[], element #4=w426:dbl[], element #5=w435:dbl[])  [unwired: 7 in]
                  n251 = Multiply(x=0.2, y=w455) -> (x*y=w427:dbl[])
                  n252 = Subtract(x=w447, y=w448) -> (x-y=w446:dbl[])
                  n253 = Add(x=w426, y=w427) -> (x+y=w434:dbl[])
                  n254 = Divide(x=w440, y=w434) -> (x/y=w441:dbl[])
                  n255 = Inverse Tangent(1:w441) -> (0:w442:dbl[])
                  n256 = Multiply(x=w442, y=180.0) -> (x*y=w444:dbl[])
                  n257 = Divide(x=w444, y=3.141592653589793) -> (x/y=w439:dbl[])
                  n258 = Subtract(x=w446, y=w439) -> (x-y=w438:dbl[])
                  n259 = Build Array(w438, w436, w434, w435) -> (w433:dbl[][])
                  n260 = Transpose 2D Array(2D array=w433) -> (transposed array=w432:dbl[][])
                }
                n261 = Index Array(array=w376, index (col) #1=0 ("disabled index (col)")) -> (element #1=w378:dbl[], element #2=w385:dbl[], element #3=w386:dbl[], element #4=w389:dbl[])  [unwired: 7 in]
                n262 = Multiply(x=3.141592653589793, y=w378) -> (x*y=w380:dbl[])
                n263 = Multiply(x=3.141592653589793, y=w385) -> (x*y=w383:dbl[])
                n264 = Multiply(x=w389, y=0.01) -> (x*y=w369:dbl[])
                n265 = Divide(x=w380, y=180.0) -> (x/y=w372:dbl[])
                n266 = Divide(x=w383, y=180.0) -> (x/y=w371:dbl[])
                n267 = Multiply(x=w386, y=0.01) -> (x*y=w370:dbl[])
                n268 = disable-structure shown="Enabled" {
                  disable-tunnel: [w405 w406] -> w375
                  disable-tunnel: w372 -> [w404 w415]
                  disable-tunnel: w371 -> [w403 w414]
                  disable-tunnel: w370 -> [w402 w408]
                  disable-tunnel: w369 -> [w401 w413]
                  disable-tunnel: w368 -> [w400 w407]
                  frame Enabled {
                    n269 = global read "G_LCM.vi" "POS_T"() -> (w397:T32)
                    n270 = Unbundle By Name(w397) -> ("y"=w396:dbl, "x"=w395:dbl, "heading"=w394:dbl)
                    n271 = Bundle By Name(cluster=T11 {"hash"=-1208058655852198207, "sys time"=0, "Timestamp"=0, "Rot_ang"=[], "Ver_ang"=[], "Dist"=[], "Ver_off"=[], "Intensity"=[], "pos x"=0.0, "pos y"=0.0, "Heading"=0.0} ("VELO_384"), "Rot_ang"=w404, "Ver_ang"=w403, "Dist"=w402, "Ver_off"=w401, "Intensity"=w400, "pos x"=w396, "pos y"=w395, "Heading"=w394) -> (w398:T11)
                    n272 = global read "G_LCM.vi" "queue velo"() -> (w399:refnum<queue>)
                    n273 = Enqueue Element(queue=w399, element=w398) -> (error out=w405:errorcluster)  [unwired: 2 in, 2 out]
                  }
                  frame Disabled {
                    n274 = Sine & Cosine(0:w415) -> (1:w417:dbl[], 2:w418:dbl[])
                    n275 = Sine & Cosine(0:w414) -> (1:w419:dbl[], 2:w416:dbl[])
                    n276 = Compound Arithmetic op=MULTIPLY(w408, w418, w416) -> (w411:dbl[])
                    n277 = Compound Arithmetic op=MULTIPLY(w417, w416, w408) -> (w412:dbl[])
                    n278 = Compound Arithmetic op=MULTIPLY(w419, w408) -> (w420:dbl[])
                    n279 = global read "G_SEN.vi" "velo_decode"() -> (w421:T33)
                    n280 = Add(x=w420, y=w413) -> (x+y=w410:dbl[])
                    n281 = global read "G_SEN.vi" "queue velo decode"() -> (w422:refnum<queue>)
                    n282 = Bundle By Name(cluster=w421, "i"=w407, "X"=w412, "Y"=w411, "Z"=w410, "d"=w408) -> (w409:T33)
                    n283 = Enqueue Element(queue=w422, element=w409) -> (error out=w406:errorcluster)  [unwired: 2 in, 2 out]
                  }
                }
                "error out 3" <- w375
              }
              frame Error {
              }
            }
          }
          frame "POS_T" {
            n284 = global read "G_LCM.vi" "POS_T"() -> (w491:T32)
            n285 = Unbundle By Name(w491) -> ("hash"=w489:i64)
            n286 = Unflatten From String(type=w491, binary string=w492, data includes array or string size? (T)=FALSE) -> (value=w490:T32, error out=w488:errorcluster)  [unwired: 2 in, 1 out]
            n287 = case shown="No Error" w488 {
              tunnel: w490 -> [w496 _]
              tunnel: w489 -> [w495 _]
              frame No Error {
                n288 = Bundle By Name(cluster=w496, "hash"=w495) -> (w494:T32)
                n289 = global write "G_LCM.vi" "POS_T"(w494) -> ()
              }
              frame Error {
              }
            }
          }
          frame "SLAM" {
            n290 = global read "G_LCM.vi" "SLAM"() -> (w500:T32)
            n291 = Unbundle By Name(w500) -> ("hash"=w498:i64)
            n292 = Unflatten From String(type=w500, binary string=w501, data includes array or string size? (T)=FALSE) -> (value=w499:T32, error out=w497:errorcluster)  [unwired: 2 in, 1 out]
            n293 = case shown="No Error" w497 {
              tunnel: w499 -> [w505 _]
              tunnel: w498 -> [w504 _]
              frame No Error {
                n294 = Bundle By Name(cluster=w505, "hash"=w504) -> (w503:T32)
                n295 = global write "G_LCM.vi" "SLAM"(w503) -> ()
              }
              frame Error {
              }
            }
          }
          frame "LANE_T" {
            n296 = Unflatten From String(type=cluster{"hash":i64, "sys time":i64, "n":i32} {"hash"=-8920902524919788889, "sys time"=0, "n"=0} ("LANE_T"), binary string=w513, data includes array or string size? (T)=FALSE) -> (rest of the binary string=w511:string, value=w514:cluster{"hash":i64, "sys time":i64, "n":i32}, error out=w508:errorcluster)  [unwired: 2 in]
            n297 = Unflatten From String(type=dbl[] [] ("data 2"), binary string=w511, data includes array or string size? (T)=FALSE, error in (no error)=w508) -> (value=w506:dbl[], error out=w507:errorcluster)  [unwired: 1 in, 1 out]
            n298 = case shown="No Error" w507 {
              tunnel: w514 -> [w529 _]
              tunnel: w506 -> [w526 _]
              frame No Error {
                n299 = Unbundle By Name(w529) -> ("sys time"=w528:i64, "n"=w520:i32)
                n300 = Delete From Array(array=w526, length=w520, index=0) -> (deleted portion=w524:dbl[], array with subset deleted=w522:dbl[])
                n301 = Delete From Array(array=w522, length=w520, index=0) -> (deleted portion=w521:dbl[], array with subset deleted=w519:dbl[])
                n302 = global read "G_LCM.vi" "LANE_T"() -> (w530:T34)
                n303 = Delete From Array(array=w519, length=w520, index=0) -> (deleted portion=w517:dbl[], array with subset deleted=w516:dbl[])
                n304 = Bundle By Name(cluster=w530, "sys time"=w528, "n"=w520, "lon"=w516, "lat"=w517, "data2"=w521, "data1"=w524) -> (w527:T34)
                n305 = global write "G_LCM.vi" "LANE_T"(w527) -> ()
              }
              frame Error {
              }
            }
          }
          frame "PATH_T" {
            n306 = Unflatten From String(type=T5 {"hash"=-8920902524919788889, "sys time"=3528569500002214, "n"=0, "pathxy"=[15.0, 175.0, 132.0, 243.0, 160.0, 0.0, 0.0, 1.0, 0.0, 0.0, 160.0, 18.0, 230.0, 6.0, 22.0, 255.0, 89.0, 1.0, 34.0, 1.0, 0.0, 0.0, 0.0, 0.0, 0.0, 0.0, 0.0, 0.0, 0.0, 0.0, 0.0, 0.0, 0.0, 0.0, 0.0, 0.0, 0.0, 0.0, 0.0, 0.0, 0.0, 0.0, 0.0, 0.0, 0.0, 0.0, 0.0, 0.0, 0.0, 0.0, 0.0, 0.0, 0.0, 0.0, 0.0, 0.0, 0.0, 0.0, 0.0, 0.0, 0.0, 0.0, 0.0, 0.0, 0.0, 0.0, 0.0, 0.0, 0.0, 0.0, 0.0, 0.0, 0.0, 0.0, 0.0, 0.0, 0.0, 0.0, 0.0, 0.0, 0.0, 0.0, 0.0, 0.0, 0.0, 0.0, 0.0, 0.0, 0.0, 0.0, 0.0, 0.0, 0.0, 0.0, 0.0, 0.0, 0.0, 0.0, 0.0, 0.0, 0.0, 0.0, 0.0, 0.0, 0.0]} ("PATH_T"), binary string=w533, data includes array or string size? (T)=FALSE) -> (value=w534:T5, error out=w531:errorcluster)  [unwired: 2 in, 1 out]
            n307 = case shown="No Error" w531 {
              tunnel: w534 -> [w541 _]
              frame No Error {
                n308 = Unbundle By Name(w541) -> ("sys time"=w539:i64, "pathxy"=w537:dbl[], "n"=w536:u32)
                n309 = global read "G_LCM.vi" "PATH_T"() -> (w540:T5)
                n310 = Bundle By Name(cluster=w540, "sys time"=w539, "pathxy"=w537, "n"=w536) -> (w538:T5)
                n311 = disable-structure shown="Enabled" {
                  disable-tunnel: w538 -> [w542 _]
                  frame Enabled {
                    n312 = global write "G_LCM.vi" "PATH_T"(w542) -> ()
                  }
                  frame Disabled {
                  }
                }
              }
              frame Error {
              }
            }
          }
          frame "ERROR_T" {
            n313 = Unflatten From String(type=T14 {"hash"=-3262420976274766845, "sys time"=0, "n"=0, "error"=[]} ("ERROR_T"), binary string=w545, data includes array or string size? (T)=FALSE) -> (value=w546:T14, error out=w544:errorcluster)  [unwired: 2 in, 1 out]
            n314 = case shown="No Error" w544 {
              tunnel: w546 -> [w553 _]
              frame No Error {
                n315 = Unbundle By Name(w553) -> ("sys time"=w551:i64, "error"=w549:i32[], "n"=w548:i32)
                n316 = global read "G_LCM.vi" "ERROR_T"() -> (w552:T14)
                n317 = Bundle By Name(cluster=w552, "sys time"=w551, "error"=w549, "n"=w548) -> (w550:T14)
                n318 = disable-structure shown="Enabled" {
                  disable-tunnel: w550 -> [w562 _]
                  frame Enabled {
                    n319 = global write "G_LCM.vi" "ERROR_T"(w562) -> ()
                    n320 = Unbundle By Name(w562) -> ("error"=w556:i32[])
                    n321 = global read "G_ALL.vi" "beep"() -> (w561:T35)
                    n322 = Unbundle By Name(w561) -> ("beep"=w560:bool)
                    n323 = Greater?(x=w556, y=10) -> (0:w555:bool[])
                    n324 = Or Array Elements(Boolean array=w555) -> (logical OR=w558:bool)
                    n325 = Not(x=w560) -> (.not. x?=w559:bool)
                    n326 = And(x=w559, y=w558) -> (x .and. y?=w557:bool)
                    n327 = case shown="True" w557 {
                      frame False {
                      }
                      frame True {
                        n328 = global read "G_ALL.vi" "beep"() -> (w563:T35)
                        n329 = Bundle By Name(cluster=w563, "beep"=TRUE ("use system alert? (T)")) -> (w564:T35)
                        n330 = global write "G_ALL.vi" "beep"(w564) -> ()
                      }
                    }
                  }
                  frame Disabled {
                  }
                }
              }
              frame Error {
              }
            }
          }
          frame "FLEA3_CURRENT" {
            n331 = String Length(string=w566) -> (length=→"length":i32)
          }
          frame "GGA_1" {
            n332 = global read "G_LCM.vi" "GGA_1"() -> (w571:T36)
            n333 = Unbundle By Name(w571) -> ("hash"=w569:i64)
            n334 = Unflatten From String(type=w571, binary string=w572, data includes array or string size? (T)=FALSE) -> (value=w570:T36, error out=w568:errorcluster)  [unwired: 2 in, 1 out]
            n335 = case shown="No Error" w568 {
              tunnel: w570 -> [w576 _]
              tunnel: w569 -> [w575 _]
              frame No Error {
                n336 = flat-sequence {
                  tunnel: w576 -> [w579]
                  tunnel: w575 -> [w578]
                  tunnel: [w577] -> w574
                  tunnel: w574 -> [w590]
                  frame #0 {
                    n337 = Bundle By Name(cluster=w579, "hash"=w578) -> (w577:T36)
                    n338 = global write "G_LCM.vi" "GGA_1"(w577) -> ()
                  }
                  frame #1 {
                    n339 = Unbundle By Name(w590) -> ("sys time"=w588:i64, "lat"=w587:dbl, "lon"=w586:dbl)
                    n340 = local read "SDT_GPS_DATA"() -> (w589:T4)
                    n341 = Bundle By Name(cluster=w589, "sys time"=w588, "lat"=w587, "lon"=w586) -> (w584:T4)
                    n342 = Flatten To String(anything=w584, prepend array or string size? (T)=FALSE) -> (data string=w581:string, error out=→"error out":errorcluster)  [unwired: 2 in, 1 out]
                    n343 = global read "G_LCM.vi" "LCM"() -> (w583:T19)
                    n344 = call "LCM_send.vi"("DATA"=w581, "ID"="SDT_GPS_DATA", "LCM"=w583) -> ()  [unwired: 7 in, 2 out]
                  }
                }
              }
              frame Error {
              }
            }
          }
          frame "GGA_2" {
            n345 = global read "G_LCM.vi" "GGA_2"() -> (w594:T36)
            n346 = Unbundle By Name(w594) -> ("hash"=w592:i64)
            n347 = Unflatten From String(type=w594, binary string=w595, data includes array or string size? (T)=FALSE) -> (value=w593:T36, error out=w591:errorcluster)  [unwired: 2 in, 1 out]
            n348 = case shown="No Error" w591 {
              tunnel: w593 -> [w599 _]
              tunnel: w592 -> [w598 _]
              frame No Error {
                n349 = Bundle By Name(cluster=w599, "hash"=w598) -> (w597:T36)
                n350 = global write "G_LCM.vi" "GGA_2"(w597) -> ()
              }
              frame Error {
              }
            }
          }
          frame "APP_GPS_DATA" {
            n351 = global read "G_LCM.vi" "APP_GPS_DATA"() -> (w603:T37)
            n352 = Unbundle By Name(w603) -> ("hash"=w601:i64)
            n353 = Unflatten From String(type=w603, binary string=w604, data includes array or string size? (T)=FALSE) -> (value=w602:T37, error out=w600:errorcluster)  [unwired: 2 in, 1 out]
            n354 = case shown="No Error" w600 {
              tunnel: w602 -> [w608 _]
              tunnel: w601 -> [w607 _]
              frame No Error {
                n355 = Bundle By Name(cluster=w608, "hash"=w607) -> (w606:T37)
                n356 = global write "G_LCM.vi" "APP_GPS_DATA"(w606) -> ()
              }
              frame Error {
              }
            }
          }
          frame "EURECAR_VISION" {
            n357 = Unflatten From String(type=T15 {"hash"=4202194748993759695, "sys time"=0, "status"=0, "TS_num"=0} ("EURECAR_VISION"), binary string=w613, data includes array or string size? (T)=FALSE) -> (rest of the binary string=w609:string, value=w612:T15, error out=w611:errorcluster)  [unwired: 2 in]
            n358 = case shown="No Error" w611 {
              tunnel: w612 -> [w635 _]
              tunnel: w609 -> [w628 _]
              frame No Error {
                n359 = Unbundle By Name(w635) -> ("sys time"=w617:i64, "status"=w616:i32, "TS_num"=w618:i32)
                n360 = Multiply(x=4, y=w618) -> (x*y=w627:i32)
                n361 = String Subset(string=w628, offset (0)=w627) -> (substring=w626:string)  [unwired: 1 in]
                n362 = String Subset(string=w628, offset (0)=0, length (rest)=w627) -> (substring=w632:string)
                n363 = Unflatten From String(type=dbl[] [] ("TS_loc_x"), binary string=w626, data includes array or string size? (T)=FALSE) -> (value=w622:dbl[])  [unwired: 2 in, 2 out]
                n364 = global read "G_LCM.vi" "EURECAR_VISION"() -> (w630:T38)
                n365 = Delete From Array(array=w622, length=w618, index=0) -> (deleted portion=w619:dbl[], array with subset deleted=w620:dbl[])
                n366 = Unflatten From String(type=i32[] [] ("TS_type"), binary string=w632, data includes array or string size? (T)=FALSE) -> (value=w629:i32[])  [unwired: 2 in, 2 out]
                n367 = Bundle By Name(cluster=w630, "sys time"=w617, "status"=w616, "TS_num"=w618, "TS_type"=w629, "TS_loc_y"=w620, "TS_loc_x"=w619) -> (w615:T38)
                n368 = global write "G_LCM.vi" "EURECAR_VISION"(w615) -> ()
              }
              frame Error {
              }
            }
          }
          frame "vision_lane" {
            n369 = global read "G_LCM.vi" "VISION_LANE"() -> (w640:T39)
            n370 = Unbundle By Name(w640) -> ("hash"=w638:i64)
            n371 = Unflatten From String(type=w640, binary string=w636, data includes array or string size? (T)=FALSE) -> (value=w639:T39, error out=w637:errorcluster)  [unwired: 2 in, 1 out]
            n372 = case shown="No Error" w637 {
              tunnel: w639 -> [w644 _]
              tunnel: w638 -> [w643 _]
              frame No Error {
                n373 = Bundle By Name(cluster=w644, "hash"=w643) -> (w642:T39)
                n374 = global write "G_LCM.vi" "VISION_LANE"(w642) -> ()
              }
              frame Error {
              }
            }
          }
          frame "vision_stopline" {
            n375 = global read "G_LCM.vi" "VISION_STOPLINE"() -> (w649:T40)
            n376 = Unbundle By Name(w649) -> ("hash"=w647:i64)
            n377 = Unflatten From String(type=w649, binary string=w645, data includes array or string size? (T)=FALSE) -> (value=w648:T40, error out=w646:errorcluster)  [unwired: 2 in, 1 out]
            n378 = case shown="No Error" w646 {
              tunnel: w648 -> [w653 _]
              tunnel: w647 -> [w652 _]
              frame No Error {
                n379 = Bundle By Name(cluster=w653, "hash"=w652) -> (w651:T40)
                n380 = global write "G_LCM.vi" "VISION_STOPLINE"(w651) -> ()
              }
              frame Error {
              }
            }
          }
          frame "RMC_1" {
            n381 = global read "G_LCM.vi" "RMC_1"() -> (w657:T41)
            n382 = Unbundle By Name(w657) -> ("hash"=w655:i64)
            n383 = Unflatten From String(type=w657, binary string=w658, data includes array or string size? (T)=FALSE) -> (value=w656:T41, error out=w654:errorcluster)  [unwired: 2 in, 1 out]
            n384 = case shown="No Error" w654 {
              tunnel: w656 -> [w662 _]
              tunnel: w655 -> [w661 _]
              frame No Error {
                n385 = Bundle By Name(cluster=w662, "hash"=w661) -> (w660:T41)
                n386 = global write "G_LCM.vi" "RMC_1"(w660) -> ()
              }
              frame Error {
              }
            }
          }
          frame "RMC_2" {
            n387 = global read "G_LCM.vi" "RMC_2"() -> (w666:T41)
            n388 = Unbundle By Name(w666) -> ("hash"=w664:i64)
            n389 = Unflatten From String(type=w666, binary string=w667, data includes array or string size? (T)=FALSE) -> (value=w665:T41, error out=w663:errorcluster)  [unwired: 2 in, 1 out]
            n390 = case shown="No Error" w663 {
              tunnel: w665 -> [w671 _]
              tunnel: w664 -> [w670 _]
              frame No Error {
                n391 = Bundle By Name(cluster=w671, "hash"=w670) -> (w669:T41)
                n392 = global write "G_LCM.vi" "RMC_2"(w669) -> ()
              }
              frame Error {
              }
            }
          }
        }
      }
      n393 = while {
        tunnel: [w719] -> w50
        shift-right: [w717] -> _
        shift-left: FALSE -> [w718]
        stop <- w716 continue-if-true
        n394 = Wait Until Next ms Multiple(millisecond multiple=u32 5000) -> ()  [unwired: 1 out]
        n395 = Select(t="10.152.36.11" ("address"), s=w718, f="192.168.100.1" ("address")) -> (s? t:f=w710:string)
        n396 = TCP Open Connection(address=w710, remote port or service name=u16 12002 ("Sensor Port 2"), timeout ms (60000)=10 ("timeout ms (25000)")) -> (connection ID=w719:refnum<k5>, error out=w716:errorcluster)  [unwired: 2 in]
        n397 = Not(x=w718) -> (.not. x?=w717:bool)
      }
      n398 = case shown="True" "velodyne enable" {
        frame False {
        }
        frame True {
          n399 = UDP Open(9:10 ("timeout ms (25000)"), 11:u16 2368 ("Sensor Port 2")) -> (port=w674:refnum<k16>, 0:w676:errorcluster)  [unwired: 3 in, 1 out]
          n400 = call "UDP_set_receive_buffer.vi"("error in (no error)"=w676, "Receive Buffer Size"=u32 12060, "connection ID"=w674) -> ("error out"=w677:errorcluster, "connection ID out"=w673:refnum<k16>)  [unwired: 6 in]
          n401 = call "UDP_read_receive_buffer.vi"("error in (no error)"=w677, "connection ID"=w673) -> ("error out"=w675:errorcluster, "connection ID out"=w672:refnum<k16>)  [unwired: 5 in, 1 out]
          n402 = while {
            tunnel: [w690] -> w679
            tunnel: w675 -> [w689]
            tunnel: w672 -> [w688]
            stop <- FALSE stop-if-true
            n403 = UDP Read(connection ID=w688, max size (548)=1206 ("bytes to read"), timeout ms (25000)=1000, 8:w689) -> (data out=w683:string, error out=w682:errorcluster, 3:w690:refnum<k16>)  [unwired: 2 out]
            n404 = case shown="No Error" w682 {
              selector: w682 -> [w692 w704]
              tunnel: w683 -> [_ w693]
              tunnel: [w692 w709] -> w686
              frame Error {
                n405 = Wait Until Next ms Multiple(millisecond multiple=u32 10000) -> ()  [unwired: 1 out]
              }
              frame No Error {
                n406 = Get Date/Time In Seconds() -> (seconds since 1Jan1904=w700:timestamp)
                n407 = To Double Precision Float(number=w700) -> (double precision float=w701:dbl)
                n408 = local read "Velodyne1"() -> (w696:T2)
                n409 = Multiply(x=w701, y=1000000.0) -> (x*y=w703:dbl)
                n410 = local read "VELO_RAW"() -> (w694:T1)
                n411 = To Quad Integer(1:w703) -> (0:w699:i64)
                n412 = To Unsigned Byte Integer(number=w696) -> (unsigned 8bit integer=w695:u8)
                n413 = Bundle By Name(cluster=w694, "sys time"=w699, "raw"=w693, "type"=w695) -> (w697:T1)
                n414 = Flatten To String(anything=w697, prepend array or string size? (T)=FALSE, error in (no error)=w704) -> (data string=w708:string, error out=w705:errorcluster)  [unwired: 1 in, 1 out]
                n415 = global read "G_LCM.vi" "LCM"() -> (w706:T19)
                n416 = call "LCM_send.vi"("error in (no error)"=w705, "DATA"=w708, "ID"="VELO_RAW", "LCM"=w706) -> ("error out"=w709:errorcluster)  [unwired: 6 in, 1 out]
              }
            }
            "veodyne error out" <- w686
          }
          n417 = UDP Close(connection ID=w679) -> ()  [unwired: 1 in, 2 out]
        }
      }
      n418 = while {
        tunnel: w50 -> [w743]
        tunnel: [w727] -> w52
        stop <- FALSE stop-if-true
        w739 = u8[] [175, 254, 192, 194] ("value")
        n419 = TCP Read(connection ID=w743, bytes to read=4 ("count (1)"), 9:1000 ("timeout ms (25000)")) -> (connection ID out=w736:refnum<k5>, data out=w735:string, error out=w738:errorcluster)  [unwired: 2 in]
        n420 = Unflatten From String(type=w739, binary string=w735, data includes array or string size? (T)=FALSE, error in (no error)=w738) -> (value=w720:u8[], error out=w737:errorcluster)  [unwired: 1 in, 1 out]
        n421 = Equal?(x=w739, y=w720) -> (x = y?=w721:bool[])
        n422 = Empty Array?(array=w720) -> (empty?=w725:bool)
        n423 = And Array Elements(Boolean array=w721) -> (logical AND=w723:bool)
        n424 = Not(x=w725) -> (.not. x?=w724:bool)
        n425 = case shown="True" w723 {
          tunnel: w736 -> [w798 w820]
          tunnel: [w797 w815] -> w731
          tunnel: w737 -> [w796 w814]
          tunnel: [w795 w805] -> w741
          frame False {
            n426 = TCP Read(connection ID=w798, bytes to read=9999999, error in (no error)=w796, 7:T18."Immediate" ("mode (standard)"), 9:10 ("timeout ms (25000)")) -> (connection ID out=w797:refnum<k5>, error out=w795:errorcluster)  [unwired: 1 out]
          }
          frame True {
            n427 = TCP Read(connection ID=w820, bytes to read=20 ("count (1)"), error in (no error)=w814, 9:10 ("timeout ms (25000)")) -> (connection ID out=w816:refnum<k5>, data out=w808:string, error out=w813:errorcluster)  [unwired: 1 in]
            n428 = Unflatten From String(type=T8 {"Size of prev messages"=20, "Size of this messages"=20, "Reserved"=20, "DeviceID"=20, "Data type"=20, "NTP time"=20} ("Header"), binary string=w808, data includes array or string size? (T)=FALSE, error in (no error)=w813) -> (value=w802:T8, error out=w812:errorcluster)  [unwired: 1 in, 1 out]
            "header" <- w802
            n429 = Unbundle By Name(w802) -> ("Data type"=w807:u16, "Size of this messages"=w804:u32)
            n430 = To Long Integer(number=w804) -> (32bit integer=w803:i32)
            n431 = TCP Read(connection ID=w816, bytes to read=w803, error in (no error)=w812, 9:1000 ("timeout ms (25000)")) -> (connection ID out=w815:refnum<k5>, data out=w809:string, error out=w806:errorcluster)  [unwired: 1 in]
            n432 = case shown="2202" w807 {
              tunnel: w809 -> [_ w837]
              tunnel: w806 -> [_ w836]
              tunnel: [_ w835] -> w805
              frame Default {
              }
              frame 8706 {
                w827 = T42 {"Scan number"=0, "scanner status"=0, "Sync phase offset"=0, "Scan start time NTP"=0, "Scan end time NTP"=0, "Angle ticks per rotation"=0, "Start angle"=0, "End angle"=0, "Scan points"=0, "Mounting position yaw angle "=0, "Mounting position pitch angle"=0, "Mounting position roll angle"=0, "Mounting position x"=0, "Mounting position y"=0, "Mounting position z"=0, "Reserved"=0}  # Scan header
                n433 = String Subset(string=w837, offset (0)=u16 44 ("y")) -> (substring=w828:string)  [unwired: 1 in]
                n434 = String Subset(string=w837, length (rest)=44 ("length (rest)")) -> (substring=w830:string)  [unwired: 1 in]
                n435 = Unflatten From String(type=w827, binary string=w830, data includes array or string size? (T)=FALSE, byte order (0:big-endian, network order)=T12."little-endian", error in (no error)=w836) -> (value=w834:T42, error out=w824:errorcluster)  [unwired: 1 out]
                n436 = Unbundle By Name(w834) -> ("Scan points"=w822:u16, "Angle ticks per rotation"=w825:u16)
                n437 = flat-sequence {
                  tunnel: w834 -> [w873]
                  tunnel: [w872] -> w833
                  frame #0 {
                    w871 = T43 {"Scan number"=0, "scanner status"=0, "Sync phase offset"=0, "Scan start time NTP"=0, "Scan end time NTP"=0, "Angle ticks per rotation"=0, "Start angle"=0.0, "End angle"=0.0, "Scan points"=0, "Mounting position yaw angle "=0.0, "Mounting position pitch angle"=0.0, "Mounting position roll angle"=0.0, "Mounting position x"=0.0, "Mounting position y"=0.0, "Mounting position z"=0.0, "Reserved"=0}  # Scan header
                    n438 = Unbundle(w873) -> ("Scan number"=w870:u16, "scanner status"=w869:u16, "Sync phase offset"=w868:u16, "Scan start time NTP"=w867:u64, "Scan end time NTP"=w866:u64, "Angle ticks per rotation"=w857:u16, "Start angle"=w863:i16, "End angle"=w862:i16, "Scan points"=w864:u16, "Mounting position yaw angle"=w861:i16, "Mounting position pitch angle"=w860:i16, "Mounting position roll angle"=w859:i16, "Mounting position x"=w852:i16, "Mounting position y"=w851:i16, "Mounting position z"=w850:i16, "Reserved"=w842:u16)
                    n439 = Build Array(w863, w862, w861, w860, w859) -> (w858:i16[])
                    n440 = Build Array(w852, w851, w850) -> (w849:i16[])
                    n441 = Divide(x=w858, y=w857) -> (x/y=w865:dbl[])
                    n442 = Multiply(x=w865, y=6.283185307179586) -> (x*y=w841:dbl[])
                    n443 = disable-structure shown="Enabled" {
                      disable-tunnel: w841 -> [w877 _]
                      disable-tunnel: [w876 w881] -> w840
                      disable-tunnel: [w875 w880] -> w839
                      disable-tunnel: [w874 w879] -> w838
                      frame Disabled {
                        n444 = Index Array(array=w877, index #1=2 ("index")) -> (element #1=w876:dbl, element #2=w875:dbl, element #3=w874:dbl)  [unwired: 2 in]
                      }
                      frame Enabled {
                        n445 = global read "G_LCM.vi" "POS_T"() -> (w882:T32)
                        n446 = Unbundle By Name(w882) -> ("y"=w881:dbl, "x"=w880:dbl, "heading"=w879:dbl)
                      }
                    }
                    n447 = Index Array(array=w841, index #1=0 ("index")) -> (element #1=w854:dbl, element #2=w853:dbl)  [unwired: 1 in]
                    n448 = Multiply(x=w849, y=0.01) -> (x*y=w847:dbl[])
                    n449 = Index Array(array=w847, index #1=0 ("index")) -> (element #1=w845:dbl, element #2=w844:dbl, element #3=w843:dbl)  [unwired: 2 in]
                    n450 = Bundle(cluster=w871, "Scan number"=w870, "scanner status"=w869, "Sync phase offset"=w868, "Scan start time NTP"=w867, "Scan end time NTP"=w866, "Angle ticks per rotation"=w857, "Start angle"=w854, "End angle"=w853, "Scan points"=w864, "Mounting position yaw angle"=w840, "Mounting position pitch angle"=w839, "Mounting position roll angle"=w838, "Mounting position x"=w845, "Mounting position y"=w844, "Mounting position z"=w843, "Reserved"=w842) -> (w872:T43)
                  }
                }
                n451 = for {
                  N: w822 -> [_]
                  shift-right: [w919] -> _
                  shift-left: w828 -> [w922]
                  tunnel: w825 -> [w906]
                  shift-right: [w901] -> w821
                  shift-left: w824 -> [w902]
                  tunnel: [w883] -> w832 mode=indexing
                  w913 = T30 {"flags"=0, "Echo"=0, "Radial distance"=0.0, "Horizontal angle"=0.0, "Vertical angle"=0.0, "Echo pulse width"=0, "Reserved"=0}  # Scan point
                  w920 = T44 {"Layer/Echo"=0, "flags"=0, "Horizontal angle"=0, "Radial distance"=0, "Echo pulse width"=0, "Reserved"=0}  # scan point
                  n452 = Unflatten From String(type=w920, binary string=w922, data includes array or string size? (T)=FALSE, byte order (0:big-endian, network order)=T12."little-endian", error in (no error)=w902) -> (rest of the binary string=w919:string, value=w918:T44, error out=w901:errorcluster)
                  n453 = Unbundle(w918) -> ("Layer/Echo"=w908:u8, "flags"=w885:u8, "Horizontal angle"=w907:i16, "Radial distance"=w889:u16, "Echo pulse width"=w896:u16, "Reserved"=w895:u16)
                  n454 = Divide(x=w907, y=w906) -> (x/y=w905:dbl)
                  n455 = Logical Shift(y=i16 4, x=w885) -> (x << y=w887:u8)
                  n456 = Logical Shift(y=i16 4, x=w908) -> (x << y=w916:u8)
                  n457 = Logical Shift(y=i16 -4, x=w887) -> (x << y=w884:u8)
                  n458 = Logical Shift(y=i16 -4, x=w916) -> (x << y=w912:u8)
                  n459 = Multiply(x=0.8, y=w912) -> (x*y=w910:dbl)
                  n460 = Multiply(x=w889, y=0.01) -> (x*y=w898:dbl)
                  n461 = Logical Shift(y=i16 -4, x=w908) -> (x << y=w899:u8)
                  n462 = Subtract(x=w910, y=1.2) -> (x-y=w894:dbl)
                  n463 = Multiply(x=3.141592653589793, y=w894) -> (x*y=w892:dbl)
                  n464 = Multiply(x=w905, y=6.283185307179586) -> (x*y=w897:dbl)
                  n465 = Divide(x=w892, y=180.0) -> (x/y=w890:dbl)
                  n466 = Bundle(cluster=w913, "flags"=w884, "Echo"=w899, "Radial distance"=w898, "Horizontal angle"=w897, "Vertical angle"=w890, "Echo pulse width"=w896, "Reserved"=w895) -> (w883:T30)
                }
                n467 = case shown="No Error" w821 {
                  selector: w821 -> [w923 _]
                  tunnel: w833 -> [w925 _]
                  tunnel: [w950 _] -> w835
                  tunnel: w832 -> [w924 _]
                  frame No Error {
                    n468 = Get Date/Time In Seconds() -> (seconds since 1Jan1904=w948:timestamp)
                    n469 = To Double Precision Float(number=w948) -> (double precision float=w947:dbl)
                    n470 = Multiply(x=w947, y=1000000.0) -> (x*y=w945:dbl)
                    n471 = local read "IBEO_2202_T"() -> (w943:T7)
                    n472 = local read "header"() -> (w949:T8)
                    n473 = To Quad Integer(1:w945) -> (0:w944:i64)
                    n474 = Bundle By Name(cluster=w943, "sys time"=w944, "Header"=w949, "Scan header"=w925, "Scan points"=w924) -> (w942:T7)
                    n475 = Unbundle(w942) -> ("hash"=w936:i64, "sys time"=w935:i64, "Header"=w928:T8, "Scan header"=w934:T27, "Scan points"=w929:T28)
                    n476 = Array Size(array=w929) -> (size(s)=w927:i32)
                    n477 = Bundle By Name(cluster=w928, "Size of this messages"=w927) -> (w926:T8)
                    n478 = for {
                      N: w927 -> [_]
                      tunnel: w929 -> [w951] mode=indexing
                      shift-right: [w952] -> w930
                      shift-left: "" -> [w954]
                      n479 = Flatten To String(anything=w951, prepend array or string size? (T)=FALSE) -> (data string=w953:string)  [unwired: 2 in, 2 out]
                      n480 = Concatenate Strings(w954, w953) -> (w952:string)
                    }
                    n481 = Bundle("hash"=w936, "sys time"=w935, "Header"=w926, "Scan header"=w934) -> (w937:T29)  [unwired: 1 in]
                    n482 = Flatten To String(anything=w937, prepend array or string size? (T)=FALSE, error in (no error)=w923) -> (data string=w931:string, error out=w939:errorcluster)  [unwired: 1 in, 1 out]
                    n483 = Concatenate Strings(w931, w930) -> (w938:string)
                    n484 = global read "G_LCM.vi" "LCM"() -> (w940:T19)
                    n485 = call "LCM_send.vi"("error in (no error)"=w939, "DATA"=w938, "ID"="IBEO_2202_T", "LCM"=w940) -> ("error out"=w950:errorcluster)  [unwired: 6 in, 1 out]
                  }
                  frame Error {
                  }
                }
              }
            }
          }
        }
        "Ibeo error out" <- w741
        n486 = And(x=w723, y=w724) -> (x .and. y?=w722:bool)
        n487 = global write "G_LCM.vi" "ibeo"(w722) -> ()
        n488 = case shown="True" "setdata" {
          tunnel: [w774 w793] -> w730
          tunnel: w731 -> [w774 w793]
          frame False {
          }
          frame True {
            w780 = T12."little-endian" ("byte order (0:big-endian, network order)")
            n489 = Bundle By Name(cluster=T17 {"command id"=16, "Reserved"=0, "parameter idx"=0} ("Header"), "parameter idx"="parameter idx") -> (w789:T17)
            n490 = Build Array("Mouting", i16 0) -> ()  [unwired: 1 out]
            n491 = Flatten To String(anything=w789, prepend array or string size? (T)=FALSE, byte order (0:big-endian, network order)=w780) -> (data string=w779:string)  [unwired: 1 in, 2 out]
            n492 = Flatten To String(anything="Mouting", prepend array or string size? (T)=FALSE, byte order (0:big-endian, network order)=w780) -> (data string=w778:string)  [unwired: 1 in, 2 out]
            n493 = Concatenate Strings(w779, w778) -> (w777:string)
            n494 = String Length(string=w777) -> (length=w786:i32)
            n495 = To Unsigned Long Integer(number=w786) -> (unsigned 32bit integer=w785:u32)
            n496 = Bundle By Name(cluster=T16 {"Magic word"=2952708290, "Size of prev messages"=0, "Size of this messages"=10, "Reserved"=0, "DeviceID"=7, "Data type"=8208, "NTP time"=0} ("Header"), "Size of this messages"=w785) -> (w787:T16)
            n497 = Flatten To String(anything=w787, prepend array or string size? (T)=FALSE) -> (data string=w784:string)  [unwired: 2 in, 2 out]
            n498 = Concatenate Strings(w784, w777) -> (w783:string)
            n499 = TCP Write(connection ID=w793, data in=w783, 9:1000 ("timeout ms (25000)")) -> ()  [unwired: 1 in, 3 out]
          }
        }
        n500 = case shown="True" "get data" {
          tunnel: [w758 w772] -> w728
          tunnel: w730 -> [w758 w772]
          frame False {
          }
          frame True {
            n501 = Bundle By Name(cluster=T17 {"command id"=17, "Reserved"=0, "parameter idx"=0} ("Header"), "parameter idx"="parameter idx 2") -> (w768:T17)
            n502 = Flatten To String(anything=w768, prepend array or string size? (T)=FALSE, byte order (0:big-endian, network order)=T12."little-endian") -> (data string=w760:string)  [unwired: 1 in, 2 out]
            n503 = String Length(string=w760) -> (length=w765:i32)
            n504 = To Unsigned Long Integer(number=w765) -> (unsigned 32bit integer=w764:u32)
            n505 = Bundle By Name(cluster=T16 {"Magic word"=2952708290, "Size of prev messages"=0, "Size of this messages"=10, "Reserved"=0, "DeviceID"=7, "Data type"=8208, "NTP time"=0} ("Header"), "Size of this messages"=w764) -> (w766:T16)
            n506 = Flatten To String(anything=w766, prepend array or string size? (T)=FALSE) -> (data string=w763:string)  [unwired: 2 in, 2 out]
            n507 = Concatenate Strings(w763, w760) -> (w762:string)
            n508 = TCP Write(connection ID=w772, data in=w762, 9:1000 ("timeout ms (25000)")) -> ()  [unwired: 1 in, 3 out]
          }
        }
        n509 = case shown="True" "saveconfig" {
          tunnel: [w744 w756] -> w727
          tunnel: w728 -> [w744 w756]
          frame False {
          }
          frame True {
            n510 = Flatten To String(anything=cluster{"command id":u16, "Reserved":u16} {"command id"=4, "Reserved"=0} ("Header"), prepend array or string size? (T)=FALSE, byte order (0:big-endian, network order)=T12."little-endian") -> (data string=w747:string)  [unwired: 1 in, 2 out]
            n511 = String Length(string=w747) -> (length=w751:i32)
            n512 = To Unsigned Long Integer(number=w751) -> (unsigned 32bit integer=w750:u32)
            n513 = Bundle By Name(cluster=T16 {"Magic word"=2952708290, "Size of prev messages"=0, "Size of this messages"=10, "Reserved"=0, "DeviceID"=7, "Data type"=8208, "NTP time"=0} ("Header"), "Size of this messages"=w750) -> (w752:T16)
            n514 = Flatten To String(anything=w752, prepend array or string size? (T)=FALSE) -> (data string=w749:string)  [unwired: 2 in, 2 out]
            n515 = Concatenate Strings(w749, w747) -> (w748:string)
            n516 = TCP Write(connection ID=w756, data in=w748, 9:1000 ("timeout ms (25000)")) -> ()  [unwired: 1 in, 3 out]
          }
        }
      }
      n517 = Not Equal?(x=refnum<k5> refnum, y=w52) -> (x != y?=w51:bool)
      n518 = case shown="True" w51 {
        tunnel: w52 -> [_ w956]
        frame False {
        }
        frame True {
          n519 = TCP Close Connection(connection ID=w956) -> ()  [unwired: 2 in, 2 out]
        }
      }
    }
  }
  n520 = disable-structure shown="Enabled" {
    frame Disabled {
      n521 = flat-sequence {
        frame #0 {
          n522 = local write "data"(dbl[][] [] ("data")) -> ()
        }
        frame #1 {
          n523 = while {
            tunnel: [w962] -> w959
            stop <- w961 stop-if-true
            n524 = flat-sequence {
              tunnel: [w966] -> w962
              tunnel: [w964] -> w961
              frame #0 {
                n525 = Wait Until Next ms Multiple(millisecond multiple=u32 10000) -> ()  [unwired: 1 out]
              }
              frame #1 {
                n526 = call-poly "VISA Configure Serial Port"("VISA resource name"=refnum<visa-resource-name> "COM7", "baud rate (9600)"=u32 115200) -> ("VISA resource name out"=w966:refnum<visa-resource-name>, "error out"=w965:errorcluster)  [unwired: 7 in, 5 out]
                n527 = case shown="No Error" w965 {
                  tunnel: [TRUE _] -> w964
                  frame No Error {
                  }
                  frame Error {
                  }
                }
              }
            }
          }
          n528 = VISA Flush I/O Buffer(VISA resource name=w959) -> (VISA resource name out=w958:refnum<visa-resource-name>)  [unwired: 2 in, 1 out]
          n529 = while {
            tunnel: w958 -> [w971]
            tunnel: [w972] -> w960
            stop <- FALSE ("Boolean") stop-if-true
            n530 = flat-sequence {
              tunnel: w971 -> [w975]
              tunnel: [w975] -> w970
              tunnel: [w982] -> w972
              tunnel: w970 -> [w981]
              frame #0 {
                n531 = Wait Until Next ms Multiple(millisecond multiple=u32 100) -> ()  [unwired: 1 out]
              }
              frame #1 {
                n532 = property class="Instr"(reference=w981) -> (reference out=w980:refnum<visa-resource-name>, error out=w976:errorcluster, "Serial Settings:Number of Bytes at Serial Port"=w979:u32)  [unwired: 1 in]
                n533 = Greater Or Equal?(x=w979, y=u32 8) -> (x >= y?=w977:bool)
                n534 = case shown="True" w977 {
                  tunnel: [w983 w988] -> w982
                  tunnel: w980 -> [w983 w990]
                  tunnel: w976 -> [_ w985]
                  frame False {
                  }
                  frame True {
                    n535 = VISA Read(VISA resource name=w990, byte count=u32 8, error in (no error)=w985) -> (VISA resource name out=w987:refnum<visa-resource-name>, read buffer=w992:string, error out=w986:errorcluster)  [unwired: 1 out]
                    n536 = Unflatten From String(type=cluster{"time":i32, "alt":sgl} {"time"=0, "alt"=0.0}, binary string=w992, byte order (0:big-endian, network order)=T12."little-endian", error in (no error)=w986) -> (value=w984:cluster{"time":i32, "alt":sgl}, error out=w989:errorcluster)  [unwired: 1 in, 1 out]
                    n537 = case shown="No Error" w989 {
                      tunnel: [w996 w1035] -> w988
                      tunnel: w987 -> [w996 w1036]
                      tunnel: w984 -> [w995 _]
                      frame No Error {
                        n538 = disable-structure shown="Disabled" {
                          disable-tunnel: w995 -> [w1005 w1029]
                          frame Disabled {
                            n539 = call "Elapsed Time"("Time Target (s)"=5.0, "Auto Reset"=TRUE) -> ("Elapsed Time (s)"=w1000:dbl)  [unwired: 10 in, 7 out]
                            n540 = feedback #1(100.0 ("Elapsed Time (s)")) -> (w1001:dbl)
                            n541 = feedback-in #1(w1000) -> ()
                            n542 = Subtract(x=w1000, y=w1001) -> (x-y=w999:dbl)
                            n543 = To Double Precision Float(number=w1005) -> (double precision float=w1004:cluster{"time":dbl, "alt":dbl})
                            n544 = Less Than 0?(x=w999) -> (x < 0?=w998:bool)
                            n545 = case shown="True" w998 {
                              tunnel: w1004 -> [_ w1011]
                              frame False {
                              }
                              frame True {
                                n546 = Cluster To Array(cluster=w1011) -> (array=w1010:dbl[])
                                n547 = local read "data"() -> (w1009:dbl[][])
                                n548 = Build Array (concatenate)(w1009, w1010) -> (w1008:dbl[][])
                                "data" <- w1008
                                n549 = Index Array(array=w1008, index (col)=1 ("disabled index (col)")) -> (element=→"Waveform Graph":dbl[])  [unwired: 1 in]
                              }
                            }
                          }
                          frame Enabled {
                            n550 = Unbundle By Name(w1029) -> ("time"=w1021:i32, "alt"=w1019:sgl)
                            n551 = First Call?() -> (First Call?: T/F=w1013:bool)
                            n552 = To Quad Integer(1:w1021) -> (0:w1020:i64)
                            n553 = case shown="True" w1013 {
                              tunnel: [w1030 w1031] -> w1012
                              frame False {
                                n554 = local read "ALT_T"() -> (w1030:T6)
                              }
                              frame True {
                                n555 = global read "G_LCM.vi" "ALT_T"() -> (w1032:T6)
                                n556 = Unbundle By Name(w1032) -> ("hash"=w1034:i64)
                                n557 = call "hash.vi"("input"=w1034) -> ("output"=w1033:i64)  [unwired: 10 in]
                                n558 = Bundle By Name(cluster=w1032, "hash"=w1033) -> (w1031:T6)
                                "ALT_T" <- w1031
                              }
                            }
                            n559 = To Double Precision Float(number=w1019) -> (double precision float=w1018:dbl)
                            n560 = Get Date/Time In Seconds() -> (seconds since 1Jan1904=w1023:timestamp)
                            n561 = To Double Precision Float(number=w1023) -> (double precision float=w1024:dbl)
                            n562 = Multiply(x=w1024, y=1000000.0) -> (x*y=w1026:dbl)
                            n563 = To Quad Integer(1:w1026) -> (0:w1022:i64)
                            n564 = Bundle By Name(cluster=w1012, "sys time"=w1022, "u time"=w1020, "alt"=w1018) -> (w1017:T6)
                            n565 = Flatten To String(anything=w1017, prepend array or string size? (T)=FALSE) -> (data string=w1015:string, error out=w1014:errorcluster)  [unwired: 2 in, 1 out]
                            n566 = global read "G_LCM.vi" "LCM"() -> (w1028:T19)
                            n567 = call "LCM_send.vi"("error in (no error)"=w1014, "DATA"=w1015, "ID"="ALT_T", "LCM"=w1028) -> ()  [unwired: 6 in, 2 out]
                          }
                        }
                        "value" <- w995
                      }
                      frame Error {
                        n568 = VISA Flush I/O Buffer(VISA resource name=w1036) -> (VISA resource name out=w1035:refnum<visa-resource-name>)  [unwired: 2 in, 1 out]
                      }
                    }
                  }
                }
              }
            }
          }
          n569 = VISA Close(VISA resource name=w960) -> ()  [unwired: 1 in, 1 out]
        }
      }
    }
    frame Enabled {
    }
  }
